vi "User Manual.vi"() -> ()   [LabVIEW 2019]
uses:
  <userlib>/Exaprom PDF/Controls/Page Controls/Page setup.ctl
  <userlib>/Exaprom PDF/Controls/Page Controls/Page size.ctl
  <userlib>/Exaprom PDF/Controls/Page Controls/Page Orientation.ctl
  <userlib>/Exaprom PDF/Controls/Page Controls/Page Layout Custom.ctl
  <userlib>/Exaprom PDF/Controls/Page Controls/Page margins.ctl
  <userlib>/Exaprom PDF/Controls/Font Controls/Font complete cluster.ctl
  <userlib>/Exaprom PDF/Controls/Font Controls/Font size.ctl
  <userlib>/Exaprom PDF/Controls/Font Controls/Font color.ctl
  <userlib>/Exaprom PDF/Controls/Font Controls/Type and encoding.ctl
  <userlib>/Exaprom PDF/Controls/Text Controls/Unicode/Type and run direction.ctl
  <userlib>/Exaprom PDF/Controls/Initialization Controls/Defaut Paragraphe and Line Spacing.ctl
  <userlib>/Exaprom PDF/Controls/Text Controls/Texte alignement.ctl
  <userlib>/Exaprom PDF/Controls/Text Controls/Line spacing.ctl
  <userlib>/Exaprom PDF/Controls/Table Controls/Table properties.ctl
  <userlib>/Exaprom PDF/Controls/Table Controls/Table position.ctl
  <userlib>/Exaprom PDF/Controls/Initialization Controls/PDF Details.ctl
  <userlib>/Exaprom PDF/Controls/Header, Footer and Watermark Controls/Header or Footer  Image cluster.ctl
  <userlib>/Exaprom PDF/Controls/Table Controls/Cell Alignment 20px.ctl
  <userlib>/Exaprom PDF/Controls/Header, Footer and Watermark Controls/Header or Footer  Page # cluster.ctl
  <userlib>/Exaprom PDF/Controls/Header, Footer and Watermark Controls/Page number.ctl
  <userlib>/Exaprom PDF/Controls/Font Controls/Font complete cluster horizontal.ctl
  <userlib>/Exaprom PDF/Controls/Header, Footer and Watermark Controls/Header or Footer Line cluster.ctl
  <userlib>/Exaprom PDF/Controls/Header, Footer and Watermark Controls/Header Footer Line.ctl
  <userlib>/Exaprom PDF/Controls/Header, Footer and Watermark Controls/Header or Footer  Text cluster.ctl
  <userlib>/Exaprom PDF/Controls/Initialization Controls/Captions.ctl
  <userlib>/Exaprom PDF/Controls/Initialization Controls/Image or Table Caption.ctl
  <userlib>/Exaprom PDF/Controls/Initialization Controls/Unit.ctl
  <userlib>/Exaprom PDF/Controls/Text Controls/Text and hyperlink [ ].ctl
  <userlib>/Exaprom PDF/Controls/Text Controls/Text from String of File and hyperlink.ctl
  <userlib>/Exaprom PDF/Controls/Text Controls/Paragraph indentation.ctl
  <userlib>/Exaprom PDF/Controls/Image Controls/Image alignment and position.ctl
  <userlib>/Exaprom PDF/Controls/Image Controls/Image aligment.ctl
  <userlib>/Exaprom PDF/Controls/Image Controls/Image border.ctl
  <userlib>/Exaprom PDF/Controls/Table Controls/Row Predefined borders cluster.ctl
  <userlib>/Exaprom PDF/Controls/Table Controls/Row Predefined borders.ctl
  <userlib>/Exaprom PDF/Controls/Image Controls/Image Scale.ctl
  <userlib>/Exaprom PDF/Controls/Table Controls/Cell Font, type, Alignment and LS V2.ctl
  <userlib>/Exaprom PDF/Controls/Table Controls/Cell Type, Alignment and LS.ctl
  <userlib>/Exaprom PDF/Controls/Table Controls/Text vertical arrangement.ctl
  <userlib>/Exaprom PDF/Controls/Table Controls/Row Back Ground color Datas.ctl
  <userlib>/Exaprom PDF/Controls/Header, Footer and Watermark Controls/Watermark Text Cluster.ctl
  <userlib>/Exaprom PDF/Controls/Header, Footer and Watermark Controls/Watermark Position.ctl
  <userlib>/Exaprom PDF/Controls/Header, Footer and Watermark Controls/Header footer horiz alignment.ctl
  <userlib>/Exaprom PDF/Controls/Header, Footer and Watermark Controls/Watermark Image Cluster.ctl
  <userlib>/Exaprom PDF/Controls/Table Controls/Simplified Table Row Borders [ ].ctl
  <userlib>/Exaprom PDF/Controls/Table Controls/Simplified Table Row Borders.ctl
  <userlib>/Exaprom PDF/Controls/Table Controls/Border and BG Color [ ].ctl
  <userlib>/Exaprom PDF/Controls/Table Controls/Border and BG Color.ctl
  <userlib>/Exaprom PDF/Controls/Table Controls/Cell Border 20 px.ctl
  <userlib>/Exaprom PDF/Controls/Concatenate Controls/PDF file to concatenate.ctl
  <userlib>/Exaprom PDF/Controls/Table Controls/Table Appearance and Font Row [ ].ctl
  <userlib>/Exaprom PDF/Controls/Table Controls/One Row Appearance.ctl
  <userlib>/Exaprom PDF/Controls/Table Controls/Row from to.ctl
  <userlib>/Exaprom PDF/Controls/Table Controls/Cell, Alignment, LS and Font - hide Vmerge.ctl
  <userlib>/Exaprom PDF/Controls/Table Controls/Cell Appearance.ctl
  <userlib>/Exaprom PDF/Controls/Table Controls/Merge Horizontal.ctl
  <userlib>/Exaprom PDF/Controls/Table Controls/Merge Vertical.ctl
  <userlib>/Exaprom PDF/Controls/Initialization Controls/File Permission Parameters.ctl
  <userlib>/Exaprom PDF/Controls/Initialization Controls/At the opening.ctl
  <vilib>/Utility/miscctls.llb/LVPointTypeDef.ctl
  <userlib>/Exaprom PDF/Controls/Header, Footer and Watermark Controls/Header or Footer.ctl
  <userlib>/Exaprom PDF/Controls/Chapter Controls/Chapter.ctl
  <userlib>/Exaprom PDF/Controls/Image Controls/Image Size Block Diagram.ctl
  <userlib>/Exaprom PDF/VIs/Low level/Header, Footer and Watermark Low level/Append Text HF.vi
  <userlib>/Exaprom PDF/VIs/Low level/Header, Footer and Watermark Low level/AppendLine seperator.vi
  <userlib>/Exaprom PDF/VIs/Low level/Header, Footer and Watermark Low level/Append Image HF.vi
  <userlib>/Exaprom PDF/VIs/Low level/Header, Footer and Watermark Low level/Append Page number HF.vi
  <userlib>/Exaprom PDF/VIs/Low level/Header, Footer and Watermark Low level/Append Watermark Image.vi
  <userlib>/Exaprom PDF/VIs/Low level/Header, Footer and Watermark Low level/Append Watermark Text.vi
  <userlib>/Exaprom PDF/VIs/Text/Append Paragraph with Link [ ].vi
  <userlib>/Exaprom PDF/VIs/Text/Append Paragraph.vi
  <userlib>/Exaprom PDF/VIs/Text/Append Phrase.vi
  <userlib>/Exaprom PDF/LV Class/PDF Report Class/PDF Report Class.lvclass
panel:
  out "Tab Control":T1(tab)
  in  "Page Setup":T2={"Page Size"=1, "Orientation"=enum."Portrait", "Custom Size"={"Width"=0.0, "Height"=0.0}, "Margins"={"Left"=1.0, "Right"=1.0, "Top"=1.0, "Bottom"=1.0}} {"Page Size" items=["Custom", "LETTER", "NOTE", "LEGAL", "TABLOID", "EXECUTIVE", "POSTCARD", "A0", "A1", "A2", "A3", "A4", "A5", "A6", "A7", "A8", "A9", "A10", "B0", "B1", "B2", "B3", "B4", "B5", "B6", "B7", "B8", "B9", "B10", "ARCH_E", "ARCH_D", "ARCH_C", "ARCH_B", "ARCH_A", "FLSA", "FLSE", "HALFLETTER", "_11X17", "ID_1", "ID_2", "ID_3", "LEDGER", "CROWN_QUARTO", "LARGE_CROWN_QUARTO", "DEMY_QUARTO", "ROYAL_QUARTO", "CROWN_OCTAVO", "LARGE_CROWN_OCTAVO", "DEMY_OCTAVO", "ROYAL_OCTAVO", "SMALL_PAPERBACK", "PENGUIN_SMALL_PAPERBACK", "PENGUIN_LARGE_PAPERBACK"]}
  in  "Default Paragraph":T7={" Aligment"=enum."JUSTIFY", "Line spacing"=enum."1.0"}
  out "error out":errorcluster
  in  "PDF Details":T10={"Title"="User Manual for Exaprom PDF 2.0", "Author"="Jean-Marc Simard", "Subject"="This example shows how to create a PDF Report with the toolkit Exaprom PDF 2.0.", "Keywords"="", "Creator"="Exaprom PDF 2.0"}
  in  "File or Directory path":path=path "C:/Users/Jean-Marc/Documents/User Manual.pdf"
  out "PDF File Name":path=path "C:/Users/Jean-Marc/Documents/User Manual.pdf"
  in  "Default Font":T11={"Name"="Arial", "Size"=12.0, "Color"=0, "Style"={"Bold"=FALSE, "Italic"=FALSE, "Underline"=FALSE, "Strikeout"=FALSE}, "Type"={"Type&direction"=enum."ASCII", "Embedded"=FALSE, "Encoding"="CP1252"}}
  in  "Captions":T16={"Figure"={"Caption"="Figure ", "Separator"=":  ", "Position"=enum."Below"}, "Table"={"Caption"="Table ", "Separator"=":  ", "Position"=enum."Above"}, "Font"={"Name"="", "Size"=-1.0, "Color"=0, "Style"={"Bold"=FALSE, "Italic"=FALSE, "Underline"=FALSE, "Strikeout"=FALSE}, "Type"={"Type&direction"=enum."Select", "Embedded"=FALSE, "Encoding"=""}}}
  in  "Unit (default = mm)":T18
  in  "Overwrite?":bool=TRUE
  out "Progress":u8(slide) scale=0.0..20.0
  in  "Permissions":T19={"User Password"="", "Owner Password"="", "Printing"=enum."Allow Printing", "Allow Modify Contents"=FALSE, "Allow Copy"=TRUE, "Allow Modify Annotations"=FALSE, "Allow Fill In "=FALSE, "Allow Screen Readers"=FALSE, "Allow Assembly"=FALSE}
  in  "At the opening":T20={"Page"=1, "Show Bookmarks"=TRUE} {"Page" items=["Single Page - Fit Page"=1, "Single Page - Fit Width"=0]}
  in  "Watermark":enum16{"none", "Image", "Text"}(ring)=enum."Text"
  in  "Footer Page #":T21={"Start at page"=3, "Start with #"=1, "Cell Alignment"=6, "Page #"={"Text 1"="!\u0004B\u0004@\u00040\u0004=\u00048\u0004F\u00040\u0004", "Text 2"="8\u00047\u0004", "Text 3"=""}, "Font"={"Name"="Arial Unicode MS", "Size"=10.0, "Color"=0, "Style"={"Bold"=FALSE, "Italic"=FALSE, "Underline"=FALSE, "Strikeout"=FALSE}, "Type"={"Type&direction"=enum."UTF-16", "Embedded"=FALSE, "Encoding"="CP1251"}}}
  in  "Footer Line":T25={"H/F Line"=enum."Horizontal line", "Thickness (point)"=0.75, " Colour"=7171459}
  in  "Header Line":T25={"H/F Line"=enum."Horizontal line", "Thickness (point)"=0.75, " Colour"=7171459}
  in  "Header Text":T27={"Start at page"=3, "Cell Alignment"=5, "Line spacing"=enum."Select", "Text"="Exaprom PDF 2.0 Toolkit for LabVIEW\n(with <a>iTextSharp</a> 4.1.6)", "Font complete"={"Name"="", "Size"=14.0, "Color"=0, "Style"={"Bold"=TRUE, "Italic"=FALSE, "Underline"=FALSE, "Strikeout"=FALSE}, "Type"={"Type&direction"=enum."Select", "Embedded"=FALSE, "Encoding"=""}}, "Link"="http://itextpdf.com/"}
  in  "Footer Text":T27={"Start at page"=3, "Cell Alignment"=4, "Line spacing"=enum."Select", "Text"="This is an example for the fonts (Segoe Script).", "Font complete"={"Name"="Segoe Script", "Size"=8.0, "Color"=16711680, "Style"={"Bold"=TRUE, "Italic"=TRUE, "Underline"=FALSE, "Strikeout"=FALSE}, "Type"={"Type&direction"=enum."Select", "Embedded"=FALSE, "Encoding"=""}}, "Link"="http://www.microsoft.com/typography/fonts/family.aspx?FID=353"}
  in  "Watermark Image":T28={"Image path"=path "C:/Program Files (x86)/National Instruments/LabVIEW 2013/vi.lib/Exaprom PDF/Examples/Images/Logo Exaprom.jpg", "Opacity (%)"=10.0, "Postion"={"Position"=enum."Center (text section)", "X"=0.0, "Y"=0.0}, "Automatic"=TRUE, "Scale(%)"=100.0, "Rotate(°)"=0.0}
  in  "Watermark Text":T30={"Text "="DRAFT", "Opacity (%)"=5.0, "Position"={"Position"=enum."Center (text section)", "X"=0.0, "Y"=0.0}, "Automatic"=TRUE, "Font"={"Font Name"="", "Size"=-1.0, "Color"=0}, "Alignment"=enum."Center", "Rotate(°)"=0.0}
  in  "Footer Image":T32={"Start at page"=3, "Cell Alignment"=5, "Path"=path "C:/Program Files (x86)/National Instruments/LabVIEW 2013/vi.lib/Exaprom PDF/Examples/Images/Logo Exaprom.jpg", "Image (%)"=15.0, "Link"="http://www.exaprom.com/"}
  in  "Text FP1 [ ]":T33=[{"Text"={"Text"="\n\nExaprom PDF 2.0 Toolkit\n\nUser Manual\n\n", "Path"=path "", "Font complete"={"Name"="", "Size"=32.0, "Color"=0, "Style"={"Bold"=TRUE, "Italic"=FALSE, "Underline"=FALSE, "Strikeout"=FALSE}, "Type"={"Type&direction"=enum."ASCII", "Embedded"=FALSE, "Encoding"=""}}}, "Link"={"Hyperlink"="", "Font complete"={"Name"="", "Size"=-1.0, "Color"=255, "Style"={"Bold"=FALSE, "Italic"=TRUE, "Underline"=FALSE, "Strikeout"=FALSE}, "Type"={"Type&direction"=enum."Select", "Embedded"=FALSE, "Encoding"=""}}}, "Paragraphe"={" Aligment"=enum."CENTER", "Line spacing"=enum."Select"}, "Indentation"={"Left"=0.0, "Right"=0.0}}, {"Text"={"Text"="\nPDF Report with iTextSharp 4.1.6\nfor LabVIEW", "Path"=path "", "Font complete"={"Name"="", "Size"=24.0, "Color"=0, "Style"={"Bold"=TRUE, "Italic"=FALSE, "Underline"=FALSE, "Strikeout"=FALSE}, "Type"={"Type&direction"=enum."Select", "Embedded"=FALSE, "Encoding"=""}}}, "Link"={"Hyperlink"="", "Font complete"={"Name"="", "Size"=-1.0, "Color"=255, "Style"={"Bold"=FALSE, "Italic"=TRUE, "Underline"=FALSE, "Strikeout"=FALSE}, "Type"={"Type&direction"=enum."Select", "Embedded"=FALSE, "Encoding"=""}}}, "Paragraphe"={" Aligment"=enum."CENTER", "Line spacing"=enum."Select"}, "Indentation"={"Left"=0.0, "Right"=0.0}}, {"Text"={"Text"="\n\n\n\nby\n\nJean-Marc Simard\n\n\n\nDevember 10, 2013", "Path"=path "", "Font complete"={"Name"="", "Size"=24.0, "Color"=0, "Style"={"Bold"=FALSE, "Italic"=FALSE, "Underline"=FALSE, "Strikeout"=FALSE}, "Type"={"Type&direction"=enum."Select", "Embedded"=FALSE, "Encoding"=""}}}, "Link"={"Hyperlink"="", "Font complete"={"Name"="", "Size"=-1.0, "Color"=255, "Style"={"Bold"=FALSE, "Italic"=TRUE, "Underline"=FALSE, "Strikeout"=FALSE}, "Type"={"Type&direction"=enum."Select", "Embedded"=FALSE, "Encoding"=""}}}, "Paragraphe"={" Aligment"=enum."CENTER", "Line spacing"=enum."Select"}, "Indentation"={"Left"=0.0, "Right"=0.0}}]
  in  "Image FP1":path=path "C:/Program Files/National Instruments/LabVIEW 2009/vi.lib/Exaprom PDF/Examples/Images/Logo Exaprom.jpg"
  in  "TOC Title":string="\nTable of Contents\n\n\n"
  in  "TOC Title Font":T11={"Name"="Arial Unicode MS", "Size"=14.0, "Color"=0, "Style"={"Bold"=TRUE, "Italic"=FALSE, "Underline"=FALSE, "Strikeout"=FALSE}, "Type"={"Type&direction"=enum."ASCII", "Embedded"=FALSE, "Encoding"="CP1252"}}
  in  "TOC Chapter and section Font":T11={"Name"="Arial Unicode MS", "Size"=-1.0, "Color"=0, "Style"={"Bold"=FALSE, "Italic"=FALSE, "Underline"=FALSE, "Strikeout"=FALSE}, "Type"={"Type&direction"=enum."UTF-16", "Embedded"=FALSE, "Encoding"="CP1251"}}
  in  "Text C8":string="\nAlthough this toolkit had not intended to replace a word processor, we have produced this document, as an example, with this PDF toolkit . The VI \"User Manual.vi\" is available in the palette \"Exaprom PDF 2.0\"."
  in  "Texte C2 [ ]":T33=[{"Text"={"Text"="\nI developed this Reports generation toolkit for PDF because I wanted to be able to generate PDF reports, on LabVIEW, without having to buy a license. The choice fell on the open source iTextSharp 4.1.6 library (<a>Mozilla Public License Version 1.1</a>).  I have developed a series of VIs allowing me to generate PDF reports directly without having to purchase a commercial product. The license chosen:\n", "Path"=path "", "Font complete"={"Name"="", "Size"=-1.0, "Color"=0, "Style"={"Bold"=FALSE, "Italic"=FALSE, "Underline"=FALSE, "Strikeout"=FALSE}, "Type"={"Type&direction"=enum."Select", "Embedded"=FALSE, "Encoding"=""}}}, "Link"={"Hyperlink"="http://www.mozilla.org/MPL/MPL-1.1.html", "Font complete"={"Name"="", "Size"=-1.0, "Color"=255, "Style"={"Bold"=FALSE, "Italic"=TRUE, "Underline"=FALSE, "Strikeout"=FALSE}, "Type"={"Type&direction"=enum."Select", "Embedded"=FALSE, "Encoding"=""}}}, "Paragraphe"={" Aligment"=enum."Select", "Line spacing"=enum."Select"}, "Indentation"={"Left"=0.0, "Right"=0.0}}, {"Text"={"Text"="\n\"The <a>BSD (Berkeley software distribution license)</a> allows proprietary use, and for the software released under the license to be incorporated into proprietary products. Works based on the material may be released under a proprietary license or as closed source software.\" \n", "Path"=path "", "Font complete"={"Name"="", "Size"=-1.0, "Color"=0, "Style"={"Bold"=FALSE, "Italic"=FALSE, "Underline"=FALSE, "Strikeout"=FALSE}, "Type"={"Type&direction"=enum."Select", "Embedded"=FALSE, "Encoding"=""}}}, "Link"={"Hyperlink"="http://fr.wikipedia.org/wiki/Licence_BSD", "Font complete"={"Name"="", "Size"=-1.0, "Color"=255, "Style"={"Bold"=FALSE, "Italic"=TRUE, "Underline"=FALSE, "Strikeout"=FALSE}, "Type"={"Type&direction"=enum."Select", "Embedded"=FALSE, "Encoding"=""}}}, "Paragraphe"={" Aligment"=enum."Select", "Line spacing"=enum."Select"}, "Indentation"={"Left"=0.5, "Right"=0.5}}, {"Text"={"Text"="\nRoughly, you do what you want with those VIs.\n\nThe newer version, <a>iTextSharp 5.X</a>, is under Affero General Public License and is not free for activities involving the iText software without disclosing the source code of your own applications.\n\n\n", "Path"=path "", "Font complete"={"Name"="", "Size"=-1.0, "Color"=0, "Style"={"Bold"=FALSE, "Italic"=FALSE, "Underline"=FALSE, "Strikeout"=FALSE}, "Type"={"Type&direction"=enum."Select", "Embedded"=FALSE, "Encoding"=""}}}, "Link"={"Hyperlink"="http://itextpdf.com/terms-of-use/", "Font complete"={"Name"="", "Size"=-1.0, "Color"=255, "Style"={"Bold"=FALSE, "Italic"=TRUE, "Underline"=FALSE, "Strikeout"=FALSE}, "Type"={"Type&direction"=enum."Select", "Embedded"=FALSE, "Encoding"=""}}}, "Paragraphe"={" Aligment"=enum."Select", "Line spacing"=enum."Select"}, "Indentation"={"Left"=0.0, "Right"=0.0}}]
  in  "Texte D2 [ ]":T33=[{"Text"={"Text"="\n\nThe production of a PDF report can be divided into four steps:\n\n     1) Creating a report (PDF file and default parameters)\n     2) Adding header, footer and watermark (all optional)\n     3) Writing of the PDF report which involves the addition of text elements, images (file,\n           control and front panel) and tables;\n     4) The closure of the PDF report.\n\nIn chapter 5, we review the different VI needed to create a PDF report.\n\n", "Path"=path "", "Font complete"={"Name"="", "Size"=-1.0, "Color"=0, "Style"={"Bold"=FALSE, "Italic"=FALSE, "Underline"=FALSE, "Strikeout"=FALSE}, "Type"={"Type&direction"=enum."Select", "Embedded"=FALSE, "Encoding"=""}}}, "Link"={"Hyperlink"="", "Font complete"={"Name"="", "Size"=-1.0, "Color"=255, "Style"={"Bold"=FALSE, "Italic"=TRUE, "Underline"=FALSE, "Strikeout"=FALSE}, "Type"={"Type&direction"=enum."Select", "Embedded"=FALSE, "Encoding"=""}}}, "Paragraphe"={" Aligment"=enum."Select", "Line spacing"=enum."Select"}, "Indentation"={"Left"=0.0, "Right"=0.0}}]
  in  "Text C6":string="After restart LabVIEW, the palette \"Exaprom PDF 2.0\" will appears.\n\n"
  in  "Text C1":string="Introduction"
  in  "Text C3":string="Installation"
  in  "Texte C4 [ ]":T33=[{"Text"={"Text"="\nAfter unzipping \"ExapromPDF2.0.ZIP\", you have a folder and a file:\n\n     1)\tthe folder \"Exaprom PDF\";\n     2)\tand the file \"exaprompdf.mnu\".\n\n\n", "Path"=path "", "Font complete"={"Name"="", "Size"=-1.0, "Color"=0, "Style"={"Bold"=FALSE, "Italic"=FALSE, "Underline"=FALSE, "Strikeout"=FALSE}, "Type"={"Type&direction"=enum."Select", "Embedded"=FALSE, "Encoding"=""}}}, "Link"={"Hyperlink"="", "Font complete"={"Name"="", "Size"=-1.0, "Color"=16777222, "Style"={"Bold"=TRUE, "Italic"=FALSE, "Underline"=FALSE, "Strikeout"=FALSE}, "Type"={"Type&direction"=enum."Select", "Embedded"=FALSE, "Encoding"=""}}}, "Paragraphe"={" Aligment"=enum."LEFT", "Line spacing"=enum."Select"}, "Indentation"={"Left"=0.0, "Right"=0.0}}]
  in  "Text C5":string="\n\nThe folder \"Exaprom PDF\" has to be place in (see figure 2):\n\nC:\\Program Files\\National Instruments\\LabVIEW Version\\vi.lib\\\n\n"
  in  "Text C7":string="\nThe file \"exaprompdf.mnu\" have to be place in (see figure 3):\n\nC:\\Program Files\\National Instruments\\LabVIEW Version\\\n                                                                                     menus\\Categories\\Programming\\"
  in  "Text D1":string="PDF Report (simplified)"
  in  "Texte E2 [ ]":T33=[{"Text"={"Text"="\n\nThe library used to generate PDF reports is iTextSharp. \n\nThis library uses the point  (72 points = 1 inch = 25.4 mm), but you will work with the unit you choose (inch or mm - section 5.4) unless  the unit \"point\" is clearly indicated.  The font is an exception: the unit is the point.\n\nThe origin of the page is the bottom left corner (see the figure below).\n\nThe text box is the page minus the margins (blue rectangle in the figure below).\n\n\n", "Path"=path "", "Font complete"={"Name"="", "Size"=-1.0, "Color"=0, "Style"={"Bold"=FALSE, "Italic"=FALSE, "Underline"=FALSE, "Strikeout"=FALSE}, "Type"={"Type&direction"=enum."Select", "Embedded"=FALSE, "Encoding"=""}}}, "Link"={"Hyperlink"="", "Font complete"={"Name"="", "Size"=-1.0, "Color"=255, "Style"={"Bold"=FALSE, "Italic"=TRUE, "Underline"=FALSE, "Strikeout"=FALSE}, "Type"={"Type&direction"=enum."Select", "Embedded"=FALSE, "Encoding"=""}}}, "Paragraphe"={" Aligment"=enum."Select", "Line spacing"=enum."Select"}, "Indentation"={"Left"=0.0, "Right"=0.0}}]
  in  "Text E1":string="General"
  in  "Text F2":string="The \"Text\" palette "
  in  "Text F1":string="The different palettes"
  in  "Texte F3 [ ]":T33=[{"Text"={"Text"="\n\nYou have access the fonts contained in the directory C: \\ Windows \\ Fonts (you should check the copyrights). In addition, you have the fonts that come automatically with iTextSharp: Courier, Helvetica, Symbol, Times-Roman and ZapfDingbats.\n\nWhen the PDF report was created, we have specified that the Default Font was Arial 12 points (bold, italic, underline and strikeout = F), Type&direction = ASCII and character encoding = CP1252 (Latin alphabet). This information is stored in the LV Class \"PDF Report\". The parameters of the font in all VI of the Text palette are:\n\n           - Name = empty string;\n           - Size = -1;\n           - Bold, Italic, Underline and Strikeout = F;\n           - Type&direction = Select;\n           - E (Embedded) = F;\n           - Encoding = empty string.\n\nWhen the name of the font is left empty, the name of the default font is used.  When the value of the font size is -1 then the default font size is used. When the value of Type&direction is left to Select, the Type&direction of the default font is used. When the value of the Encoding is left empty, the Encoding of the default font is used.\n", "Path"=path "", "Font complete"={"Name"="", "Size"=-1.0, "Color"=0, "Style"={"Bold"=FALSE, "Italic"=FALSE, "Underline"=FALSE, "Strikeout"=FALSE}, "Type"={"Type&direction"=enum."Select", "Embedded"=FALSE, "Encoding"=""}}}, "Link"={"Hyperlink"="", "Font complete"={"Name"="", "Size"=-1.0, "Color"=255, "Style"={"Bold"=FALSE, "Italic"=TRUE, "Underline"=FALSE, "Strikeout"=FALSE}, "Type"={"Type&direction"=enum."Select", "Embedded"=FALSE, "Encoding"=""}}}, "Paragraphe"={" Aligment"=enum."Select", "Line spacing"=enum."Select"}, "Indentation"={"Left"=0.0, "Right"=0.0}}]
  in  "Text F6":string="When the PDF Report was created, we specified that the default alignment was \"JUSTIFY\" and the default line spacing was 1.0. This information is also stored in the LV Class \"PDF Report\". \n\nWhen the alignment is left to \"Select\" than the default alignment is used. When the spacing is left to \"Select\" than the default line spacing is used.\n\n"
  in  "Text F8 [ ]":T33=[{"Text"={"Text"="This tag allows you to insert the image \"Arrow.jpg\" like this <img src=\"Arrow\"/>.  To insert the image \"Logo E.jpg\" with a link <a><img src=\"Logo\"/></a> you should use \"Append Paragraph & Link [ ].vi\".  All these paragraphs are automatically terminated with a line Feed.  \n\n", "Path"=path "", "Font complete"={"Name"="", "Size"=-1.0, "Color"=0, "Style"={"Bold"=FALSE, "Italic"=FALSE, "Underline"=FALSE, "Strikeout"=FALSE}, "Type"={"Type&direction"=enum."Select", "Embedded"=FALSE, "Encoding"=""}}}, "Link"={"Hyperlink"="http://www.exaprom.com/", "Font complete"={"Name"="", "Size"=-1.0, "Color"=255, "Style"={"Bold"=FALSE, "Italic"=TRUE, "Underline"=FALSE, "Strikeout"=FALSE}, "Type"={"Type&direction"=enum."Select", "Embedded"=FALSE, "Encoding"=""}}}, "Paragraphe"={" Aligment"=enum."Select", "Line spacing"=enum."Select"}, "Indentation"={"Left"=0.0, "Right"=0.0}}, {"Text"={"Text"="The third one, \"Append Phrase.vi\" (number \"4\"), adds a phrase but without a line feed and with a left alignment.   In addition, except for \"Append Phrase.vi\", it is possible to have a paragraph indentation (left and right).\n", "Path"=path "", "Font complete"={"Name"="", "Size"=-1.0, "Color"=0, "Style"={"Bold"=FALSE, "Italic"=FALSE, "Underline"=FALSE, "Strikeout"=FALSE}, "Type"={"Type&direction"=enum."Select", "Embedded"=FALSE, "Encoding"=""}}}, "Link"={"Hyperlink"="", "Font complete"={"Name"="", "Size"=-1.0, "Color"=255, "Style"={"Bold"=FALSE, "Italic"=TRUE, "Underline"=FALSE, "Strikeout"=FALSE}, "Type"={"Type&direction"=enum."Select", "Embedded"=FALSE, "Encoding"=""}}}, "Paragraphe"={" Aligment"=enum."Select", "Line spacing"=enum."Select"}, "Indentation"={"Left"=0.0, "Right"=0.0}}]
  in  "Text F7":string="There are three VIs to add text, and they are grouped in the VI \"Append Text polymorphic.vi\" (number \"1\"  in the previous figure). \n\nWith the first, \"Append Paragraph.vi\" (number \"2\"), you can add text as paragraphs and the text is automatically terminated with a line feed.\n\nThe second or \"Append Paragraph & Link [ ]. Vi\" (number \"3\"), adds a sequence of paragraphs with the particularity that it is possible to associate a link (http://www.mywebsite.com/ ou mailto:name@example.com) with the text, placed between the tags < a> </ a>. \n\nFurthermore, it is possible with \"Append Paragraph.vi\" and \"Append Paragraph & Link [ ]. Vi\" to insert images in a paragraph with the tag <img src=\"Image name\"/>.\n"
  in  "Text F5":string="\nThe character encoding can be ASCII or Unicode (UTF-16).  The writing directions (only for Unicode) are:\n\n  - UTF-16 \"UTF-16 characters, left to right writing\";\n  - UTF-16 (default) \"Use the default run direction\";\n  - UTF-16 (LTR) \"Use bidirectional reordering with a left-to-right preferential\n     run direction\";\n  - UTF-16 (RTL) \"Use bidirectional reordering with a right-to-left preferential\n     run direction\".\n\n"
  in  "Text F4":string="The cluster font could be vertical or horizontal.\n"
  in  "Text G4":string="\nThe available choices are:\n1) Absolute (X, Y) in mm;\n2) Left;\n3) Center;\n4) Right;\n5) Left (TextWrap)\n6) Right (TextWrap).\n\"Left (TextWrap)\" means the image is placed left and the text is placed to the right.  \"Right (TextWrap)\" means that the image is placed to the right, and the text is placed to the left. The indentation works only with \"TextWrap\" and it is the horizontal space that we leave between the image and the text. We can also choose to put a border to the image.\n"
  in  "Texte G3 [ ]":T33=[{"Text"={"Text"=" \nThe Image palette has 4 VIs :\n\n         1)\t\"Append Control Image.vi \";\n         2)\t\"Append Front Panel Image.vi\".\n         3)\t\"Append Block Diagram Image.vi \";\n         4)\t\"Append Image File.vi\".\n\nWe have at the following figure the controls for the properties of the image (this image has been added with \"Append Control Image.vi). We can reduce or enlarge the size of the image (Scale percent). If the image is bigger than the text zone (page size minus the margins), the size will be adjusted automatically to fit.", "Path"=path "", "Font complete"={"Name"="", "Size"=-1.0, "Color"=0, "Style"={"Bold"=FALSE, "Italic"=FALSE, "Underline"=FALSE, "Strikeout"=FALSE}, "Type"={"Type&direction"=enum."Select", "Embedded"=FALSE, "Encoding"=""}}}, "Link"={"Hyperlink"="", "Font complete"={"Name"="", "Size"=-1.0, "Color"=255, "Style"={"Bold"=FALSE, "Italic"=TRUE, "Underline"=FALSE, "Strikeout"=FALSE}, "Type"={"Type&direction"=enum."Select", "Embedded"=FALSE, "Encoding"=""}}}, "Paragraphe"={" Aligment"=enum."Select", "Line spacing"=enum."Select"}, "Indentation"={"Left"=0.0, "Right"=0.0}}, {"Text"={"Text"="\nWe can choose the horizontal position of the image, as long as we have not added a caption, because in this case, it is always centered horizontally.", "Path"=path "", "Font complete"={"Name"="", "Size"=-1.0, "Color"=0, "Style"={"Bold"=FALSE, "Italic"=FALSE, "Underline"=FALSE, "Strikeout"=FALSE}, "Type"={"Type&direction"=enum."Select", "Embedded"=FALSE, "Encoding"=""}}}, "Link"={"Hyperlink"="", "Font complete"={"Name"="", "Size"=-1.0, "Color"=255, "Style"={"Bold"=FALSE, "Italic"=TRUE, "Underline"=FALSE, "Strikeout"=FALSE}, "Type"={"Type&direction"=enum."Select", "Embedded"=FALSE, "Encoding"=""}}}, "Paragraphe"={" Aligment"=enum."Select", "Line spacing"=enum."Select"}, "Indentation"={"Left"=0.0, "Right"=0.0}}]
  in  "Texte G2 [ ]":T33=[{"Text"={"Text"="\nImages placed in the PDF can be reduced or enlarged, but it's only a matter of view: they will always occupy the same space in the PDF file.\n", "Path"=path "", "Font complete"={"Name"="", "Size"=-1.0, "Color"=0, "Style"={"Bold"=FALSE, "Italic"=FALSE, "Underline"=FALSE, "Strikeout"=FALSE}, "Type"={"Type&direction"=enum."Select", "Embedded"=FALSE, "Encoding"=""}}}, "Link"={"Hyperlink"="", "Font complete"={"Name"="", "Size"=-1.0, "Color"=255, "Style"={"Bold"=FALSE, "Italic"=TRUE, "Underline"=FALSE, "Strikeout"=FALSE}, "Type"={"Type&direction"=enum."Select", "Embedded"=FALSE, "Encoding"=""}}}, "Paragraphe"={" Aligment"=enum."Select", "Line spacing"=enum."Select"}, "Indentation"={"Left"=0.0, "Right"=0.0}}]
  in  "Text G1":string="The \"Image\" palette"
  in  "Text H3":string="To create a table, there are six variables, including five optional:\n\n               1) Table columnWidht [ ] (optional);\n               2) Repeat Headers Column (optional)\n               3) Column Headers 2D [ ] (optional);\n               4) Row Headers 1D [ ] (optional);\n               5) Text Data 2D [ ] (required);\n               6) Image to Add [ ] (optional).\n\nThe first specifies the width of each column. The second offers the possibility, if the table has more than one page, to repeat the column headers on each new page.   The third is the column headers.  The fourth is the row headers.  The fifth is the text datas while the last one  allows you to insert images in a table cell. It should be noted that a cell can contain either text or an image, but not both.\n\nThe number of columns is defined by the number of columns after \"Column Headers 2D [ ]\", \"Row Headers 1D\" and \"Text Data 2D [ ]\" are concatenated.\n\nIf the variable \"Table columnWidht [ ]\" is not wired, then the width of each column will be identical and equal to the width of the page (minus the margins) divided by the number of columns (Table 2 versus Table 3 at page 21). If the variable  \"Table columnWidht []\" has more elements than the number of columns, only the first elements will be used. If the variable \"Table columnWidht [ ]\" has fewer elements than the number of columns, columns of 25 mm will be added.\n\nIf the total width of the table is larger than the width of the text zone, then the width of each column will be proportionately reduced so that the table width equals the width of the text zone.\n\nLike for images, we can choose the horizontal position if we have not added any caption, because in this case, the table is always centered horizontally.\n"
  in  "Texte H2 [ ]":T33=[{"Text"={"Text"="\nAdding a table is done in two steps: first, create the table with \"Create Table.vi\" and then add the table with \"Append Table.vi\" or \"Append Customized Table.vi\".\n\n", "Path"=path "", "Font complete"={"Name"="", "Size"=-1.0, "Color"=0, "Style"={"Bold"=FALSE, "Italic"=FALSE, "Underline"=FALSE, "Strikeout"=FALSE}, "Type"={"Type&direction"=enum."Select", "Embedded"=FALSE, "Encoding"=""}}}, "Link"={"Hyperlink"="", "Font complete"={"Name"="", "Size"=-1.0, "Color"=255, "Style"={"Bold"=FALSE, "Italic"=TRUE, "Underline"=FALSE, "Strikeout"=FALSE}, "Type"={"Type&direction"=enum."Select", "Embedded"=FALSE, "Encoding"=""}}}, "Paragraphe"={" Aligment"=enum."Select", "Line spacing"=enum."Select"}, "Indentation"={"Left"=0.0, "Right"=0.0}}]
  in  "Text H7 [ ]":T33=[{"Text"={"Text"="The variable \"Costum Borders\", column by column, defines the type of border for each cell. In iTextSharp there are 16 options, ranging from no line to a line on all four sides. We can also define the background color of each cell.\n\nThe variable <img src=\"Row1\"/> is used to format the table, row by row. A value of -2 indicates the penultimate row. For example,  <img src=\"Row2\"/> iindicates that formatting is applied to row 0 to the penultimate row. A value of -1 indicates the last row. For example, <img src=\"Row3\"/> indicates that formatting is applied to the last row.\n\n", "Path"=path "", "Font complete"={"Name"="", "Size"=-1.0, "Color"=0, "Style"={"Bold"=FALSE, "Italic"=FALSE, "Underline"=FALSE, "Strikeout"=FALSE}, "Type"={"Type&direction"=enum."Select", "Embedded"=FALSE, "Encoding"=""}}}, "Link"={"Hyperlink"="", "Font complete"={"Name"="", "Size"=-1.0, "Color"=255, "Style"={"Bold"=FALSE, "Italic"=TRUE, "Underline"=FALSE, "Strikeout"=FALSE}, "Type"={"Type&direction"=enum."Select", "Embedded"=FALSE, "Encoding"=""}}}, "Paragraphe"={" Aligment"=enum."Select", "Line spacing"=enum."Select"}, "Indentation"={"Left"=0.0, "Right"=0.0}}]
  in  "Texte H4 [ ]":T33=[{"Text"={"Text"="\nIf the total width of the table is larger than the width of the text zone, then the width of each column will be proportionately reduced so that the table width equals the width of the text zone.\n\nLike for images, we can choose the horizontal position if we have not added any caption, because in this case, the table is always centered horizontally.\n", "Path"=path "", "Font complete"={"Name"="", "Size"=-1.0, "Color"=0, "Style"={"Bold"=FALSE, "Italic"=FALSE, "Underline"=FALSE, "Strikeout"=FALSE}, "Type"={"Type&direction"=enum."Select", "Embedded"=FALSE, "Encoding"=""}}}, "Link"={"Hyperlink"="", "Font complete"={"Name"="", "Size"=-1.0, "Color"=255, "Style"={"Bold"=FALSE, "Italic"=TRUE, "Underline"=FALSE, "Strikeout"=FALSE}, "Type"={"Type&direction"=enum."Select", "Embedded"=FALSE, "Encoding"=""}}}, "Paragraphe"={" Aligment"=enum."Select", "Line spacing"=enum."Select"}, "Indentation"={"Left"=0.0, "Right"=0.0}}, {"Text"={"Text"="\nThe final table generated with \"Column Headers 2D [ ]\", \"Row Headers 1D [ ]\" and \"Text Data 2D [ ]\" appears at the following figure.\n\n", "Path"=path "", "Font complete"={"Name"="", "Size"=-1.0, "Color"=0, "Style"={"Bold"=FALSE, "Italic"=FALSE, "Underline"=FALSE, "Strikeout"=FALSE}, "Type"={"Type&direction"=enum."Select", "Embedded"=FALSE, "Encoding"=""}}}, "Link"={"Hyperlink"="", "Font complete"={"Name"="", "Size"=-1.0, "Color"=255, "Style"={"Bold"=FALSE, "Italic"=TRUE, "Underline"=FALSE, "Strikeout"=FALSE}, "Type"={"Type&direction"=enum."Select", "Embedded"=FALSE, "Encoding"=""}}}, "Paragraphe"={" Aligment"=enum."Select", "Line spacing"=enum."Select"}, "Indentation"={"Left"=0.0, "Right"=0.0}}]
  in  "Text H8":string="We can also append a table with \"Append Customized Table.vi\". It is not really intuitive, but you have more flexibility like horizontal merging (see table 5).\n\n"
  in  "Text H5":string="When we add the table to the document with \"Append Table.vi\" we have , if we exclude \"PDF Table\", eight variables (all optional):\n               1) Row background color\n               2) Predefined Borders;\n               3) Column Header Format;\n               4) Table properties;\n               5) Caption;\n               6) Row Header Format;\n               7) Datas Format;\n               8) Custom Table Borders.\n\nThe first offer the possibility to add a background color at each X row.  The second offers a choice for types of borders available: predefined and custom. If the custom type is chosen, then it must use the variable \"Custom Table Borders\" to define the borders of table cells.\n\n"
  in  "Text H6":string="The third, the sixth and the seventh are the cell format for the column headers, the row headers and the data respectively."
  in  "Text H1":string="The \"Table\" palette"
  in  "Texte I6 [ ]":T33=[{"Text"={"Text"="\n ix) the opening of the PDF file generated\n\nHow the PDF file will open.\n\n", "Path"=path "", "Font complete"={"Name"="", "Size"=-1.0, "Color"=0, "Style"={"Bold"=FALSE, "Italic"=FALSE, "Underline"=FALSE, "Strikeout"=FALSE}, "Type"={"Type&direction"=enum."Select", "Embedded"=FALSE, "Encoding"=""}}}, "Link"={"Hyperlink"="", "Font complete"={"Name"="", "Size"=-1.0, "Color"=255, "Style"={"Bold"=FALSE, "Italic"=TRUE, "Underline"=FALSE, "Strikeout"=FALSE}, "Type"={"Type&direction"=enum."Select", "Embedded"=FALSE, "Encoding"=""}}}, "Paragraphe"={" Aligment"=enum."Select", "Line spacing"=enum."Select"}, "Indentation"={"Left"=0.0, "Right"=0.0}}, {"Text"={"Text"="b) Closing the PDF report with \"Close PDF.vi\"", "Path"=path "", "Font complete"={"Name"="", "Size"=-1.0, "Color"=0, "Style"={"Bold"=TRUE, "Italic"=FALSE, "Underline"=FALSE, "Strikeout"=FALSE}, "Type"={"Type&direction"=enum."Select", "Embedded"=FALSE, "Encoding"=""}}}, "Link"={"Hyperlink"="", "Font complete"={"Name"="", "Size"=-1.0, "Color"=255, "Style"={"Bold"=FALSE, "Italic"=TRUE, "Underline"=FALSE, "Strikeout"=FALSE}, "Type"={"Type&direction"=enum."Select", "Embedded"=FALSE, "Encoding"=""}}}, "Paragraphe"={" Aligment"=enum."Select", "Line spacing"=enum."Select"}, "Indentation"={"Left"=0.0, "Right"=0.0}}, {"Text"={"Text"="\nThis VI is used to complete the writing of the report PDF. He closes various references needed to write a PDF file, it writes the header, footer and watermark (if needed) and closes the PDF.\n\n", "Path"=path "", "Font complete"={"Name"="", "Size"=-1.0, "Color"=0, "Style"={"Bold"=FALSE, "Italic"=FALSE, "Underline"=FALSE, "Strikeout"=FALSE}, "Type"={"Type&direction"=enum."Select", "Embedded"=FALSE, "Encoding"=""}}}, "Link"={"Hyperlink"="", "Font complete"={"Name"="", "Size"=-1.0, "Color"=255, "Style"={"Bold"=FALSE, "Italic"=TRUE, "Underline"=FALSE, "Strikeout"=FALSE}, "Type"={"Type&direction"=enum."Select", "Embedded"=FALSE, "Encoding"=""}}}, "Paragraphe"={" Aligment"=enum."Select", "Line spacing"=enum."Select"}, "Indentation"={"Left"=0.0, "Right"=0.0}}, {"Text"={"Text"="c) Adding a page break with \"Append New Page.vi\"", "Path"=path "", "Font complete"={"Name"="", "Size"=-1.0, "Color"=0, "Style"={"Bold"=TRUE, "Italic"=FALSE, "Underline"=FALSE, "Strikeout"=FALSE}, "Type"={"Type&direction"=enum."Select", "Embedded"=FALSE, "Encoding"=""}}}, "Link"={"Hyperlink"="", "Font complete"={"Name"="", "Size"=-1.0, "Color"=255, "Style"={"Bold"=FALSE, "Italic"=TRUE, "Underline"=FALSE, "Strikeout"=FALSE}, "Type"={"Type&direction"=enum."Select", "Embedded"=FALSE, "Encoding"=""}}}, "Paragraphe"={" Aligment"=enum."Select", "Line spacing"=enum."Select"}, "Indentation"={"Left"=0.0, "Right"=0.0}}, {"Text"={"Text"="\nThis VI adds a page break in PDF document.\n\n", "Path"=path "", "Font complete"={"Name"="", "Size"=-1.0, "Color"=0, "Style"={"Bold"=FALSE, "Italic"=FALSE, "Underline"=FALSE, "Strikeout"=FALSE}, "Type"={"Type&direction"=enum."Select", "Embedded"=FALSE, "Encoding"=""}}}, "Link"={"Hyperlink"="", "Font complete"={"Name"="", "Size"=-1.0, "Color"=255, "Style"={"Bold"=FALSE, "Italic"=TRUE, "Underline"=FALSE, "Strikeout"=FALSE}, "Type"={"Type&direction"=enum."Select", "Embedded"=FALSE, "Encoding"=""}}}, "Paragraphe"={" Aligment"=enum."Select", "Line spacing"=enum."Select"}, "Indentation"={"Left"=0.0, "Right"=0.0}}, {"Text"={"Text"="d) Adding a section break (new page) by changing the properties of the page with \"Page Set Size.vi\"", "Path"=path "", "Font complete"={"Name"="", "Size"=-1.0, "Color"=0, "Style"={"Bold"=TRUE, "Italic"=FALSE, "Underline"=FALSE, "Strikeout"=FALSE}, "Type"={"Type&direction"=enum."Select", "Embedded"=FALSE, "Encoding"=""}}}, "Link"={"Hyperlink"="", "Font complete"={"Name"="", "Size"=-1.0, "Color"=255, "Style"={"Bold"=FALSE, "Italic"=TRUE, "Underline"=FALSE, "Strikeout"=FALSE}, "Type"={"Type&direction"=enum."Select", "Embedded"=FALSE, "Encoding"=""}}}, "Paragraphe"={" Aligment"=enum."Select", "Line spacing"=enum."Select"}, "Indentation"={"Left"=0.0, "Right"=0.0}}, {"Text"={"Text"="\nThis VI adds a page break in PDF document and can change the properties of the new page. These new properties apply to all new pages as long you will  not use \"Set Page Size.vi.\n\n", "Path"=path "", "Font complete"={"Name"="", "Size"=-1.0, "Color"=0, "Style"={"Bold"=FALSE, "Italic"=FALSE, "Underline"=FALSE, "Strikeout"=FALSE}, "Type"={"Type&direction"=enum."Select", "Embedded"=FALSE, "Encoding"=""}}}, "Link"={"Hyperlink"="", "Font complete"={"Name"="", "Size"=-1.0, "Color"=255, "Style"={"Bold"=FALSE, "Italic"=TRUE, "Underline"=FALSE, "Strikeout"=FALSE}, "Type"={"Type&direction"=enum."Select", "Embedded"=FALSE, "Encoding"=""}}}, "Paragraphe"={" Aligment"=enum."Select", "Line spacing"=enum."Select"}, "Indentation"={"Left"=0.0, "Right"=0.0}}, {"Text"={"Text"="e) Change the default font with \"Set Default Font.vi\"", "Path"=path "", "Font complete"={"Name"="", "Size"=-1.0, "Color"=0, "Style"={"Bold"=TRUE, "Italic"=FALSE, "Underline"=FALSE, "Strikeout"=FALSE}, "Type"={"Type&direction"=enum."Select", "Embedded"=FALSE, "Encoding"=""}}}, "Link"={"Hyperlink"="", "Font complete"={"Name"="", "Size"=-1.0, "Color"=255, "Style"={"Bold"=FALSE, "Italic"=TRUE, "Underline"=FALSE, "Strikeout"=FALSE}, "Type"={"Type&direction"=enum."Select", "Embedded"=FALSE, "Encoding"=""}}}, "Paragraphe"={" Aligment"=enum."Select", "Line spacing"=enum."Select"}, "Indentation"={"Left"=0.0, "Right"=0.0}}, {"Text"={"Text"="\nThis VI changes the default font.\n\n", "Path"=path "", "Font complete"={"Name"="", "Size"=-1.0, "Color"=0, "Style"={"Bold"=FALSE, "Italic"=FALSE, "Underline"=FALSE, "Strikeout"=FALSE}, "Type"={"Type&direction"=enum."Select", "Embedded"=FALSE, "Encoding"=""}}}, "Link"={"Hyperlink"="", "Font complete"={"Name"="", "Size"=-1.0, "Color"=255, "Style"={"Bold"=FALSE, "Italic"=TRUE, "Underline"=FALSE, "Strikeout"=FALSE}, "Type"={"Type&direction"=enum."Select", "Embedded"=FALSE, "Encoding"=""}}}, "Paragraphe"={" Aligment"=enum."Select", "Line spacing"=enum."Select"}, "Indentation"={"Left"=0.0, "Right"=0.0}}, {"Text"={"Text"="f) Printing of the PDF report with \"Print PDF.vi\"\n", "Path"=path "", "Font complete"={"Name"="", "Size"=-1.0, "Color"=0, "Style"={"Bold"=TRUE, "Italic"=FALSE, "Underline"=FALSE, "Strikeout"=FALSE}, "Type"={"Type&direction"=enum."Select", "Embedded"=FALSE, "Encoding"=""}}}, "Link"={"Hyperlink"="", "Font complete"={"Name"="", "Size"=-1.0, "Color"=255, "Style"={"Bold"=FALSE, "Italic"=TRUE, "Underline"=FALSE, "Strikeout"=FALSE}, "Type"={"Type&direction"=enum."Select", "Embedded"=FALSE, "Encoding"=""}}}, "Paragraphe"={" Aligment"=enum."Select", "Line spacing"=enum."Select"}, "Indentation"={"Left"=0.0, "Right"=0.0}}, {"Text"={"Text"="\nThis VI is not based on the iTextSharp library.\n\n", "Path"=path "", "Font complete"={"Name"="", "Size"=-1.0, "Color"=0, "Style"={"Bold"=FALSE, "Italic"=FALSE, "Underline"=FALSE, "Strikeout"=FALSE}, "Type"={"Type&direction"=enum."Select", "Embedded"=FALSE, "Encoding"=""}}}, "Link"={"Hyperlink"="", "Font complete"={"Name"="", "Size"=-1.0, "Color"=255, "Style"={"Bold"=FALSE, "Italic"=TRUE, "Underline"=FALSE, "Strikeout"=FALSE}, "Type"={"Type&direction"=enum."Select", "Embedded"=FALSE, "Encoding"=""}}}, "Paragraphe"={" Aligment"=enum."Select", "Line spacing"=enum."Select"}, "Indentation"={"Left"=0.0, "Right"=0.0}}]
  in  "Texte I4":string="\n\ni) The generic name for captions\n\nYou can specify a generic name for figure captions and tables. If you write in Figure.Caption \"Figure\" and in Figure.Separator \":\" then for each picture (or pictures) that you add a caption, it will be written into the PDF document: \"Figure 1: Caption of Figure 1\", \" Figure 2: Caption of Figure 2\" and so on. The numbering is automatic.\nii) Unit (default = mm)\n\nThe basic unit used throughout the PDF report (mm or inch)\n\niii) File path or directory\n\nIf you only specify the directory, a dialog box will appear when the program runs,  asking for the file name to use.\n\niv) Default Font\n\nThis is the font (name, color, size and style) used in the document when no other font is specified. The font name is a string. The fonts available are those that appear in the directory \"C: \\ Windows \\ Fonts\". If you specify a font that is not available or misspelled, the font \"Helvetica\" will be substituted.\n\nv) The line spacing and text alignment\n \nYou have the choice of line spacing 1.0, 1.5 and 2.0. Text alignment can be: centered, justify, left or right.\n\nvi) Page Setup\n\nYou choose the page size (default or not), orientation and margins. If the chosen format is \"Custom\", then you must specify the width X (mm or inch) and height Y (mm or inch). This format will be used in the document as you will not change the page size.\n\nvii) The metadata of the PDF (PDF Details)\n\nThis is metadata that you see when you look after the properties from the PDF file that you created (File>>Properties and Description tab).\n\n"
  in  "Texte I3 [ ]":T33=[{"Text"={"Text"="a) Creating a new PDF report with \"New PDF.vi\"", "Path"=path "", "Font complete"={"Name"="", "Size"=-1.0, "Color"=0, "Style"={"Bold"=TRUE, "Italic"=FALSE, "Underline"=FALSE, "Strikeout"=FALSE}, "Type"={"Type&direction"=enum."Select", "Embedded"=FALSE, "Encoding"=""}}}, "Link"={"Hyperlink"="", "Font complete"={"Name"="", "Size"=-1.0, "Color"=255, "Style"={"Bold"=FALSE, "Italic"=TRUE, "Underline"=FALSE, "Strikeout"=FALSE}, "Type"={"Type&direction"=enum."Select", "Embedded"=FALSE, "Encoding"=""}}}, "Paragraphe"={" Aligment"=enum."Select", "Line spacing"=enum."Select"}, "Indentation"={"Left"=0.0, "Right"=0.0}}, {"Text"={"Text"="\nThe first step is to create a new PDF report. The variables in the PDF report are:\n\n          i) generic names for captions of figures and tables;\n          ii) the unit used;\n          iii) the directory or file name (full path) to use;\n          iv) the default font of the document;\n          v) the line spacing and the default alignment of the document;\n          vi) the format of the page;\n          vii) the metadata about the PDF file created;\n          viii) the file permissions;\n          ix) the opening of the PDF file generated.\n", "Path"=path "", "Font complete"={"Name"="", "Size"=-1.0, "Color"=0, "Style"={"Bold"=FALSE, "Italic"=FALSE, "Underline"=FALSE, "Strikeout"=FALSE}, "Type"={"Type&direction"=enum."Select", "Embedded"=FALSE, "Encoding"=""}}}, "Link"={"Hyperlink"="", "Font complete"={"Name"="", "Size"=-1.0, "Color"=255, "Style"={"Bold"=FALSE, "Italic"=TRUE, "Underline"=FALSE, "Strikeout"=FALSE}, "Type"={"Type&direction"=enum."Select", "Embedded"=FALSE, "Encoding"=""}}}, "Paragraphe"={" Aligment"=enum."Select", "Line spacing"=enum."Select"}, "Indentation"={"Left"=0.0, "Right"=0.0}}]
  in  "Texte I2 [ ]":T33=[{"Text"={"Text"="\nDocument palette consists of 6 VIs:\n\na)\tNew PDF.vi;\nb)\tClose PDF.vi;\nc)\tAppend New Page.vi;\nd)\tSet Page Size.vi;\ne)\tSet Default Font.vi;\nf)\tPrint PDF.vi.\n", "Path"=path "", "Font complete"={"Name"="", "Size"=-1.0, "Color"=0, "Style"={"Bold"=FALSE, "Italic"=FALSE, "Underline"=FALSE, "Strikeout"=FALSE}, "Type"={"Type&direction"=enum."Select", "Embedded"=FALSE, "Encoding"=""}}}, "Link"={"Hyperlink"="", "Font complete"={"Name"="", "Size"=-1.0, "Color"=255, "Style"={"Bold"=FALSE, "Italic"=TRUE, "Underline"=FALSE, "Strikeout"=FALSE}, "Type"={"Type&direction"=enum."Select", "Embedded"=FALSE, "Encoding"=""}}}, "Paragraphe"={" Aligment"=enum."Select", "Line spacing"=enum."Select"}, "Indentation"={"Left"=0.0, "Right"=0.0}}]
  in  "Texte I5":string="viii) The file permissions\n\nIn the following table, you have the file permissions you can set with an owner password.  The user password is for the opening of the file.\n\n"
  in  "Text I1":string="The \"Document\" palette"
  in  "Texte J2 [ ]":T33=[{"Text"={"Text"="\nThe header, footer and watermark can be added anywhere during the creation of the report because they are written at the end with \"Close PDF.vi\". For reasons of clarity, we put them immediately after the creation of new PDF report.\n\nA header or footer is a table with one row and a maximum of three columns of equal widths. The number of elements added to a header or a footer (text, image or page number) gives the number of columns for the table.\n\nThe total width of the header (or footer) is the text zone (page width minus the left margin and the right margin). The height of the header (or footer) is the margin (top or bottom) minus 10 mm (0.394\"). The header or the footer is centered vertically.\n", "Path"=path "", "Font complete"={"Name"="", "Size"=-1.0, "Color"=0, "Style"={"Bold"=FALSE, "Italic"=FALSE, "Underline"=FALSE, "Strikeout"=FALSE}, "Type"={"Type&direction"=enum."Select", "Embedded"=FALSE, "Encoding"=""}}}, "Link"={"Hyperlink"="", "Font complete"={"Name"="", "Size"=-1.0, "Color"=255, "Style"={"Bold"=FALSE, "Italic"=TRUE, "Underline"=FALSE, "Strikeout"=FALSE}, "Type"={"Type&direction"=enum."Select", "Embedded"=FALSE, "Encoding"=""}}}, "Paragraphe"={" Aligment"=enum."Select", "Line spacing"=enum."Select"}, "Indentation"={"Left"=0.0, "Right"=0.0}}]
  in  "Texte J4 [ ]":T33=[{"Text"={"Text"=" Header", "Path"=path "", "Font complete"={"Name"="", "Size"=-1.0, "Color"=0, "Style"={"Bold"=TRUE, "Italic"=FALSE, "Underline"=FALSE, "Strikeout"=FALSE}, "Type"={"Type&direction"=enum."Select", "Embedded"=FALSE, "Encoding"=""}}}, "Link"={"Hyperlink"="", "Font complete"={"Name"="", "Size"=-1.0, "Color"=255, "Style"={"Bold"=FALSE, "Italic"=TRUE, "Underline"=FALSE, "Strikeout"=FALSE}, "Type"={"Type&direction"=enum."Select", "Embedded"=FALSE, "Encoding"=""}}}, "Paragraphe"={" Aligment"=enum."Select", "Line spacing"=enum."Select"}, "Indentation"={"Left"=0.0, "Right"=0.0}}, {"Text"={"Text"="\nIn the previous figure, we see that we added one block to the header. It follows that we will have a table consisting of a single column. If we look at the controls \"Header Text\", we can see that the variables are as follows:\n    \n    - Start Page;\n    - Text (the text in question: PDF report generation toolkit for LabVIEW...);\n    - Link (hyperlink optional - http://itextpdf.com/);\n    - The vertical and horizontal alignment (\"CENTER-top\" is selected);\n    - The font (Arial, 14 points bold).\n\nMoreover, we can add a horizontal line to separate the header or the footer from the text.\n\n", "Path"=path "", "Font complete"={"Name"="", "Size"=-1.0, "Color"=0, "Style"={"Bold"=FALSE, "Italic"=FALSE, "Underline"=FALSE, "Strikeout"=FALSE}, "Type"={"Type&direction"=enum."Select", "Embedded"=FALSE, "Encoding"=""}}}, "Link"={"Hyperlink"="", "Font complete"={"Name"="", "Size"=-1.0, "Color"=255, "Style"={"Bold"=FALSE, "Italic"=TRUE, "Underline"=FALSE, "Strikeout"=FALSE}, "Type"={"Type&direction"=enum."Select", "Embedded"=FALSE, "Encoding"=""}}}, "Paragraphe"={" Aligment"=enum."Select", "Line spacing"=enum."Select"}, "Indentation"={"Left"=0.0, "Right"=0.0}}]
  in  "Texte J5 [ ]":T33=[{"Text"={"Text"=" \nFooter", "Path"=path "", "Font complete"={"Name"="", "Size"=-1.0, "Color"=0, "Style"={"Bold"=TRUE, "Italic"=FALSE, "Underline"=FALSE, "Strikeout"=FALSE}, "Type"={"Type&direction"=enum."Select", "Embedded"=FALSE, "Encoding"=""}}}, "Link"={"Hyperlink"="", "Font complete"={"Name"="", "Size"=-1.0, "Color"=255, "Style"={"Bold"=FALSE, "Italic"=TRUE, "Underline"=FALSE, "Strikeout"=FALSE}, "Type"={"Type&direction"=enum."Select", "Embedded"=FALSE, "Encoding"=""}}}, "Paragraphe"={" Aligment"=enum."Select", "Line spacing"=enum."Select"}, "Indentation"={"Left"=0.0, "Right"=0.0}}, {"Text"={"Text"="\nWe have added three blocks to the footer. It follows that we will have a table consisting of three columns. The addition of the blocks is done from left to right:\n\n    - the first block, block \"Text\" is located to the left;\n    - the second block, block \"Image\" is located in the center;\n    - the last block, the block \"Page #\" is located right.\n\t\nIn all cases, we need to specify at which page this block begins to appear (and the vertical and horizontal alignment). The hyperlink is always optional. If an image is too large to fit into the space provided, the dimensions are automatically reduced.\n\n", "Path"=path "", "Font complete"={"Name"="", "Size"=-1.0, "Color"=0, "Style"={"Bold"=FALSE, "Italic"=FALSE, "Underline"=FALSE, "Strikeout"=FALSE}, "Type"={"Type&direction"=enum."Select", "Embedded"=FALSE, "Encoding"=""}}}, "Link"={"Hyperlink"="", "Font complete"={"Name"="", "Size"=-1.0, "Color"=255, "Style"={"Bold"=FALSE, "Italic"=TRUE, "Underline"=FALSE, "Strikeout"=FALSE}, "Type"={"Type&direction"=enum."Select", "Embedded"=FALSE, "Encoding"=""}}}, "Paragraphe"={" Aligment"=enum."Select", "Line spacing"=enum."Select"}, "Indentation"={"Left"=0.0, "Right"=0.0}}]
  in  "Texte J6 [ ]":T33=[{"Text"={"Text"=" \nWatermark\n\n", "Path"=path "", "Font complete"={"Name"="", "Size"=-1.0, "Color"=0, "Style"={"Bold"=TRUE, "Italic"=FALSE, "Underline"=FALSE, "Strikeout"=FALSE}, "Type"={"Type&direction"=enum."Select", "Embedded"=FALSE, "Encoding"=""}}}, "Link"={"Hyperlink"="", "Font complete"={"Name"="", "Size"=-1.0, "Color"=255, "Style"={"Bold"=FALSE, "Italic"=TRUE, "Underline"=FALSE, "Strikeout"=FALSE}, "Type"={"Type&direction"=enum."Select", "Embedded"=FALSE, "Encoding"=""}}}, "Paragraphe"={" Aligment"=enum."Select", "Line spacing"=enum."Select"}, "Indentation"={"Left"=0.0, "Right"=0.0}}, {"Text"={"Text"="\nThe first element in the cluster watermark is the cluster name \"General\", it consists of:\n\n    - Type (Text, Text auto and Image);\n    - Opacity (%);\n    - The angle of rotation (Rotate (°))\n    - The position (Absolute, Center on page and Center on text section);\n    - Absolute position (X (mm or inch) and Y (mm or inch)).\n\n\nThe type defines the element that we add (Text, Text auto et Image). In the case of  \" Text auto \", the angle of rotation is automatically calculated so that the text is placed on the diagonal of the area (the whole page or text zone), and the font size is maximized.\n\nBecause the watermark is placed into the foreground, you must specify its opacity. When you select \"Text\" or \"Picture\", we can specify the rotation of the text box or image.\n\nPosition \"Absolute\" applies only to the type \"Text\" or \"Picture\". When this position is selected then the point (0,0) is the lower left corner of the page.\n\n\n", "Path"=path "", "Font complete"={"Name"="", "Size"=-1.0, "Color"=0, "Style"={"Bold"=FALSE, "Italic"=FALSE, "Underline"=FALSE, "Strikeout"=FALSE}, "Type"={"Type&direction"=enum."Select", "Embedded"=FALSE, "Encoding"=""}}}, "Link"={"Hyperlink"="", "Font complete"={"Name"="", "Size"=-1.0, "Color"=255, "Style"={"Bold"=FALSE, "Italic"=TRUE, "Underline"=FALSE, "Strikeout"=FALSE}, "Type"={"Type&direction"=enum."Select", "Embedded"=FALSE, "Encoding"=""}}}, "Paragraphe"={" Aligment"=enum."Select", "Line spacing"=enum."Select"}, "Indentation"={"Left"=0.0, "Right"=0.0}}]
  in  "Texte J3":string="\n\nBlocks of the header or footer are added with \"Header or Footer polymorphic.vi\" and the watermark with \"Append Watermark.vi\".\n"
  in  "TexteJ7":string="\nFor the watermark, it is impossible  to change the style of a font (bold, italic, underline and strikeout) and Watermark supports only ASCII characters.\n\n"
  in  "Text J1":string="The \"Header, Footer and Watermark\" palette"
  in  "Texte K2 [ ]":T33=[{"Text"={"Text"="\n\nYou could append a PDF file in the PDF Report with \"Append PDF files to PDF Report.vi\".  You have to take care if the Report has header or footer because it is added as an exact copy (the footer, and the header could be written over a part of the text you added).  The last page of this manual is added with this VI.  I also include a standalone VI to concatenate PDF files.\n\n", "Path"=path "", "Font complete"={"Name"="", "Size"=-1.0, "Color"=0, "Style"={"Bold"=FALSE, "Italic"=FALSE, "Underline"=FALSE, "Strikeout"=FALSE}, "Type"={"Type&direction"=enum."Select", "Embedded"=FALSE, "Encoding"=""}}}, "Link"={"Hyperlink"="", "Font complete"={"Name"="", "Size"=-1.0, "Color"=255, "Style"={"Bold"=FALSE, "Italic"=TRUE, "Underline"=FALSE, "Strikeout"=FALSE}, "Type"={"Type&direction"=enum."Select", "Embedded"=FALSE, "Encoding"=""}}}, "Paragraphe"={" Aligment"=enum."Select", "Line spacing"=enum."Select"}, "Indentation"={"Left"=0.0, "Right"=0.0}}]
  in  "Texte K3 [ ]":T33=[{"Text"={"Text"="The general syntax for the range that is used looks like this: [!][o][odd][e][even]start-end.   You can have multiple page ranges separated by commas. The ! modifier removes pages from what is already selected. The range changes are incremental—numbers are added or deleted as the range appears. The start or the end can be omitted. If you omit both, you need at least o (odd; selects all odd pages) or e (even; selects all even pages):\n\n", "Path"=path "", "Font complete"={"Name"="", "Size"=-1.0, "Color"=0, "Style"={"Bold"=FALSE, "Italic"=FALSE, "Underline"=FALSE, "Strikeout"=FALSE}, "Type"={"Type&direction"=enum."Select", "Embedded"=FALSE, "Encoding"=""}}}, "Link"={"Hyperlink"="", "Font complete"={"Name"="", "Size"=-1.0, "Color"=255, "Style"={"Bold"=FALSE, "Italic"=TRUE, "Underline"=FALSE, "Strikeout"=FALSE}, "Type"={"Type&direction"=enum."Select", "Embedded"=FALSE, "Encoding"=""}}}, "Paragraphe"={" Aligment"=enum."Select", "Line spacing"=enum."Select"}, "Indentation"={"Left"=0.0, "Right"=0.0}}, {"Text"={"Text"="\"all\" : complete PDF document\n\"o\":  selects all odd pages\n\"e\":  selects all even pages\n\"1-4, 6-8, !7\": selects pages 1, 2, 3,4, 6, and 8 (\"!\" excluded page 7)\n\n\n", "Path"=path "", "Font complete"={"Name"="", "Size"=-1.0, "Color"=0, "Style"={"Bold"=FALSE, "Italic"=FALSE, "Underline"=FALSE, "Strikeout"=FALSE}, "Type"={"Type&direction"=enum."Select", "Embedded"=FALSE, "Encoding"=""}}}, "Link"={"Hyperlink"="", "Font complete"={"Name"="", "Size"=-1.0, "Color"=255, "Style"={"Bold"=FALSE, "Italic"=TRUE, "Underline"=FALSE, "Strikeout"=FALSE}, "Type"={"Type&direction"=enum."Select", "Embedded"=FALSE, "Encoding"=""}}}, "Paragraphe"={" Aligment"=enum."Select", "Line spacing"=enum."Select"}, "Indentation"={"Left"=1.0, "Right"=0.0}}, {"Text"={"Text"="If a PDF file is not protected, then Password = empty string. If the PDF file is protected you need to provide:\n\n", "Path"=path "", "Font complete"={"Name"="", "Size"=-1.0, "Color"=0, "Style"={"Bold"=FALSE, "Italic"=FALSE, "Underline"=FALSE, "Strikeout"=FALSE}, "Type"={"Type&direction"=enum."Select", "Embedded"=FALSE, "Encoding"=""}}}, "Link"={"Hyperlink"="", "Font complete"={"Name"="", "Size"=-1.0, "Color"=255, "Style"={"Bold"=FALSE, "Italic"=TRUE, "Underline"=FALSE, "Strikeout"=FALSE}, "Type"={"Type&direction"=enum."Select", "Embedded"=FALSE, "Encoding"=""}}}, "Paragraphe"={" Aligment"=enum."Select", "Line spacing"=enum."Select"}, "Indentation"={"Left"=0.0, "Right"=0.0}}, {"Text"={"Text"="- the owner password (if protected with a user and an owner password);\n- the owner password (if protected with only an owner password);\n- the user password (if protected with only a user password).\n", "Path"=path "", "Font complete"={"Name"="", "Size"=-1.0, "Color"=0, "Style"={"Bold"=FALSE, "Italic"=FALSE, "Underline"=FALSE, "Strikeout"=FALSE}, "Type"={"Type&direction"=enum."Select", "Embedded"=FALSE, "Encoding"=""}}}, "Link"={"Hyperlink"="", "Font complete"={"Name"="", "Size"=-1.0, "Color"=255, "Style"={"Bold"=FALSE, "Italic"=TRUE, "Underline"=FALSE, "Strikeout"=FALSE}, "Type"={"Type&direction"=enum."Select", "Embedded"=FALSE, "Encoding"=""}}}, "Paragraphe"={" Aligment"=enum."Select", "Line spacing"=enum."Select"}, "Indentation"={"Left"=1.0, "Right"=0.0}}]
  in  "Text k1":string="The \"Concatenate\" palette"
  in  "Text L1":string="The \"Table of Contents\" palette"
  in  "Text L2":string="\nYou could add auto numbering bookmark (Append Chapter bookmark.vi) and you could add a Table of Contents (Append a Table of Contents.vi).\n"
  in  "Text L3":string="\nAppend Chapter bookmark.vi works with UTF-16 characters like you can see in this manual.\n"
  in  "Text L4":string="\nYou could also add a table of contents with \"Append a Table of Contents.vi\".  Bookmarks you set (with \"Append Chapter bookmark.vi\") are then used to generate the table of contents.  If you left click on the text  of the table of content you will jump to the corresponding section for ASCII text, but you will not jump for UTF-16 text.  \n"
  in  "Text M1":string="The \"Tools\" palette"
  in  "Text M2":string="All the VIs in this palette are standalone.\n\nThe first two VIs (\"Read Unicode File.vi\" and \"Get Available Font Encoding [ ].vi\") will be discussed in the next section of the document.\n\nThe third VI \"Change AcroField Value (String).vi\" allows to change the value of an AcroField (string) of a PDF form.\n\nThe fourth VI \"Read AcroFields.vi\" allows to read the list of AcroFields in a PDF form.\n\n\n"
  in  "Texte N4 [ ]":T33=[{"Text"={"Text"="\nYou have access to the characters U+0000 to U+FFFF (what is in the \"Character Map\" of Windows).  I know two methods to write Unicode text in a LabVIEW string:\n\n", "Path"=path "", "Font complete"={"Name"="", "Size"=-1.0, "Color"=0, "Style"={"Bold"=FALSE, "Italic"=FALSE, "Underline"=FALSE, "Strikeout"=FALSE}, "Type"={"Type&direction"=enum."Select", "Embedded"=FALSE, "Encoding"=""}}}, "Link"={"Hyperlink"="", "Font complete"={"Name"="", "Size"=-1.0, "Color"=255, "Style"={"Bold"=FALSE, "Italic"=TRUE, "Underline"=FALSE, "Strikeout"=FALSE}, "Type"={"Type&direction"=enum."Select", "Embedded"=FALSE, "Encoding"=""}}}, "Paragraphe"={" Aligment"=enum."Select", "Line spacing"=enum."Select"}, "Indentation"={"Left"=0.0, "Right"=0.0}}, {"Text"={"Text"="1) enable Unicode support by adding the following setting in the LabVIEW.ini \"UseUnicode=True\" (see \"<a>A List of Tips and Tools for using Unicode in LabVIEW</a>\") and write directly in the string control.\n2) read an Unicode text file and copy it in a string.", "Path"=path "", "Font complete"={"Name"="", "Size"=-1.0, "Color"=0, "Style"={"Bold"=FALSE, "Italic"=FALSE, "Underline"=FALSE, "Strikeout"=FALSE}, "Type"={"Type&direction"=enum."Select", "Embedded"=FALSE, "Encoding"=""}}}, "Link"={"Hyperlink"="https://decibel.ni.com/content/docs/DOC-10153", "Font complete"={"Name"="", "Size"=-1.0, "Color"=255, "Style"={"Bold"=FALSE, "Italic"=TRUE, "Underline"=FALSE, "Strikeout"=FALSE}, "Type"={"Type&direction"=enum."Select", "Embedded"=FALSE, "Encoding"=""}}}, "Paragraphe"={" Aligment"=enum."Select", "Line spacing"=enum."Select"}, "Indentation"={"Left"=0.75, "Right"=0.0}}, {"Text"={"Text"="\nI stopped to use the first method because I often had unexpected LabVIEW crash or strange things have happened (like what JackDunaway has reported in <a>post 657</a>).  If I want to use Unicode I write the text in Notepad and I save with the encoding Unicode.\n\n", "Path"=path "", "Font complete"={"Name"="", "Size"=-1.0, "Color"=0, "Style"={"Bold"=FALSE, "Italic"=FALSE, "Underline"=FALSE, "Strikeout"=FALSE}, "Type"={"Type&direction"=enum."Select", "Embedded"=FALSE, "Encoding"=""}}}, "Link"={"Hyperlink"="http://forums.ni.com/t5/BreakPoint/Rube-Goldberg-Code/m-p/1106596#M11877", "Font complete"={"Name"="", "Size"=-1.0, "Color"=255, "Style"={"Bold"=FALSE, "Italic"=TRUE, "Underline"=FALSE, "Strikeout"=FALSE}, "Type"={"Type&direction"=enum."Select", "Embedded"=FALSE, "Encoding"=""}}}, "Paragraphe"={" Aligment"=enum."Select", "Line spacing"=enum."Select"}, "Indentation"={"Left"=0.0, "Right"=0.0}}]
  in  "Text N1":string="U\u0000n\u0000i\u0000c\u0000o\u0000d\u0000e\u0000 \u0000U\u0000T\u0000F\u0000-\u00001\u00006\u0000 \u0000(\u0000B\u0000a\u0000s\u0000i\u0000c\u0000 \u0000M\u0000u\u0000l\u0000t\u0000i\u0000l\u0000i\u0000n\u0000g\u0000u\u0000a\u0000l\u0000 \u0000P\u0000l\u0000a\u0000n\u0000e\u0000)\u0000 \u0000i\u0000n\u0000 \u0000P\u0000D\u0000F\u0000 \u0000R\u0000e\u0000p\u0000o\u0000r\u0000t\u0000 \u0000(\u0000.\u0004=\u00048\u0004:\u0004>\u00044\u0004)\u0000"
  in  "Font N1":T11={"Name"="Arial Unicode MS", "Size"=-1.0, "Color"=0, "Style"={"Bold"=TRUE, "Italic"=FALSE, "Underline"=FALSE, "Strikeout"=FALSE}, "Type"={"Type&direction"=enum."UTF-16", "Embedded"=FALSE, "Encoding"="CP1251"}}
  in  "Text N10":string="\nIf you want to know the different encoding supported by a font you can use \"Get Available Font Encoding [ ].vi\" from the tools' palette (you need at least to know one supported encoding).\n\n"
  in  "Text N8":string="\nHere is the string in the PDF Report with font = \"Arial Unicode MS\", Bold = True, Encoding = CP1251 (cyrillic) and type = unicode:\n\n"
  in  "Text N6":string="Here is the original text saved in Notepad (as Unicode).\n"
  in  "Text N5":string="Then I read the file with \"Read Unicode File.vi\" (in the tools palette) and I copy the text from \"Copy from this string\" in the string of the PDF Report.  \n\nBecause we have not enabled Unicode support, and we don't want to activate that support, then what you see in the normal display is not shown correctly, but the hexagonal values from the string are correct."
  in  "Text N9":string
  in  "Text N7":string="\nHere is the text copied in the string of the PDF Report. \n"
  in  "Text N3":string="How to write Unicode text in a string"
  in  "Text N11":string="Which VIs support Unicode"
  in  "Text N2":string="\nWarning:  Unicode is not officially supported by LabVIEW.\n\n"
  in  "Text O2 [ ]":T33=[{"Text"={"Text"="\n\n\nError 1172\n\n", "Path"=path "", "Font complete"={"Name"="", "Size"=-1.0, "Color"=0, "Style"={"Bold"=TRUE, "Italic"=FALSE, "Underline"=FALSE, "Strikeout"=FALSE}, "Type"={"Type&direction"=enum."Select", "Embedded"=FALSE, "Encoding"=""}}}, "Link"={"Hyperlink"="", "Font complete"={"Name"="", "Size"=-1.0, "Color"=255, "Style"={"Bold"=FALSE, "Italic"=TRUE, "Underline"=FALSE, "Strikeout"=FALSE}, "Type"={"Type&direction"=enum."Select", "Embedded"=FALSE, "Encoding"=""}}}, "Paragraphe"={" Aligment"=enum."Select", "Line spacing"=enum."Select"}, "Indentation"={"Left"=0.0, "Right"=0.0}}, {"Text"={"Text"="If the built application is running from a Network Drive take a look at:   <a>Running LabVIEW VIs or Executables That Use .NET Assemblies From a Network Drive</a>.  This text is at the next page of the manual.", "Path"=path "", "Font complete"={"Name"="", "Size"=-1.0, "Color"=0, "Style"={"Bold"=FALSE, "Italic"=FALSE, "Underline"=FALSE, "Strikeout"=FALSE}, "Type"={"Type&direction"=enum."Select", "Embedded"=FALSE, "Encoding"=""}}}, "Link"={"Hyperlink"="http://digital.ni.com/public.nsf/allkb/F326A891E72073B486256EEC0006E019", "Font complete"={"Name"="", "Size"=-1.0, "Color"=255, "Style"={"Bold"=FALSE, "Italic"=TRUE, "Underline"=FALSE, "Strikeout"=FALSE}, "Type"={"Type&direction"=enum."Select", "Embedded"=FALSE, "Encoding"=""}}}, "Paragraphe"={" Aligment"=enum."Select", "Line spacing"=enum."Select"}, "Indentation"={"Left"=0.0, "Right"=0.0}}, {"Text"={"Text"="\n\n\nFor the built application:\n\n", "Path"=path "", "Font complete"={"Name"="", "Size"=-1.0, "Color"=0, "Style"={"Bold"=TRUE, "Italic"=FALSE, "Underline"=FALSE, "Strikeout"=FALSE}, "Type"={"Type&direction"=enum."Select", "Embedded"=FALSE, "Encoding"=""}}}, "Link"={"Hyperlink"="", "Font complete"={"Name"="", "Size"=-1.0, "Color"=255, "Style"={"Bold"=FALSE, "Italic"=TRUE, "Underline"=FALSE, "Strikeout"=FALSE}, "Type"={"Type&direction"=enum."Select", "Embedded"=FALSE, "Encoding"=""}}}, "Paragraphe"={" Aligment"=enum."Select", "Line spacing"=enum."Select"}, "Indentation"={"Left"=0.0, "Right"=0.0}}, {"Text"={"Text"="“Properties>>Source Files>>Always included” add “itextsharp.dll”\n\niTextSharp.dll is located at:\n\nC:\\Program Files\\National Instruments\\LabVIEW XXXX\\vi.lib\\Exaprom PDF\\\n                                                                                                   DLL\\itextsharp.dll", "Path"=path "", "Font complete"={"Name"="", "Size"=-1.0, "Color"=0, "Style"={"Bold"=FALSE, "Italic"=FALSE, "Underline"=FALSE, "Strikeout"=FALSE}, "Type"={"Type&direction"=enum."Select", "Embedded"=FALSE, "Encoding"=""}}}, "Link"={"Hyperlink"="", "Font complete"={"Name"="", "Size"=-1.0, "Color"=255, "Style"={"Bold"=FALSE, "Italic"=TRUE, "Underline"=FALSE, "Strikeout"=FALSE}, "Type"={"Type&direction"=enum."Select", "Embedded"=FALSE, "Encoding"=""}}}, "Paragraphe"={" Aligment"=enum."LEFT", "Line spacing"=enum."Select"}, "Indentation"={"Left"=0.0, "Right"=0.0}}]
  in  "PDF Files  to concatenate and pages":T36={"Path"=path "C:/Program Files (x86)/National Instruments/LabVIEW 2013/vi.lib/Exaprom PDF/Examples/Images/Running LabVIEW VIs or Executables That Use .NET Assemblies From a Network Drive.pdf", "Pages"="all", "Password"=""}
  in  "Text O1":string="Build application with error 1172"
  in  "Image F4":cluster{"Nom":path, "Légende":string}={"Nom"=path "C:/Program Files/National Instruments/LabVIEW 2009/vi.lib/Exaprom PDF/Examples/Images/Palette Text/Palette Text.jpg", "Légende"="Text palette and the VI \"Append Text polymorphic.vi\""}
  in  "Image H8":cluster{"Nom":path, "Légende":string}={"Nom"=path "C:/Program Files/National Instruments/LabVIEW 2009/vi.lib/Exaprom PDF/Examples/Images/Palette Table/Custom Borders.jpg", "Légende"="Custom borders"}
  in  "Image C2":cluster{"Nom":path, "Légende":string}={"Nom"=path "C:/Program Files/National Instruments/LabVIEW 2009/vi.lib/Exaprom PDF/Examples/Images/Installation/Folder programming.jpg", "Légende"="Folder \"Exaprom PDF\""}
  in  "Image F5":cluster{"Nom":path, "Légende":string}={"Nom"=path "C:/Program Files/National Instruments/LabVIEW 2009/vi.lib/Exaprom PDF/Examples/Images/Palette Text/Controls Text poly.jpg", "Légende"="The main variables for the different VIs of \"Append Text polymorphic.vi\""}
  in  "Image G1":cluster{"Nom":path, "Légende":string}={"Nom"=path "C:/Program Files/National Instruments/LabVIEW 2009/vi.lib/Exaprom PDF/Examples/Images/Palette Images/Palette Image.jpg", "Légende"="The VIs to insert images in PDF documents (this image was\nadded with \"Append Image.vi\")"}
  in  "Image H1":cluster{"Nom":path, "Légende":string}={"Nom"=path "C:/Program Files/National Instruments/LabVIEW 2009/vi.lib/Exaprom PDF/Examples/Images/Palette Table/Palette Table.jpg", "Légende"="The three VIs to create a table"}
  in  "Image H2":cluster{"Nom":path, "Légende":string}={"Nom"=path "C:/Program Files/National Instruments/LabVIEW 2009/vi.lib/Exaprom PDF/Examples/Images/Palette Table/Create table B.jpg", "Légende"="Table creation"}
  in  "Image H3":cluster{"Nom":path, "Légende":string}={"Nom"=path "C:/Program Files/National Instruments/LabVIEW 2009/vi.lib/Exaprom PDF/Examples/Images/Palette Table/Create Table VI.jpg", "Légende"="Create Table.vi and default values"}
  in  "Image D1":cluster{"Nom":path, "Légende":string}={"Nom"=path "C:/Program Files/National Instruments/LabVIEW 2009/vi.lib/Exaprom PDF/Examples/Images/Simplified Report block diagram V2.jpg", "Légende"="\"Bloc Diagram\" of a simplified PDF Report"}
  in  "Image E1":cluster{"Nom":path, "Légende":string}={"Nom"=path "C:/Program Files/National Instruments/LabVIEW 2009/vi.lib/Exaprom PDF/Examples/Images/Page Layout V2.jpg", "Légende"="Text zone and origin"}
  in  "Image G2":string="Font Panel Image (this image was added with  \"Append Front Panel Image.vi\")"
  in  "Image H6":cluster{"Nom":path, "Légende":string}={"Nom"=path "C:/Program Files/National Instruments/LabVIEW 2009/vi.lib/Exaprom PDF/Examples/Images/Palette Table/Predefined borders.jpg", "Légende"="Choice of table borders (the default is framed)."}
  in  "Image H5":cluster{"Nom":path, "Légende":string}={"Nom"=path "C:/Program Files/National Instruments/LabVIEW 2009/vi.lib/Exaprom PDF/Examples/Images/Palette Table/Append Table VI.jpg", "Légende"="Append Table.vi and default values"}
  in  "Image G3":string="Block Diagram Image (this image was added with \"Append Block Diagram Image.vi\")"
  in  "Add block diagram":bool=TRUE caption="Add block \ndiagram image"
  in  "Image C3":cluster{"Nom":path, "Légende":string}={"Nom"=path "C:/Program Files/National Instruments/LabVIEW 2009/vi.lib/Exaprom PDF/Examples/Images/Installation/Folder menu.jpg", "Légende"="File \"exaprompdf.mnu\""}
  in  "Image C4":cluster{"Nom":path, "Légende":string}={"Nom"=path "C:/Program Files/National Instruments/LabVIEW 2009/vi.lib/Exaprom PDF/Examples/Images/Installation/Palette Exaprom.jpg", "Légende"="Palette \"PDF Exaprom\""}
  in  "Image F2":cluster{"Nom":path, "Légende":string}={"Nom"=path "C:/Program Files/National Instruments/LabVIEW 2009/vi.lib/Exaprom PDF/Examples/Images/Palette Text/Controls Text Types.jpg", "Légende"="Text Types (ASCII or Unicode) and writing directions"}
  in  "Image H7":cluster{"Nom":path, "Légende":string}={"Nom"=path "C:/Program Files/National Instruments/LabVIEW 2009/vi.lib/Exaprom PDF/Examples/Images/Palette Table/Table Standard Format.jpg", "Légende"="Cell format for the column headers, the row headers and the data "}
  in  "Image H9":cluster{"Nom":path, "Légende":string}={"Nom"=path "C:/Program Files/National Instruments/LabVIEW 2009/vi.lib/Exaprom PDF/Examples/Images/Palette Table/Append Customized VI.jpg", "Légende"="Append Customized Table.vi and default values"}
  in  "Image H10":cluster{"Nom":path, "Légende":string}={"Nom"=path "C:/Program Files/National Instruments/LabVIEW 2009/vi.lib/Exaprom PDF/Examples/Images/Palette Table/Control for Append Customized Table VI.jpg", "Légende"="Specific control for \"Append Customized Table.vi\" at the right bottom"}
  in  "Cluster of images controls":T40={"Scale (%)"=55.0, "Position"={"Alignment"=enum."Left (textwrap)", "X "=0.0, "Y"=0.0, "Indentation"=0.1}, "Border"={"Show?"=TRUE, "Thickness (point)"=5.0, "Color"=3418879}}
  in  "Image H11":cluster{"Nom":path, "Légende":string}={"Nom"=path "C:/Program Files/National Instruments/LabVIEW 2009/vi.lib/Exaprom PDF/Examples/Images/Palette Table/Block Diagram Tableaux 2 et 3.jpg", "Légende"="Block diagram for table 2 and 3"}
  in  "Image H12":cluster{"Nom":path, "Légende":string}={"Nom"=path "C:/Program Files/National Instruments/LabVIEW 2009/vi.lib/Exaprom PDF/Examples/Images/Palette Table/Block Diagram Tableau 4.jpg", "Légende"="Block diagram for table 4"}
  in  "Image H13":cluster{"Nom":path, "Légende":string}={"Nom"=path "C:/Program Files/National Instruments/LabVIEW 2009/vi.lib/Exaprom PDF/Examples/Images/Palette Table/Block Diagram Tableau 5.jpg", "Légende"="Block diagram for table 5"}
  in  "Image C1":cluster{"Nom":path, "Légende":string}={"Nom"=path "C:/Program Files/National Instruments/LabVIEW 2009/vi.lib/Exaprom PDF/Examples/Images/Installation/Unzip ExapromPDF 2.jpg", "Légende"="Folder \"Exaprom PD2.0\" unzipped"}
  in  "Image F3":cluster{"Nom":path, "Légende":string}={"Nom"=path "C:/Program Files/National Instruments/LabVIEW 2009/vi.lib/Exaprom PDF/Examples/Images/Palette Text/Default Paragraph.jpg", "Légende"="Alignment and line spacing"}
  in  "Image F1":cluster{"Nom":path, "Légende":string}={"Nom"=path "C:/Program Files/National Instruments/LabVIEW 2009/vi.lib/Exaprom PDF/Examples/Images/Palette Text/Font V and H clusters.jpg", "Légende"="Vertical and horizontal cluster font"}
  in  "Image H4":cluster{"Nom":path, "Légende":string}={"Nom"=path "C:/Program Files/National Instruments/LabVIEW 2009/vi.lib/Exaprom PDF/Examples/Images/Palette Table/Final table.jpg", "Légende"="Final table generated"}
  in  "Image L1":cluster{"Nom":path, "Légende":string}={"Nom"=path "C:/Program Files/National Instruments/LabVIEW 2009/vi.lib/Exaprom PDF/Examples/Images/TOC Palette/TOC palette.jpg", "Légende"="VIs of \"Table of Contents\" palette"}
  in  "Image J10":string="Text Watermark control"
  in  "Image J9":string="Image Watermark control"
  in  "Image J4":cluster{"Nom":path, "Légende":string}={"Nom"=path "C:/Program Files/National Instruments/LabVIEW 2009/vi.lib/Exaprom PDF/Examples/Images/Palette Header Footer Watermark/Header2.jpg", "Légende"="Horizontal line and block Text of the Header"}
  in  "Image J3":cluster{"Nom":path, "Légende":string}={"Nom"=path "C:/Program Files/National Instruments/LabVIEW 2009/vi.lib/Exaprom PDF/Examples/Images/Palette Header Footer Watermark/Block Diagram H F and W.jpg", "Légende"="Block Diagram for Header, Footer and Watermark"}
  in  "Image J2":cluster{"Nom":path, "Légende":string}={"Nom"=path "C:/Program Files/National Instruments/LabVIEW 2009/vi.lib/Exaprom PDF/Examples/Images/Palette Header Footer Watermark/Palette Header, Footer et Watermark.jpg", "Légende"="Header, Footer and Watermark palette"}
  in  "Image J1":cluster{"Nom":path, "Légende":string}={"Nom"=path "C:/Program Files/National Instruments/LabVIEW 2009/vi.lib/Exaprom PDF/Examples/Images/Palette Header Footer Watermark/Header footer V2.jpg", "Légende"="Header and footer"}
  in  "Image I2":cluster{"Nom":path, "Légende":string}={"Nom"=path "C:/Program Files/National Instruments/LabVIEW 2009/vi.lib/Exaprom PDF/Examples/Images/Palette Document/New PDF VI variables.jpg", "Légende"="Variables for a new PDF report"}
  in  "Image I3":cluster{"Nom":path, "Légende":string}={"Nom"=path "C:/Program Files/National Instruments/LabVIEW 2009/vi.lib/Exaprom PDF/Examples/Images/Palette Document/New PDF VI.jpg", "Légende"="New PDF.vi and his default values"}
  in  "Image I4":cluster{"Nom":path, "Légende":string}={"Nom"=path "C:/Program Files/National Instruments/LabVIEW 2009/vi.lib/Exaprom PDF/Examples/Images/Palette Document/Metadatas.jpg", "Légende"="Metada (PDF Details)"}
  in  "Image I1":cluster{"Nom":path, "Légende":string}={"Nom"=path "C:/Program Files/National Instruments/LabVIEW 2009/vi.lib/Exaprom PDF/Examples/Images/Palette Document/Palette Document.jpg", "Légende"="VIs of \"Document\" palette"}
  in  "Image J5":cluster{"Nom":path, "Légende":string}={"Nom"=path "C:/Program Files/National Instruments/LabVIEW 2009/vi.lib/Exaprom PDF/Examples/Images/Palette Header Footer Watermark/Footer Text.jpg", "Légende"="Footer Text block"}
  in  "Image J6":cluster{"Nom":path, "Légende":string}={"Nom"=path "C:/Program Files/National Instruments/LabVIEW 2009/vi.lib/Exaprom PDF/Examples/Images/Palette Header Footer Watermark/Footer Image.jpg", "Légende"="Footer Image block"}
  in  "Image J7":cluster{"Nom":path, "Légende":string}={"Nom"=path "C:/Program Files/National Instruments/LabVIEW 2009/vi.lib/Exaprom PDF/Examples/Images/Palette Header Footer Watermark/Footer Page#.jpg", "Légende"="Footer Page number block"}
  in  "Image J8":cluster{"Nom":path, "Légende":string}={"Nom"=path "C:/Program Files/National Instruments/LabVIEW 2009/vi.lib/Exaprom PDF/Examples/Images/Palette Header Footer Watermark/Two footers.jpg", "Légende"="Change the order of VIs"}
  in  "Image K1":cluster{"Nom":path, "Légende":string}={"Nom"=path "C:/Program Files/National Instruments/LabVIEW 2009/vi.lib/Exaprom PDF/Examples/Images/Palette Concatenate/Palette Concatenate.jpg", "Légende"="VIs of \"Concatenate\" palette"}
  in  "Image N1":cluster{"Nom":path, "Légende":string}={"Nom"=path "C:/Program Files/National Instruments/LabVIEW 2009/vi.lib/Exaprom PDF/Examples/Images/Unicode/Cyrillic 0410 to 042F.jpg", "Légende"="Notepad and Unicode"}
  in  "Image N2":cluster{"Nom":path, "Légende":string}={"Nom"=path "C:/Program Files/National Instruments/LabVIEW 2009/vi.lib/Exaprom PDF/Examples/Images/Unicode/Read Unicode File VI.jpg", "Légende"="Copy the text from \"Read Unicode File.vi\" and paste in  the string of the PDF Report"}
  in  "Image N3":cluster{"Nom":path, "Légende":string}={"Nom"=path "C:/Program Files/National Instruments/LabVIEW 2009/vi.lib/Exaprom PDF/Examples/Images/Unicode/Unicode string in Notepad.jpg", "Légende"="Original text in Notepad"}
  in  "Image N4":string="String in the PDF Report (not shown correctly, but the hexagonal values from the string are correct)"
  in  "Image N5":cluster{"Nom":path, "Légende":string}={"Nom"=path "C:/Program Files/National Instruments/LabVIEW 2009/vi.lib/Exaprom PDF/Examples/Images/Unicode/Get Available Font Encoding VI.jpg", "Légende"="Get Availaible Font Encoding [ ].vi for \"Arial Unicode MS\" (ARIALUNI.TTF)"}
  in  "Image K2":string="Variable of \"Append PDF file to PDF Report .vi\""
  in  "Image M1":cluster{"Nom":path, "Légende":string}={"Nom"=path "C:/Program Files/National Instruments/LabVIEW 2009/vi.lib/Exaprom PDF/Examples/Images/Tools palette/Tools palette.jpg", "Légende"="VIs of \"Tools\" palette"}
  in  "Image L2":cluster{"Nom":path, "Légende":string}={"Nom"=path "C:/Program Files/National Instruments/LabVIEW 2009/vi.lib/Exaprom PDF/Examples/Images/TOC Palette/Append Bookmark VI.jpg", "Légende"="Append Chapter bookmark.vi"}
  in  "Image L3":cluster{"Nom":path, "Légende":string}={"Nom"=path "C:/Program Files/National Instruments/LabVIEW 2009/vi.lib/Exaprom PDF/Examples/Images/TOC Palette/User Manual Bookmark.jpg", "Légende"="Bookmarks ot this User Manual"}
  in  "Image L4":cluster{"Nom":path, "Légende":string}={"Nom"=path "C:/Program Files/National Instruments/LabVIEW 2009/vi.lib/Exaprom PDF/Examples/Images/TOC Palette/Append TOC VI.jpg", "Légende"="Append a Table of Contents.vi"}
  in  "Predefined Borders Table 1":T41={"Borders"=4, "Header"={"Thickness"=1.0, "Line"=0, "Background "=16777215}, "Data"={"Thickness"=0.5, "Line"=0, "Background "=16777215}}
  in  "Image to Add [ ]":T44(array[cluster])=[{"Image name"="Arrow", "Path"=path "C:/Program Files/National Instruments/LabVIEW 2009/vi.lib/Exaprom PDF/Examples/Images/Arrow.jpg", "Scale"=7.0}, {"Image name"="Default", "Path"=path "C:/Program Files/National Instruments/LabVIEW 2009/vi.lib/Exaprom PDF/Examples/Images/Palette Text/Default font.jpg", "Scale"=100.0}, {"Image name"="A", "Path"=path "C:/Program Files/National Instruments/LabVIEW 2009/vi.lib/Exaprom PDF/Examples/Images/Palette Text/Font A.jpg", "Scale"=100.0}, {"Image name"="B", "Path"=path "C:/Program Files/National Instruments/LabVIEW 2009/vi.lib/Exaprom PDF/Examples/Images/Palette Text/Font B.jpg", "Scale"=100.0}, {"Image name"="B1", "Path"=path "C:/Program Files/National Instruments/LabVIEW 2009/vi.lib/Exaprom PDF/Examples/Images/Palette Text/Font B1.jpg", "Scale"=100.0}, {"Image name"="C", "Path"=path "C:/Program Files/National Instruments/LabVIEW 2009/vi.lib/Exaprom PDF/Examples/Images/Palette Text/Font C.jpg", "Scale"=100.0}, {"Image name"="C1", "Path"=path "C:/Program Files/National Instruments/LabVIEW 2009/vi.lib/Exaprom PDF/Examples/Images/Palette Text/Font C1.jpg", "Scale"=100.0}, {"Image name"="D", "Path"=path "C:/Program Files/National Instruments/LabVIEW 2009/vi.lib/Exaprom PDF/Examples/Images/Palette Text/Font D.jpg", "Scale"=100.0}, {"Image name"="D1", "Path"=path "C:/Program Files/National Instruments/LabVIEW 2009/vi.lib/Exaprom PDF/Examples/Images/Palette Text/Font D1.jpg", "Scale"=100.0}, {"Image name"="E", "Path"=path "C:/Program Files/National Instruments/LabVIEW 2009/vi.lib/Exaprom PDF/Examples/Images/Palette Text/Font E.jpg", "Scale"=100.0}, {"Image name"="E1", "Path"=path "C:/Program Files/National Instruments/LabVIEW 2009/vi.lib/Exaprom PDF/Examples/Images/Palette Text/Font E1.jpg", "Scale"=100.0}, {"Image name"="Logo", "Path"=path "C:/Program Files/National Instruments/LabVIEW 2009/vi.lib/Exaprom PDF/Examples/Images/Logo Exaprom.jpg", "Scale"=15.0}, {"Image name"="Row1", "Path"=path "C:/Program Files/National Instruments/LabVIEW 2009/vi.lib/Exaprom PDF/Examples/Images/Palette Table/Row1.jpg", "Scale"=37.0}, {"Image name"="Row2", "Path"=path "C:/Program Files/National Instruments/LabVIEW 2009/vi.lib/Exaprom PDF/Examples/Images/Palette Table/Row2.jpg", "Scale"=37.0}, {"Image name"="Row3", "Path"=path "C:/Program Files/National Instruments/LabVIEW 2009/vi.lib/Exaprom PDF/Examples/Images/Palette Table/Row3.jpg", "Scale"=37.0}] {"Scale" format="%#_g %"}
  in  "Caption 1":string="Resulting font if  \"Default font\" is Arial 12 points (bold, underline, Italic and strikeout = false), Type&direction = ASCII with Embedded = F and Encoding = CP1252."
  in  "Datas properties 1":T45={"Cell Type, Alignment and LS"={"Cell Alignment"=5, "Text rotation"=enum."None", "Line spacing"=enum."Select"}, "Font"={"Name"="", "Size"=0.0, "Color"=0, "Style"={"Bold"=FALSE, "Italic"=FALSE, "Underline"=FALSE, "Strikeout"=FALSE}, "Type"={"Type&direction"=enum."Select", "Embedded"=FALSE, "Encoding"=""}}}
  in  "Column Headers 2D [ ] - Table 1":string[][](array[string])=[["Wired to terminal", "", "In the\nPDF Report", " ", "Wired to terminal", " ", "In the\nPDF Report"]]
  in  "Table columnWidth [ ] - Table 1":sgl[](array[numeric])=[1.0, 0.6, 1.0, 0.4, 1.0, 0.6, 1.0]
  in  "Table properties 1)":T48={"Table position"=1, "SpacingBefore (points)"=12.0, "SpacingAfter (points)"=12.0} {"Table position" items=["LEFT", "CENTER", "RIGHT"]}
  in  "Text Data 2D [ ] - Table 1":string[][](array[string])=[["nothing", "Arrow", "Default", "", "C", "Arrow", "C1"], ["A", "Arrow", "Default", "", "D", "Arrow", "D1"], ["B", "Arrow", "B1", "", "E", "Arrow", "E1"]]
  in  "Custom Table Borders 1":T50=[{"Row"={"#"=0, "to #"=0}, "Line"={"Thickness"=1.5, "Color"=0}, "Column Borders [ ]"=[{"Cell Border"=8, "BG"=16776704}, {"Cell Border"=4, "BG"=16776704}, {"Cell Border"=18, "BG"=16776704}, {"Cell Border"=0, "BG"=16777225}, {"Cell Border"=8, "BG"=16776704}, {"Cell Border"=4, "BG"=16776704}, {"Cell Border"=18, "BG"=16776704}]}, {"Row"={"#"=1, "to #"=-1}, "Line"={"Thickness"=0.75, "Color"=0}, "Column Borders [ ]"=[{"Cell Border"=2, "BG"=16777225}, {"Cell Border"=1, "BG"=16777225}, {"Cell Border"=17, "BG"=16777225}, {"Cell Border"=0, "BG"=16777225}, {"Cell Border"=2, "BG"=16777225}, {"Cell Border"=1, "BG"=16777225}, {"Cell Border"=17, "BG"=16777225}]}]
  in  "Table columnWidth [ ]  - Tables 3 and 4":sgl[](array[numeric])=[1.0, 1.4, 1.4, 1.4]
  in  "Column Headers 2D [ ] - Tables 2 to 4":string[][](array[string])=[["Time", "Thermocouple 1\n(°C)", "Thermocouple 2\n(°C)", "Thermocouple 3\n(°C)"]]
  in  "Text Data 2D [ ]  - Tables 2 to 4":string[][](array[string])=[["09:59:42", "214.8", "212.3", "216.1"], ["09:59:52", "215.0", "212.4", "217.8"], ["10:00:02", "215.0", "212.0", "217.7"], ["10:00:12", "214.1", "211.6", "217.2"], ["10:00:22", "214.2", "212.6", "217.3"], ["10:00:32", "214.6", "212.5", "217.8"], ["10:00:42", "214.6", "212.5", "217.8"], ["10:00:52", "214.8", "212.5", "216.3"], ["10:01:02", "215.6", "211.7", "216.7"], ["10:01:12", "214.6", "211.1", "218.0"]]
  in  "Table properties  - Tables 2 to 4":T48={"Table position"=1, "SpacingBefore (points)"=12.0, "SpacingAfter (points)"=12.0} {"Table position" items=["LEFT", "CENTER", "RIGHT"]}
  in  "Caption - Table 2":string="Example of a table with the variable columnWidth [ ] \"not wired"
  in  "Caption - Table 3":string="Example of a table with the variable columnWidth [ ] \"wired"
  in  "Caption - Table 4":string="Example with Row Background color"
  in  "Row background color - Table 4":T55={"color"=14606046, "at each"=3}
  in  "Predefined Borders - Table 4":T41={"Borders"=2, "Header"={"Thickness"=1.0, "Line"=0, "Background "=15990711}, "Data"={"Thickness"=0.5, "Line"=0, "Background "=16777215}}
  in  "Datas format - Table 4":T45={"Cell Type, Alignment and LS"={"Cell Alignment"=5, "Text rotation"=enum."None", "Line spacing"=enum."Select"}, "Font"={"Name"="", "Size"=0.0, "Color"=0, "Style"={"Bold"=FALSE, "Italic"=FALSE, "Underline"=FALSE, "Strikeout"=FALSE}, "Type"={"Type&direction"=enum."Select", "Embedded"=FALSE, "Encoding"=""}}}
  in  "Column Header format - Table 4":T45={"Cell Type, Alignment and LS"={"Cell Alignment"=5, "Text rotation"=enum."None", "Line spacing"=enum."Select"}, "Font"={"Name"="", "Size"=0.0, "Color"=0, "Style"={"Bold"=FALSE, "Italic"=FALSE, "Underline"=FALSE, "Strikeout"=FALSE}, "Type"={"Type&direction"=enum."Select", "Embedded"=FALSE, "Encoding"=""}}}
  in  "Table columnWidth [ ] - Table 5":sgl[](array[numeric])=[0.75, 0.6, 0.6, 0.6, 0.6, 0.6, 0.6]
  in  "Column Headers 2D [ ] - Table 5":string[][](array[string])=[["", "Furnace (°C)", "", "", "Crucible (°C)", "", ""], ["", "Thermocouple 1", "Thermocouple 2", "Thermocouple 3", "Thermocouple 4", "Thermocouple 5", "Thermocouple 6"]]
  in  "Text Data 2D [ ] - Table 5":string[][](array[string])=[["722.2", "753.0", "714.6", "647.7", "649.3", "644.9"], ["722.9", "751.2", "711.4", "646.4", "652.7", "646.9"], ["721.8", "753.0", "713.0", "645.3", "652.5", "645.4"], ["724.2", "750.9", "711.6", "648.9", "651.1", "644.0"], ["723.7", "752.4", "710.7", "648.4", "650.6", "645.3"], ["723.9", "753.8", "712.2", "645.3", "648.9", "646.8"], ["722.6", "754.1", "710.5", "645.7", "651.0", "645.8"], ["724.6", "751.2", "713.8", "648.8", "648.6", "644.4"], ["722.9", "750.7", "710.8", "645.7", "649.7", "647.2"], ["721.8", "755.0", "713.7", "646.8", "652.2", "644.5"], ["723.1", "752.5", "712.2", "646.9", "650.7", "645.5"]]
  in  "Table properties - Table 5":T48={"Table position"=1, "SpacingBefore (points)"=12.0, "SpacingAfter (points)"=12.0} {"Table position" items=["LEFT", "CENTER", "RIGHT"]}
  in  "Caption - Table 5":string="Example with merge cell"
  in  "Row Headers 1D [ ] - Table 5":string[](array[string])=["Test 1", "Test 2", "Test 3", "Test 4", "Test 5", "Test 6", "Test 7", "Test 8", "Test 9", "\nTest 10\n ", "Mean"]
  in  "Row  [ ] - Table 5":T56=[{"Row"={"From #"=0, "to #"=0}, "Cell [ ]"=[{"Text"={"Cell Alignment"=5, "Text rotation"=enum."None", "Line spacing"=enum."Select"}, "Cell Appearance"={"Border"=0, "Thickness"=0.5, "Color"=0, "BG"=16777225}, "HMerge"={"From"=-1, "to"=-1}, "VMerge"={"From"=-1, "to"=-1}, "Font"={"Name"="", "Size"=-1.0, "Color"=0, "Style"={"Bold"=FALSE, "Italic"=FALSE, "Underline"=FALSE, "Strikeout"=FALSE}, "Type"={"Type&direction"=enum."Select", "Embedded"=FALSE, "Encoding"=""}}}, {"Text"={"Cell Alignment"=5, "Text rotation"=enum."None", "Line spacing"=enum."Select"}, "Cell Appearance"={"Border"=8, "Thickness"=1.0, "Color"=0, "BG"=16777225}, "HMerge"={"From"=1, "to"=3}, "VMerge"={"From"=-1, "to"=-1}, "Font"={"Name"="", "Size"=0.0, "Color"=0, "Style"={"Bold"=TRUE, "Italic"=FALSE, "Underline"=FALSE, "Strikeout"=FALSE}, "Type"={"Type&direction"=enum."Select", "Embedded"=FALSE, "Encoding"=""}}}, {"Text"={"Cell Alignment"=5, "Text rotation"=enum."None", "Line spacing"=enum."Select"}, "Cell Appearance"={"Border"=5, "Thickness"=1.0, "Color"=0, "BG"=16777225}, "HMerge"={"From"=4, "to"=6}, "VMerge"={"From"=-1, "to"=-1}, "Font"={"Name"="", "Size"=0.0, "Color"=0, "Style"={"Bold"=TRUE, "Italic"=FALSE, "Underline"=FALSE, "Strikeout"=FALSE}, "Type"={"Type&direction"=enum."Select", "Embedded"=FALSE, "Encoding"=""}}}]}, {"Row"={"From #"=1, "to #"=1}, "Cell [ ]"=[{"Text"={"Cell Alignment"=5, "Text rotation"=enum."None", "Line spacing"=enum."Select"}, "Cell Appearance"={"Border"=0, "Thickness"=1.0, "Color"=0, "BG"=16777225}, "HMerge"={"From"=-1, "to"=-1}, "VMerge"={"From"=-1, "to"=-1}, "Font"={"Name"="", "Size"=-1.0, "Color"=0, "Style"={"Bold"=FALSE, "Italic"=FALSE, "Underline"=FALSE, "Strikeout"=FALSE}, "Type"={"Type&direction"=enum."Select", "Embedded"=FALSE, "Encoding"=""}}}, {"Text"={"Cell Alignment"=5, "Text rotation"=enum."Clockwise", "Line spacing"=enum."Select"}, "Cell Appearance"={"Border"=2, "Thickness"=1.0, "Color"=0, "BG"=16777225}, "HMerge"={"From"=-1, "to"=-1}, "VMerge"={"From"=-1, "to"=-1}, "Font"={"Name"="", "Size"=0.0, "Color"=0, "Style"={"Bold"=TRUE, "Italic"=FALSE, "Underline"=FALSE, "Strikeout"=FALSE}, "Type"={"Type&direction"=enum."Select", "Embedded"=FALSE, "Encoding"=""}}}, {"Text"={"Cell Alignment"=5, "Text rotation"=enum."Clockwise", "Line spacing"=enum."Select"}, "Cell Appearance"={"Border"=2, "Thickness"=1.0, "Color"=0, "BG"=16777225}, "HMerge"={"From"=-1, "to"=-1}, "VMerge"={"From"=-1, "to"=-1}, "Font"={"Name"="", "Size"=0.0, "Color"=0, "Style"={"Bold"=TRUE, "Italic"=FALSE, "Underline"=FALSE, "Strikeout"=FALSE}, "Type"={"Type&direction"=enum."Select", "Embedded"=FALSE, "Encoding"=""}}}, {"Text"={"Cell Alignment"=5, "Text rotation"=enum."Clockwise", "Line spacing"=enum."Select"}, "Cell Appearance"={"Border"=2, "Thickness"=1.0, "Color"=0, "BG"=16777225}, "HMerge"={"From"=-1, "to"=-1}, "VMerge"={"From"=-1, "to"=-1}, "Font"={"Name"="", "Size"=0.0, "Color"=0, "Style"={"Bold"=TRUE, "Italic"=FALSE, "Underline"=FALSE, "Strikeout"=FALSE}, "Type"={"Type&direction"=enum."Select", "Embedded"=FALSE, "Encoding"=""}}}, {"Text"={"Cell Alignment"=5, "Text rotation"=enum."Clockwise", "Line spacing"=enum."Select"}, "Cell Appearance"={"Border"=2, "Thickness"=1.0, "Color"=0, "BG"=16777225}, "HMerge"={"From"=-1, "to"=-1}, "VMerge"={"From"=-1, "to"=-1}, "Font"={"Name"="", "Size"=0.0, "Color"=0, "Style"={"Bold"=TRUE, "Italic"=FALSE, "Underline"=FALSE, "Strikeout"=FALSE}, "Type"={"Type&direction"=enum."Select", "Embedded"=FALSE, "Encoding"=""}}}, {"Text"={"Cell Alignment"=5, "Text rotation"=enum."Clockwise", "Line spacing"=enum."Select"}, "Cell Appearance"={"Border"=2, "Thickness"=1.0, "Color"=0, "BG"=16777225}, "HMerge"={"From"=-1, "to"=-1}, "VMerge"={"From"=-1, "to"=-1}, "Font"={"Name"="", "Size"=0.0, "Color"=0, "Style"={"Bold"=TRUE, "Italic"=FALSE, "Underline"=FALSE, "Strikeout"=FALSE}, "Type"={"Type&direction"=enum."Select", "Embedded"=FALSE, "Encoding"=""}}}, {"Text"={"Cell Alignment"=5, "Text rotation"=enum."Clockwise", "Line spacing"=enum."Select"}, "Cell Appearance"={"Border"=3, "Thickness"=1.0, "Color"=0, "BG"=16777225}, "HMerge"={"From"=-1, "to"=-1}, "VMerge"={"From"=-1, "to"=-1}, "Font"={"Name"="", "Size"=0.0, "Color"=0, "Style"={"Bold"=TRUE, "Italic"=FALSE, "Underline"=FALSE, "Strikeout"=FALSE}, "Type"={"Type&direction"=enum."Select", "Embedded"=FALSE, "Encoding"=""}}}]}, {"Row"={"From #"=2, "to #"=-2}, "Cell [ ]"=[{"Text"={"Cell Alignment"=4, "Text rotation"=enum."None", "Line spacing"=enum."Select"}, "Cell Appearance"={"Border"=5, "Thickness"=0.5, "Color"=0, "BG"=16777225}, "HMerge"={"From"=-1, "to"=-1}, "VMerge"={"From"=-1, "to"=-1}, "Font"={"Name"="", "Size"=-1.0, "Color"=16777222, "Style"={"Bold"=FALSE, "Italic"=FALSE, "Underline"=FALSE, "Strikeout"=FALSE}, "Type"={"Type&direction"=enum."Select", "Embedded"=FALSE, "Encoding"=""}}}, {"Text"={"Cell Alignment"=1, "Text rotation"=enum."None", "Line spacing"=enum."Select"}, "Cell Appearance"={"Border"=17, "Thickness"=0.5, "Color"=0, "BG"=16777225}, "HMerge"={"From"=-1, "to"=-1}, "VMerge"={"From"=-1, "to"=-1}, "Font"={"Name"="", "Size"=0.0, "Color"=0, "Style"={"Bold"=FALSE, "Italic"=FALSE, "Underline"=FALSE, "Strikeout"=FALSE}, "Type"={"Type&direction"=enum."Select", "Embedded"=FALSE, "Encoding"=""}}}, {"Text"={"Cell Alignment"=5, "Text rotation"=enum."None", "Line spacing"=enum."Select"}, "Cell Appearance"={"Border"=17, "Thickness"=0.5, "Color"=0, "BG"=16777225}, "HMerge"={"From"=-1, "to"=-1}, "VMerge"={"From"=-1, "to"=-1}, "Font"={"Name"="", "Size"=0.0, "Color"=0, "Style"={"Bold"=FALSE, "Italic"=FALSE, "Underline"=FALSE, "Strikeout"=FALSE}, "Type"={"Type&direction"=enum."Select", "Embedded"=FALSE, "Encoding"=""}}}, {"Text"={"Cell Alignment"=9, "Text rotation"=enum."None", "Line spacing"=enum."Select"}, "Cell Appearance"={"Border"=17, "Thickness"=0.5, "Color"=0, "BG"=16777225}, "HMerge"={"From"=-1, "to"=-1}, "VMerge"={"From"=-1, "to"=-1}, "Font"={"Name"="", "Size"=0.0, "Color"=0, "Style"={"Bold"=FALSE, "Italic"=FALSE, "Underline"=FALSE, "Strikeout"=FALSE}, "Type"={"Type&direction"=enum."Select", "Embedded"=FALSE, "Encoding"=""}}}, {"Text"={"Cell Alignment"=5, "Text rotation"=enum."None", "Line spacing"=enum."Select"}, "Cell Appearance"={"Border"=17, "Thickness"=0.5, "Color"=0, "BG"=16777225}, "HMerge"={"From"=-1, "to"=-1}, "VMerge"={"From"=-1, "to"=-1}, "Font"={"Name"="", "Size"=0.0, "Color"=0, "Style"={"Bold"=FALSE, "Italic"=FALSE, "Underline"=FALSE, "Strikeout"=FALSE}, "Type"={"Type&direction"=enum."Select", "Embedded"=FALSE, "Encoding"=""}}}, {"Text"={"Cell Alignment"=5, "Text rotation"=enum."None", "Line spacing"=enum."Select"}, "Cell Appearance"={"Border"=17, "Thickness"=0.5, "Color"=0, "BG"=16777225}, "HMerge"={"From"=-1, "to"=-1}, "VMerge"={"From"=-1, "to"=-1}, "Font"={"Name"="", "Size"=0.0, "Color"=0, "Style"={"Bold"=FALSE, "Italic"=FALSE, "Underline"=FALSE, "Strikeout"=FALSE}, "Type"={"Type&direction"=enum."Select", "Embedded"=FALSE, "Encoding"=""}}}, {"Text"={"Cell Alignment"=5, "Text rotation"=enum."None", "Line spacing"=enum."Select"}, "Cell Appearance"={"Border"=17, "Thickness"=0.5, "Color"=0, "BG"=16777225}, "HMerge"={"From"=-1, "to"=-1}, "VMerge"={"From"=-1, "to"=-1}, "Font"={"Name"="", "Size"=0.0, "Color"=0, "Style"={"Bold"=FALSE, "Italic"=FALSE, "Underline"=FALSE, "Strikeout"=FALSE}, "Type"={"Type&direction"=enum."Select", "Embedded"=FALSE, "Encoding"=""}}}]}, {"Row"={"From #"=-1, "to #"=-1}, "Cell [ ]"=[{"Text"={"Cell Alignment"=5, "Text rotation"=enum."None", "Line spacing"=enum."Select"}, "Cell Appearance"={"Border"=5, "Thickness"=1.0, "Color"=0, "BG"=15000804}, "HMerge"={"From"=-1, "to"=-1}, "VMerge"={"From"=-1, "to"=-1}, "Font"={"Name"="", "Size"=-1.0, "Color"=16777222, "Style"={"Bold"=TRUE, "Italic"=FALSE, "Underline"=FALSE, "Strikeout"=FALSE}, "Type"={"Type&direction"=enum."Select", "Embedded"=FALSE, "Encoding"=""}}}, {"Text"={"Cell Alignment"=5, "Text rotation"=enum."None", "Line spacing"=enum."Select"}, "Cell Appearance"={"Border"=18, "Thickness"=1.0, "Color"=0, "BG"=15000804}, "HMerge"={"From"=-1, "to"=-1}, "VMerge"={"From"=-1, "to"=-1}, "Font"={"Name"="", "Size"=0.0, "Color"=0, "Style"={"Bold"=TRUE, "Italic"=FALSE, "Underline"=FALSE, "Strikeout"=FALSE}, "Type"={"Type&direction"=enum."Select", "Embedded"=FALSE, "Encoding"=""}}}, {"Text"={"Cell Alignment"=5, "Text rotation"=enum."None", "Line spacing"=enum."Select"}, "Cell Appearance"={"Border"=18, "Thickness"=1.0, "Color"=0, "BG"=15000804}, "HMerge"={"From"=-1, "to"=-1}, "VMerge"={"From"=-1, "to"=-1}, "Font"={"Name"="", "Size"=0.0, "Color"=0, "Style"={"Bold"=TRUE, "Italic"=FALSE, "Underline"=FALSE, "Strikeout"=FALSE}, "Type"={"Type&direction"=enum."Select", "Embedded"=FALSE, "Encoding"=""}}}, {"Text"={"Cell Alignment"=5, "Text rotation"=enum."None", "Line spacing"=enum."Select"}, "Cell Appearance"={"Border"=18, "Thickness"=1.0, "Color"=0, "BG"=15000804}, "HMerge"={"From"=-1, "to"=-1}, "VMerge"={"From"=-1, "to"=-1}, "Font"={"Name"="", "Size"=0.0, "Color"=0, "Style"={"Bold"=TRUE, "Italic"=FALSE, "Underline"=FALSE, "Strikeout"=FALSE}, "Type"={"Type&direction"=enum."Select", "Embedded"=FALSE, "Encoding"=""}}}, {"Text"={"Cell Alignment"=5, "Text rotation"=enum."None", "Line spacing"=enum."Select"}, "Cell Appearance"={"Border"=18, "Thickness"=1.0, "Color"=0, "BG"=15000804}, "HMerge"={"From"=-1, "to"=-1}, "VMerge"={"From"=-1, "to"=-1}, "Font"={"Name"="", "Size"=0.0, "Color"=0, "Style"={"Bold"=TRUE, "Italic"=FALSE, "Underline"=FALSE, "Strikeout"=FALSE}, "Type"={"Type&direction"=enum."Select", "Embedded"=FALSE, "Encoding"=""}}}, {"Text"={"Cell Alignment"=5, "Text rotation"=enum."None", "Line spacing"=enum."Select"}, "Cell Appearance"={"Border"=18, "Thickness"=1.0, "Color"=0, "BG"=15000804}, "HMerge"={"From"=-1, "to"=-1}, "VMerge"={"From"=-1, "to"=-1}, "Font"={"Name"="", "Size"=0.0, "Color"=0, "Style"={"Bold"=TRUE, "Italic"=FALSE, "Underline"=FALSE, "Strikeout"=FALSE}, "Type"={"Type&direction"=enum."Select", "Embedded"=FALSE, "Encoding"=""}}}, {"Text"={"Cell Alignment"=5, "Text rotation"=enum."None", "Line spacing"=enum."Select"}, "Cell Appearance"={"Border"=18, "Thickness"=1.0, "Color"=0, "BG"=15000804}, "HMerge"={"From"=-1, "to"=-1}, "VMerge"={"From"=-1, "to"=-1}, "Font"={"Name"="", "Size"=0.0, "Color"=0, "Style"={"Bold"=TRUE, "Italic"=FALSE, "Underline"=FALSE, "Strikeout"=FALSE}, "Type"={"Type&direction"=enum."Select", "Embedded"=FALSE, "Encoding"=""}}}]}]
  in  "Column Headers 2D [ ] - table 6":string[][](array[string])=[["Permission", "Bit position", "Meaning"]]
  in  "Text Data 2D [ ] - table 6":string[][](array[string])=[["3", "Print the document. Print the document (possibly not at the highest quality level, depending on whether bit 12 is also set). "], ["4", "Modify the contents of the document by operations other than those controlled by bits 6, 9, and 11. "], ["5", "Copy or otherwise extract text and graphics from the document, including extracting text and graphics (in support of accessibility to users with disabilities or for other purposes). Copy or otherwise extract text and graphics from the document by operations other than that controlled by bit 10. "], ["6", "Add or modify text annotations, fill in interactive form fields, and, if bit 4 is also set, create or modify interactive form fields (including signature fields). "], ["9", "Fill in existing interactive form fields (including signature fields), even if bit 6 is clear. "], ["10", "Extract text and graphics (in support of accessibility to users with disabilities or for other purposes). "], ["11", "Assemble the document (insert, rotate, or delete pages and create bookmarks or thumbnail images), even if bit 4 is clear. "], ["12", "Print the document to a representation from which a faithful digital copy of the PDF content could be generated. When this bit is clear (and bit 3 is set), printing is limited to a low-level representation of the appearance, possibly of degraded quality. "]]
  in  "Row Headers 1D [ ] - table 6":string[](array[string])=["Allow Degradated Printing", "Allow Modify Contents", "Allow Copy", "Allow Modify Annotations", "Allow Fill In", "Allow Screen Readers", "Allow Assembly", "Allow Printing"]
  in  "Table columnWidth [ ] - table 6":sgl[](array[numeric])=[1.9, 0.7, 3.9]
  in  "Row  [ ] - table 6":T56=[{"Row"={"From #"=0, "to #"=0}, "Cell [ ]"=[{"Text"={"Cell Alignment"=5, "Text rotation"=enum."None", "Line spacing"=enum."Select"}, "Cell Appearance"={"Border"=5, "Thickness"=1.0, "Color"=0, "BG"=16777225}, "HMerge"={"From"=-1, "to"=-1}, "VMerge"={"From"=-1, "to"=-1}, "Font"={"Name"="", "Size"=0.0, "Color"=0, "Style"={"Bold"=FALSE, "Italic"=FALSE, "Underline"=FALSE, "Strikeout"=FALSE}, "Type"={"Type&direction"=enum."Select", "Embedded"=FALSE, "Encoding"=""}}}, {"Text"={"Cell Alignment"=5, "Text rotation"=enum."None", "Line spacing"=enum."Select"}, "Cell Appearance"={"Border"=18, "Thickness"=1.0, "Color"=0, "BG"=16777225}, "HMerge"={"From"=-1, "to"=-1}, "VMerge"={"From"=-1, "to"=-1}, "Font"={"Name"="", "Size"=0.0, "Color"=0, "Style"={"Bold"=FALSE, "Italic"=FALSE, "Underline"=FALSE, "Strikeout"=FALSE}, "Type"={"Type&direction"=enum."Select", "Embedded"=FALSE, "Encoding"=""}}}, {"Text"={"Cell Alignment"=5, "Text rotation"=enum."None", "Line spacing"=enum."Select"}, "Cell Appearance"={"Border"=18, "Thickness"=1.0, "Color"=0, "BG"=16777225}, "HMerge"={"From"=-1, "to"=-1}, "VMerge"={"From"=-1, "to"=-1}, "Font"={"Name"="", "Size"=0.0, "Color"=0, "Style"={"Bold"=FALSE, "Italic"=FALSE, "Underline"=FALSE, "Strikeout"=FALSE}, "Type"={"Type&direction"=enum."Select", "Embedded"=FALSE, "Encoding"=""}}}]}, {"Row"={"From #"=1, "to #"=-1}, "Cell [ ]"=[{"Text"={"Cell Alignment"=4, "Text rotation"=enum."None", "Line spacing"=enum."Select"}, "Cell Appearance"={"Border"=3, "Thickness"=0.5, "Color"=0, "BG"=16777225}, "HMerge"={"From"=-1, "to"=-1}, "VMerge"={"From"=-1, "to"=-1}, "Font"={"Name"="", "Size"=0.0, "Color"=0, "Style"={"Bold"=FALSE, "Italic"=FALSE, "Underline"=FALSE, "Strikeout"=FALSE}, "Type"={"Type&direction"=enum."Select", "Embedded"=FALSE, "Encoding"=""}}}, {"Text"={"Cell Alignment"=5, "Text rotation"=enum."None", "Line spacing"=enum."Select"}, "Cell Appearance"={"Border"=17, "Thickness"=0.5, "Color"=0, "BG"=16777225}, "HMerge"={"From"=-1, "to"=-1}, "VMerge"={"From"=-1, "to"=-1}, "Font"={"Name"="", "Size"=0.0, "Color"=0, "Style"={"Bold"=FALSE, "Italic"=FALSE, "Underline"=FALSE, "Strikeout"=FALSE}, "Type"={"Type&direction"=enum."Select", "Embedded"=FALSE, "Encoding"=""}}}, {"Text"={"Cell Alignment"=7, "Text rotation"=enum."None", "Line spacing"=enum."Select"}, "Cell Appearance"={"Border"=17, "Thickness"=0.5, "Color"=0, "BG"=16777225}, "HMerge"={"From"=-1, "to"=-1}, "VMerge"={"From"=-1, "to"=-1}, "Font"={"Name"="", "Size"=0.0, "Color"=0, "Style"={"Bold"=FALSE, "Italic"=FALSE, "Underline"=FALSE, "Strikeout"=FALSE}, "Type"={"Type&direction"=enum."Select", "Embedded"=FALSE, "Encoding"=""}}}]}]
  in  "Caption - table 6":string="Permissions from \"Document management — Portable document format — Part 1: PDF 1.7 (PDF 32000-1:2008, page 61)\""
  in  "Row  [ ] - Table 7":T56
  in  "Table properties - Table 7":T48={"Table position"=1, "SpacingBefore (points)"=12.0, "SpacingAfter (points)"=12.0} {"Table position" items=["LEFT", "CENTER", "RIGHT"]}
  in  "Text Data 2D [ ] - Table 7":string[][](array[string])
  in  "Column Headers 2D [ ] - Table 7":string[][](array[string])=[["", "ASCII", "UTF-16", "UTF-16 (deault)", "UTF-16 (LTR)", "UTF-16 (RTL)"]]
  in  "Table columnWidth [ ] - Table 7":sgl[](array[numeric])=[3.0, 0.5, 0.5, 0.5, 0.5, 0.5]
  in  "Row Headers 1D [ ] - Table 7":string[](array[string])=["Text palette", "Append Phrase.vi", "Append Paragraph.vi", "Append Paragraph with Link [ ].vi", "Table palette", "Caption for table (not a VI)", "Append Table.vi", "Append Customized Table.vi", "Image palette", "Caption for image (not a VI)", "Header, Footer and Watermark palette", "Append Text HF.vi", "Append Page number HF.vi", "Append Watermark Text.vi", "Table of Contents palette", "Append Chapter bookmark.vi", "Append a Table of Contents.vi"]
  in  "Table properties - Table 8":T48={"Table position"=1, "SpacingBefore (points)"=12.0, "SpacingAfter (points)"=12.0} {"Table position" items=["LEFT", "CENTER", "RIGHT"]}
  in  "Text Data 2D [ ] - Table 8":string[][](array[string])=[["Not supported"], ["Not tested"], ["Tested"]]
  in  "Table columnWidth [ ] - Table 8":sgl[](array[numeric])=[0.5, 1.5]
  in  "Row  [ ] - Table 8":T56=[{"Row"={"From #"=0, "to #"=0}, "Cell [ ]"=[{"Text"={"Cell Alignment"=5, "Text rotation"=enum."None", "Line spacing"=enum."Select"}, "Cell Appearance"={"Border"=8, "Thickness"=0.5, "Color"=0, "BG"=15066597}, "HMerge"={"From"=-1, "to"=-1}, "VMerge"={"From"=-1, "to"=-1}, "Font"={"Name"="", "Size"=-1.0, "Color"=0, "Style"={"Bold"=FALSE, "Italic"=FALSE, "Underline"=FALSE, "Strikeout"=FALSE}, "Type"={"Type&direction"=enum."Select", "Embedded"=FALSE, "Encoding"=""}}}, {"Text"={"Cell Alignment"=4, "Text rotation"=enum."None", "Line spacing"=enum."Select"}, "Cell Appearance"={"Border"=5, "Thickness"=0.5, "Color"=0, "BG"=16777225}, "HMerge"={"From"=-1, "to"=-1}, "VMerge"={"From"=-1, "to"=-1}, "Font"={"Name"="", "Size"=-1.0, "Color"=0, "Style"={"Bold"=FALSE, "Italic"=FALSE, "Underline"=FALSE, "Strikeout"=FALSE}, "Type"={"Type&direction"=enum."Select", "Embedded"=FALSE, "Encoding"=""}}}]}, {"Row"={"From #"=1, "to #"=1}, "Cell [ ]"=[{"Text"={"Cell Alignment"=5, "Text rotation"=enum."None", "Line spacing"=enum."Select"}, "Cell Appearance"={"Border"=2, "Thickness"=0.5, "Color"=0, "BG"=10473471}, "HMerge"={"From"=-1, "to"=-1}, "VMerge"={"From"=-1, "to"=-1}, "Font"={"Name"="", "Size"=-1.0, "Color"=0, "Style"={"Bold"=FALSE, "Italic"=FALSE, "Underline"=FALSE, "Strikeout"=FALSE}, "Type"={"Type&direction"=enum."Select", "Embedded"=FALSE, "Encoding"=""}}}, {"Text"={"Cell Alignment"=4, "Text rotation"=enum."None", "Line spacing"=enum."Select"}, "Cell Appearance"={"Border"=3, "Thickness"=0.5, "Color"=0, "BG"=16777225}, "HMerge"={"From"=-1, "to"=-1}, "VMerge"={"From"=-1, "to"=-1}, "Font"={"Name"="", "Size"=-1.0, "Color"=0, "Style"={"Bold"=FALSE, "Italic"=FALSE, "Underline"=FALSE, "Strikeout"=FALSE}, "Type"={"Type&direction"=enum."Select", "Embedded"=FALSE, "Encoding"=""}}}]}, {"Row"={"From #"=2, "to #"=2}, "Cell [ ]"=[{"Text"={"Cell Alignment"=5, "Text rotation"=enum."None", "Line spacing"=enum."Select"}, "Cell Appearance"={"Border"=2, "Thickness"=0.5, "Color"=0, "BG"=16777224}, "HMerge"={"From"=-1, "to"=-1}, "VMerge"={"From"=-1, "to"=-1}, "Font"={"Name"="", "Size"=-1.0, "Color"=0, "Style"={"Bold"=FALSE, "Italic"=FALSE, "Underline"=FALSE, "Strikeout"=FALSE}, "Type"={"Type&direction"=enum."Select", "Embedded"=FALSE, "Encoding"=""}}}, {"Text"={"Cell Alignment"=4, "Text rotation"=enum."None", "Line spacing"=enum."Select"}, "Cell Appearance"={"Border"=3, "Thickness"=0.5, "Color"=0, "BG"=16777225}, "HMerge"={"From"=-1, "to"=-1}, "VMerge"={"From"=-1, "to"=-1}, "Font"={"Name"="", "Size"=-1.0, "Color"=0, "Style"={"Bold"=FALSE, "Italic"=FALSE, "Underline"=FALSE, "Strikeout"=FALSE}, "Type"={"Type&direction"=enum."Select", "Embedded"=FALSE, "Encoding"=""}}}]}]
  in  "Row Headers 1D [ ] - Table 8":string[](array[string])=[" ", "  ", " "]
  # "C:\\Program Files\\National Instruments\\LabVIEW 2009\\vi.lib\\Exaprom PDF\\Examples\\Images\\Palette Table\\Append Table VI.jpg\nC:\\Program Files\\National Instruments\\LabVIEW 2009\\vi.lib\\Exaprom PDF\\Examples\\Images\\Palette Table\\Table Standard Format.jpg"
  # "Table Standard Format"
  # "A"
  # "Not available in the Run Time System"
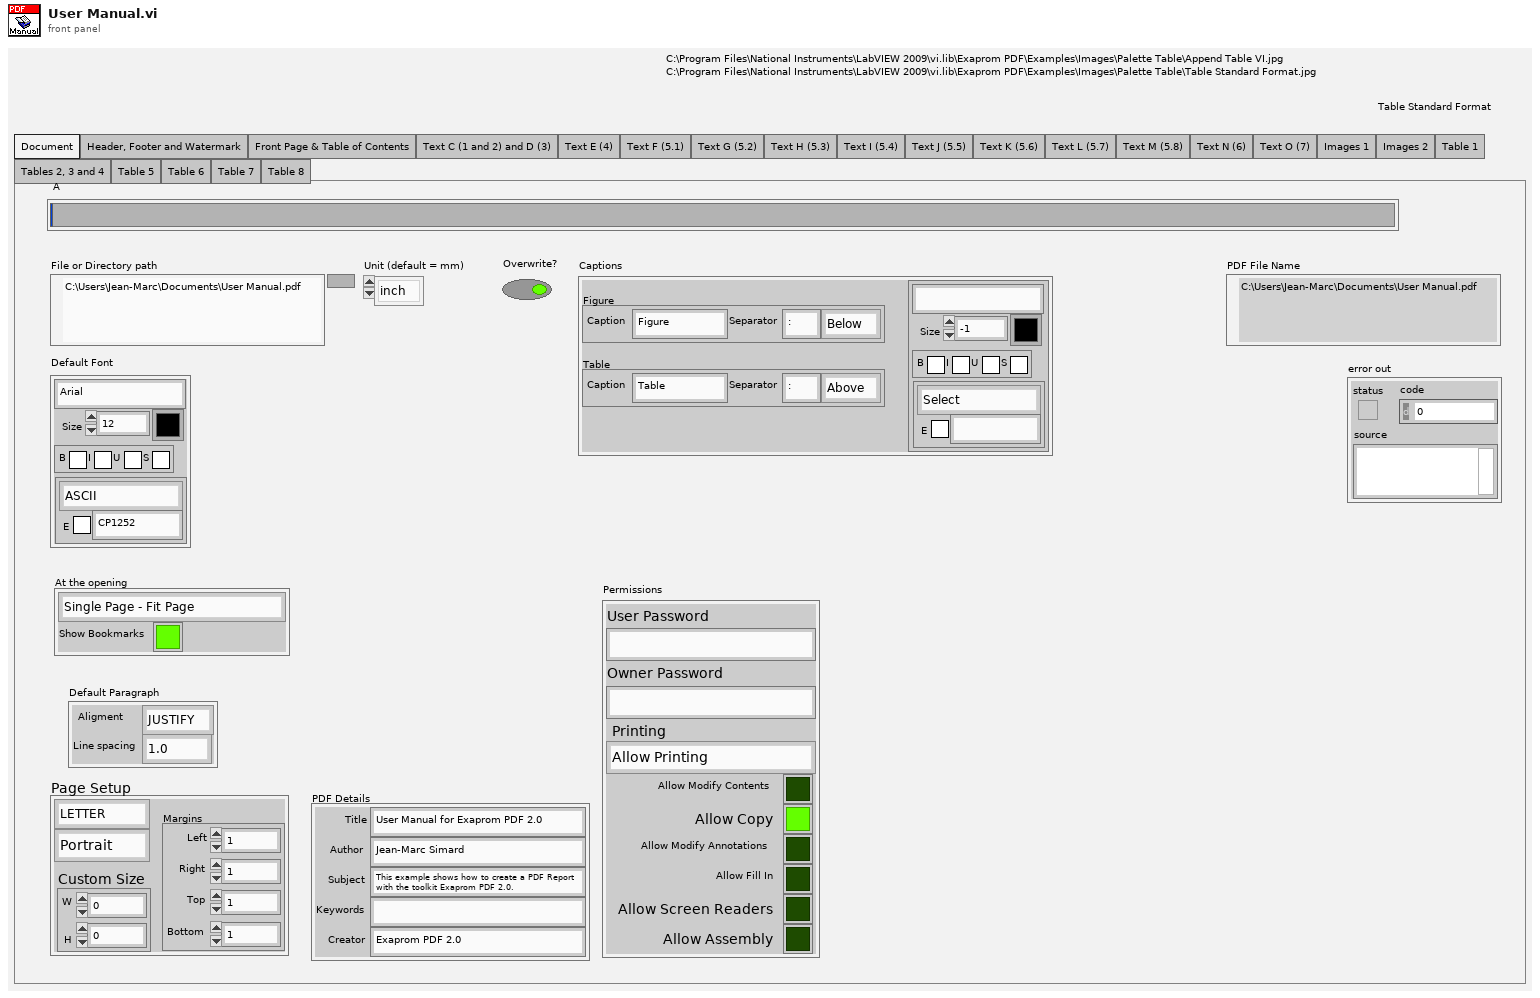
[diagram p1: front panel]
types:
  T1 = enum32{"Document", "Header, Footer and Watermark", "Front Page & Table of Contents", "Text C (1 and 2) and D (3)", "Text E (4)", "Text F (5.1)", "Text G (5.2)", "Text H (5.3)", "Text I (5.4)", "Text J (5.5)", "Text K (5.6)", "Text L (5.7)", "Text M (5.8)", "Text N (6)", "Text O (7)", "Images 1", "Images 2", "Table 1", "Tables 2, 3 and 4", "Table 5", "Table 6", "Table 7", "Table 8"}
  T2 = typedef "Page setup.ctl" = cluster{"Page Size":T3, "Orientation":T4, "Custom Size":T5, "Margins":T6}
  T3 = typedef "Page size.ctl" = i32
  T4 = typedef "Page Orientation.ctl" = enum16{"Portrait", "Landscape"}
  T5 = typedef "Page Layout Custom.ctl" = cluster{"Width":sgl, "Height":sgl}
  T6 = typedef "Page margins.ctl" = cluster{"Left":sgl, "Right":sgl, "Top":sgl, "Bottom":sgl}
  T7 = typedef "Defaut Paragraphe and Line Spacing.ctl" = cluster{" Aligment":T8, "Line spacing":T9}
  T8 = typedef "Texte alignement.ctl" = enum16{"Select", "CENTER", "JUSTIFY", "LEFT", "RIGHT"}
  T9 = typedef "Line spacing.ctl" = enum16{"Select", "1.0", "1.5", "2.0"}
  T10 = typedef "PDF Details.ctl" = cluster{"Title":string, "Author":string, "Subject":string, "Keywords":string, "Creator":string}
  T11 = typedef "Font complete cluster.ctl" = cluster{"Name":string, "Size":T12, "Color":T13, "Style":cluster{"Bold":bool, "Italic":bool, "Underline":bool, "Strikeout":bool}, "Type":T14}
  T12 = typedef "Font size.ctl" = sgl
  T13 = typedef "Font color.ctl" = u32
  T14 = typedef "Type and encoding.ctl" = cluster{"Type&direction":T15, "Embedded":bool, "Encoding":string}
  T15 = typedef "Type and run direction.ctl" = enum16{"Select", "ASCII", "UTF-16", "UTF-16 (default)", "UTF-16 (LTR)", "UTF-16 (RTL)"}
  T16 = typedef "Captions.ctl" = cluster{"Figure":T17, "Table":T17, "Font":T11}
  T17 = typedef "Image or Table Caption.ctl" = cluster{"Caption":string, "Separator":string, "Position":enum16{"Above", "Below"}}
  T18 = typedef "Unit.ctl" = enum16{"inch", "mm"}
  T19 = typedef "File Permission Parameters.ctl" = cluster{"User Password":string, "Owner Password":string, "Printing":enum16{"Allow Printing", "Allow Degraded Printing", "Don't Allow Printing"}, "Allow Modify Contents":bool, "Allow Copy":bool, "Allow Modify Annotations":bool, "Allow Fill In ":bool, "Allow Screen Readers":bool, "Allow Assembly":bool}
  T20 = typedef "At the opening.ctl" = cluster{"Page":u16, "Show Bookmarks":bool}
  T21 = typedef "Header or Footer  Page # cluster.ctl" = cluster{"Start at page":i32, "Start with #":i32, "Cell Alignment":T22, "Page #":T23, "Font":T24}
  T22 = typedef "Cell Alignment 20px.ctl" = u16
  T23 = typedef "Page number.ctl" = cluster{"Text 1":string, "Text 2":string, "Text 3":string}
  T24 = typedef "Font complete cluster horizontal.ctl" = cluster{"Name":string, "Size":T12, "Color":T13, "Style":cluster{"Bold":bool, "Italic":bool, "Underline":bool, "Strikeout":bool}, "Type":T14}
  T25 = typedef "Header or Footer Line cluster.ctl" = cluster{"H/F Line":T26, "Thickness (point)":sgl, " Colour":u32}
  T26 = typedef "Header Footer Line.ctl" = enum16{"No line", "Horizontal line"}
  T27 = typedef "Header or Footer  Text cluster.ctl" = cluster{"Start at page":i32, "Cell Alignment":T22, "Line spacing":T9, "Text":string, "Font complete":T24, "Link":string}
  T28 = typedef "Watermark Image Cluster.ctl" = cluster{"Image path":path, "Opacity (%)":sgl, "Postion":cluster{"Position":T29, "X":sgl, "Y":sgl}, "Automatic":bool, "Scale(%)":sgl, "Rotate(°)":sgl}
  T29 = typedef "Watermark Position.ctl" = enum16{"Absolute", "Center (page)", "Center (text section)"}
  T30 = typedef "Watermark Text Cluster.ctl" = cluster{"Text ":string, "Opacity (%)":sgl, "Position":cluster{"Position":T29, "X":sgl, "Y":sgl}, "Automatic":bool, "Font":cluster{"Font Name":string, "Size":T12, "Color":T13}, "Alignment":T31, "Rotate(°)":sgl}
  T31 = typedef "Header footer horiz alignment.ctl" = enum16{"Left", "Center", "Right"}
  T32 = typedef "Header or Footer  Image cluster.ctl" = cluster{"Start at page":i32, "Cell Alignment":T22, "Path":path, "Image (%)":sgl, "Link":string}
  T33 = typedef "Text and hyperlink [ ].ctl" = T34[]
  T34 = typedef "Text from String of File and hyperlink.ctl" = cluster{"Text":cluster{"Text":string, "Path":path, "Font complete":T24}, "Link":cluster{"Hyperlink":string, "Font complete":T24}, "Paragraphe":T7, "Indentation":T35}
  T35 = typedef "Paragraph indentation.ctl" = cluster{"Left":sgl, "Right":sgl}
  T36 = typedef "PDF file to concatenate.ctl" = cluster{"Path":path, "Pages":string, "Password":string}
  T37 = typedef "Image alignment and position.ctl" = cluster{"Alignment":T38, "X ":sgl, "Y":sgl, "Indentation":sgl}
  T38 = typedef "Image aligment.ctl" = enum16{"Absolute (X,Y)", "Left", "Center", "Right", "Left (textwrap)", "Right (textwrap)"}
  T39 = typedef "Image border.ctl" = cluster{"Show?":bool, "Thickness (point)":sgl, "Color":u32}
  T40 = cluster{"Scale (%)":sgl, "Position":T37, "Border":T39}
  T41 = typedef "Row Predefined borders cluster.ctl" = cluster{"Borders":T42, "Header":cluster{"Thickness":sgl, "Line":u32, "Background ":u32}, "Data":cluster{"Thickness":sgl, "Line":u32, "Background ":u32}}
  T42 = typedef "Row Predefined borders.ctl" = u16
  T43 = typedef "Image Scale.ctl" = sgl
  T44 = cluster{"Image name":string, "Path":path, "Scale":T43}[]
  T45 = typedef "Cell Font, type, Alignment and LS V2.ctl" = cluster{"Cell Type, Alignment and LS":T46, "Font":T11}
  T46 = typedef "Cell Type, Alignment and LS.ctl" = cluster{"Cell Alignment":T22, "Text rotation":T47, "Line spacing":T9}
  T47 = typedef "Text vertical arrangement.ctl" = enum16{"None", "Clockwise", "Counterclockwise"}
  T48 = typedef "Table properties.ctl" = cluster{"Table position":T49, "SpacingBefore (points)":sgl, "SpacingAfter (points)":sgl}
  T49 = typedef "Table position.ctl" = i32
  T50 = typedef "Simplified Table Row Borders [ ].ctl" = T51[]
  T51 = typedef "Simplified Table Row Borders.ctl" = cluster{"Row":cluster{"#":i16, "to #":i16}, "Line":cluster{"Thickness":sgl, "Color":u32}, "Column Borders [ ]":T52}
  T52 = typedef "Border and BG Color [ ].ctl" = T53[]
  T53 = typedef "Border and BG Color.ctl" = cluster{"Cell Border":T54, "BG":u32}
  T54 = typedef "Cell Border 20 px.ctl" = u16
  T55 = typedef "Row Back Ground color Datas.ctl" = cluster{"color":u32, "at each":i16}
  T56 = typedef "Table Appearance and Font Row [ ].ctl" = T57[]
  T57 = typedef "One Row Appearance.ctl" = cluster{"Row":T58, "Cell [ ]":T59[]}
  T58 = typedef "Row from to.ctl" = cluster{"From #":i16, "to #":i16}
  T59 = typedef "Cell, Alignment, LS and Font - hide Vmerge.ctl" = cluster{"Text":T46, "Cell Appearance":T60, "HMerge":T61, "VMerge":T62, "Font":T11}
  T60 = typedef "Cell Appearance.ctl" = cluster{"Border":T54, "Thickness":sgl, "Color":u32, "BG":u32}
  T61 = typedef "Merge Horizontal.ctl" = cluster{"From":i8, "to":i8}
  T62 = typedef "Merge Vertical.ctl" = cluster{"From":i8, "to":i8}
  T63 = typedef "LVPointTypeDef.ctl" = cluster{"Horizontal":i16, "Vertical":i16}
  T64 = typedef "Chapter.ctl" = enum16{"Chapter - level 1", "Chapter - level 2", "Chapter - level 3", "Chapter - level 4"}
  T65 = typedef "Header or Footer.ctl" = enum16{"Header", "Footer"}
  T66 = typedef "Image Size Block Diagram.ctl" = cluster{"Maximum Width":i32, "Maximum Height":i32}
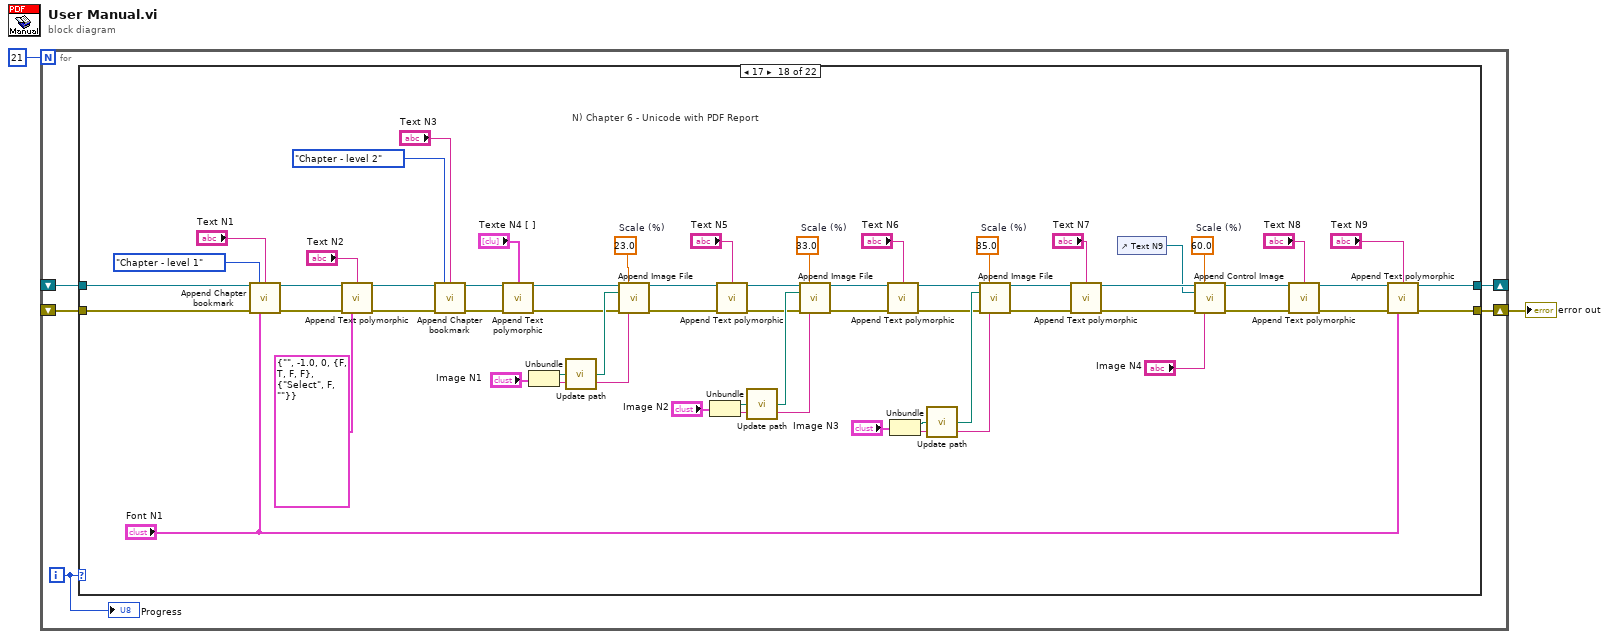
[diagram p0: block diagram]
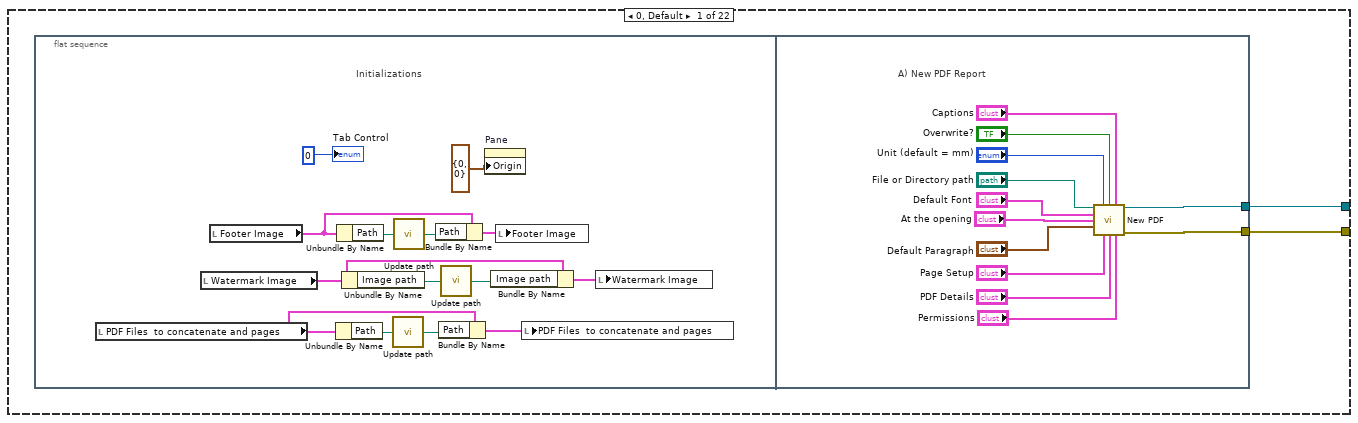
[diagram p2: hidden frame]
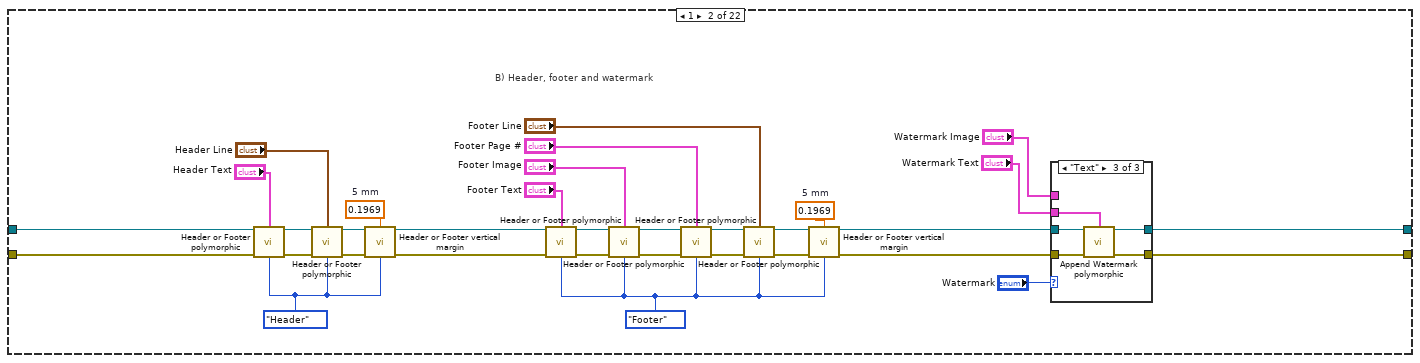
[diagram p3: hidden frame]
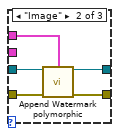
[diagram p5: hidden frame]
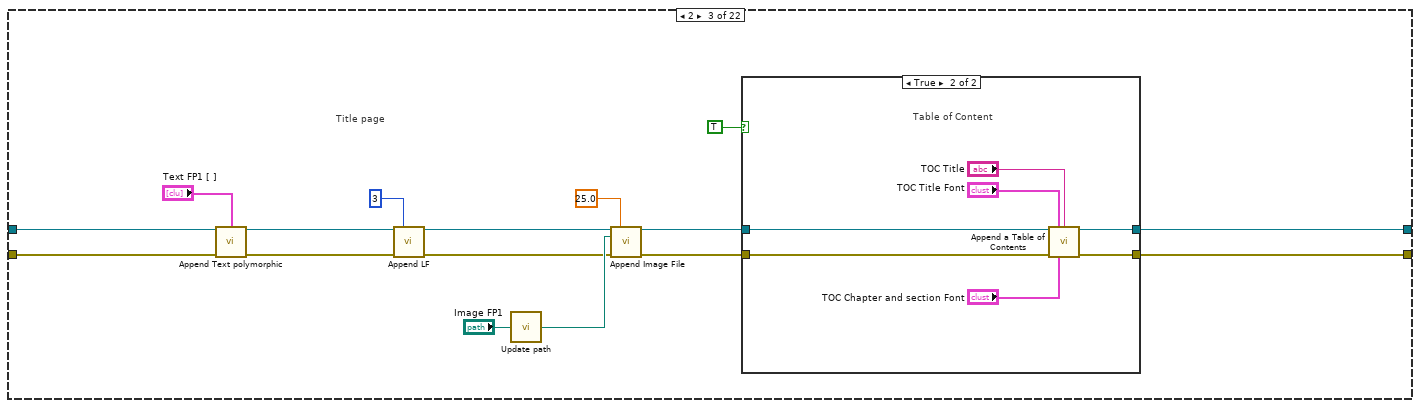
[diagram p6: hidden frame]
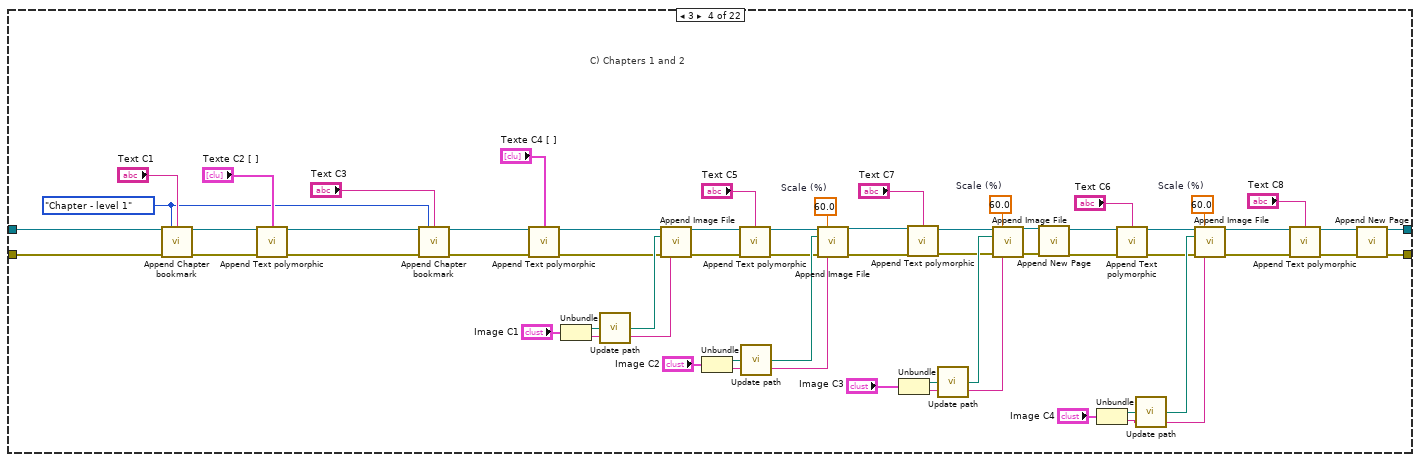
[diagram p8: hidden frame]
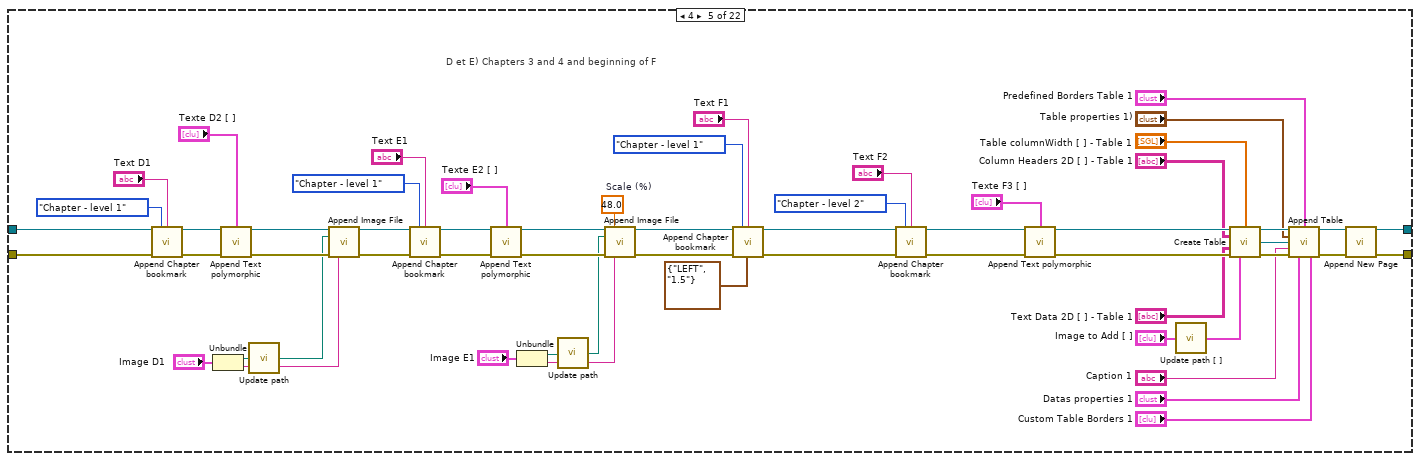
[diagram p9: hidden frame]
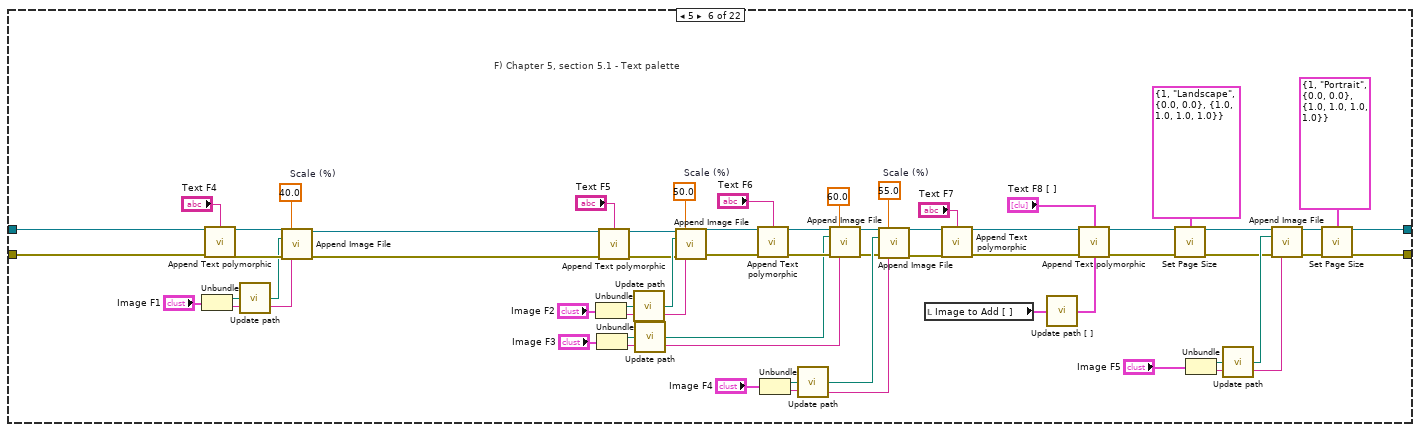
[diagram p10: hidden frame]
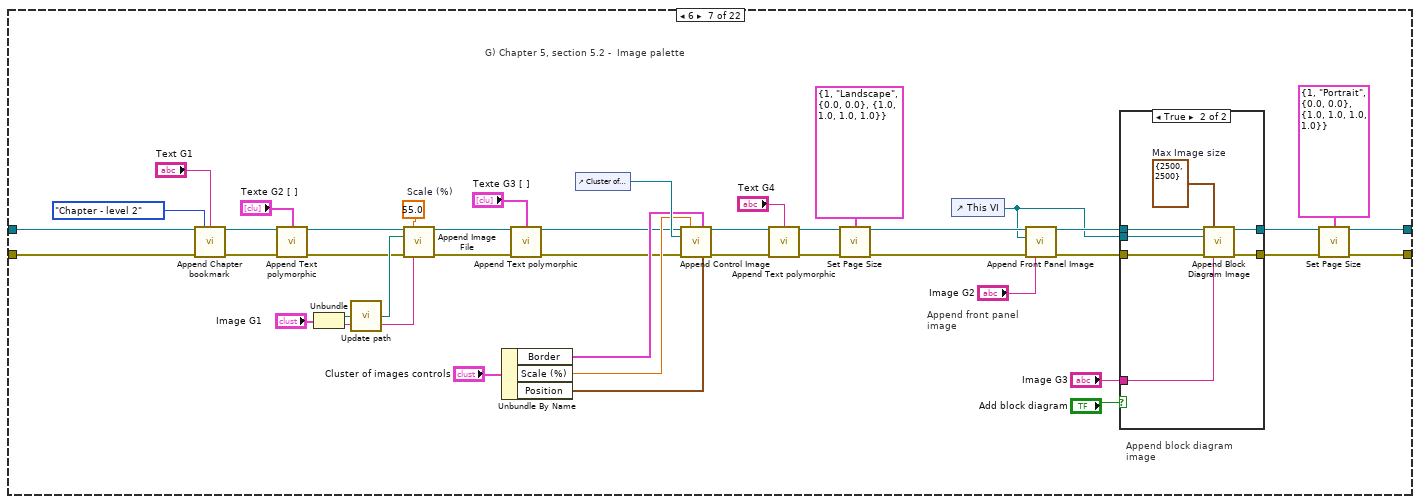
[diagram p11: hidden frame]
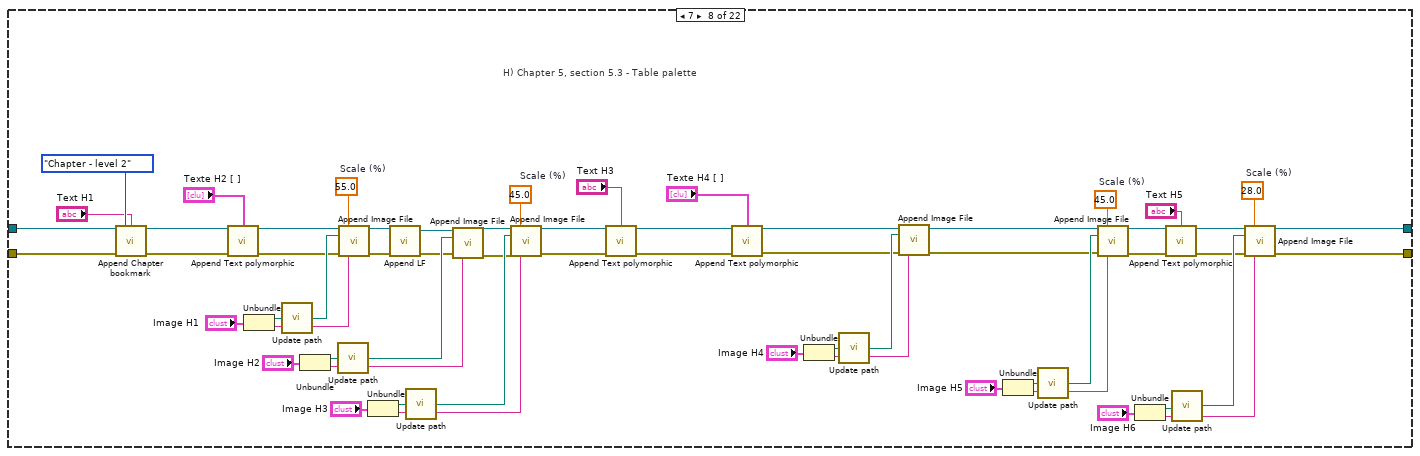
[diagram p13: hidden frame]
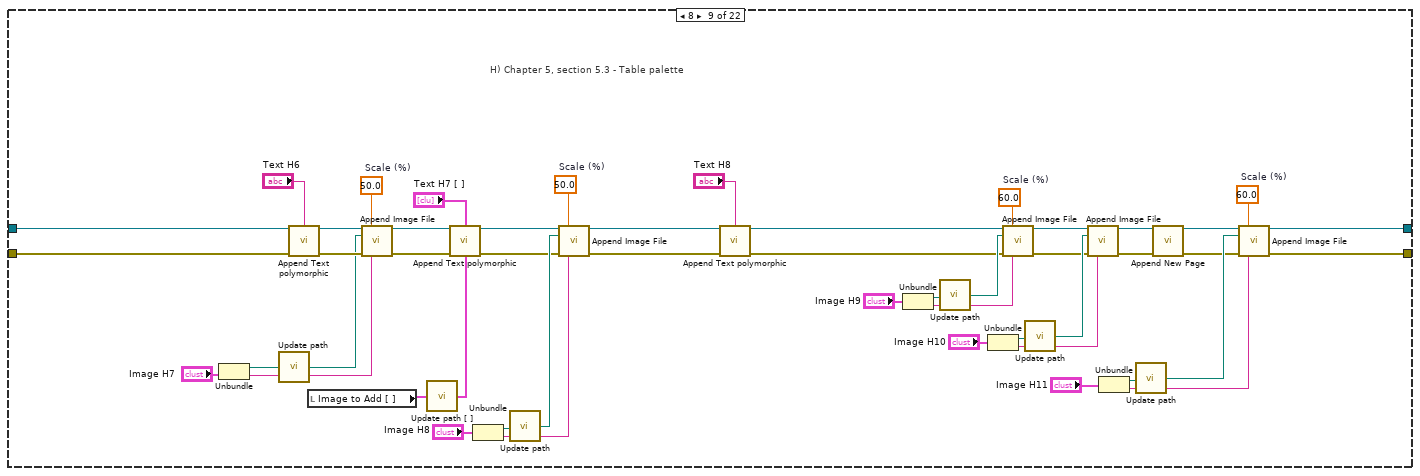
[diagram p14: hidden frame]
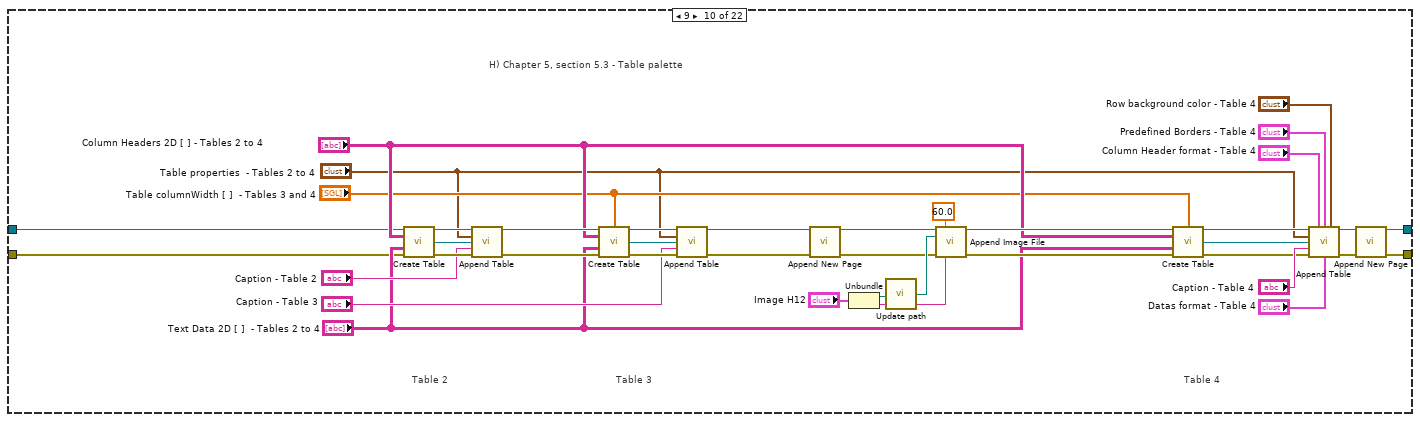
[diagram p15: hidden frame]
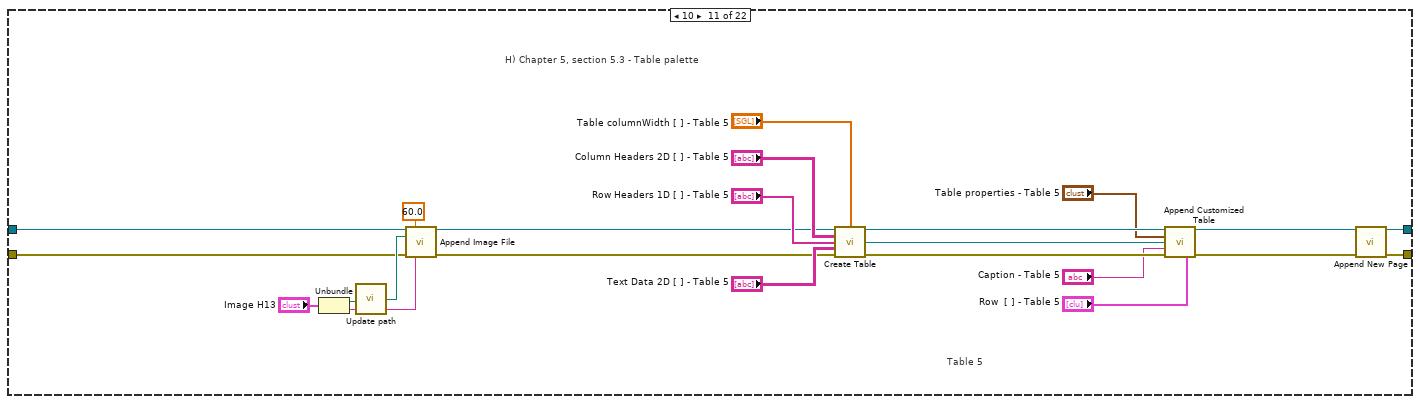
[diagram p16: hidden frame]
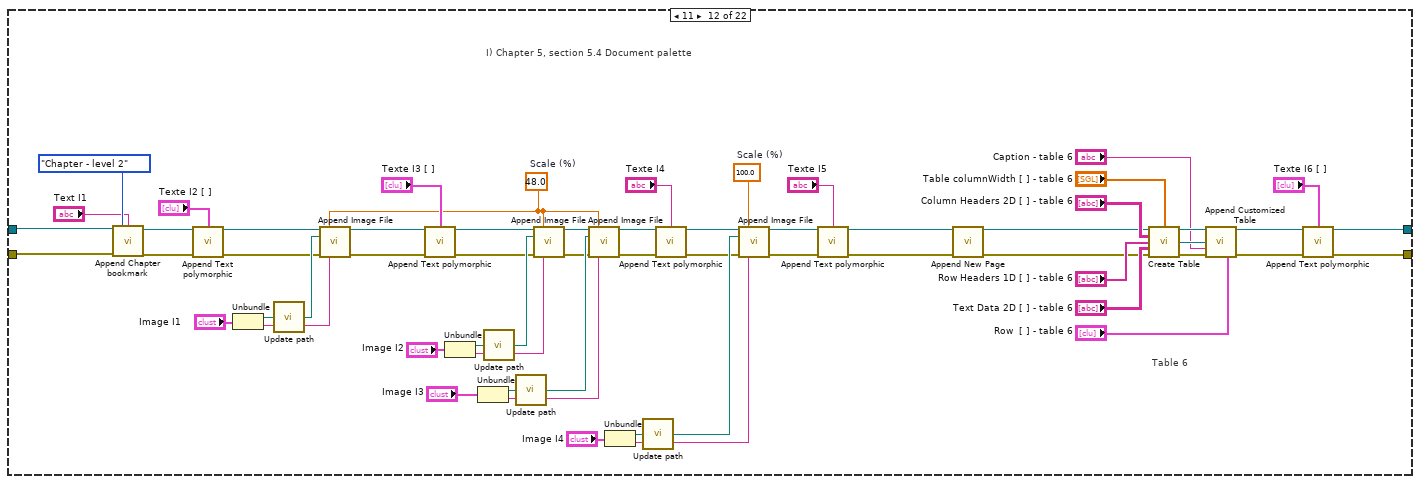
[diagram p17: hidden frame]
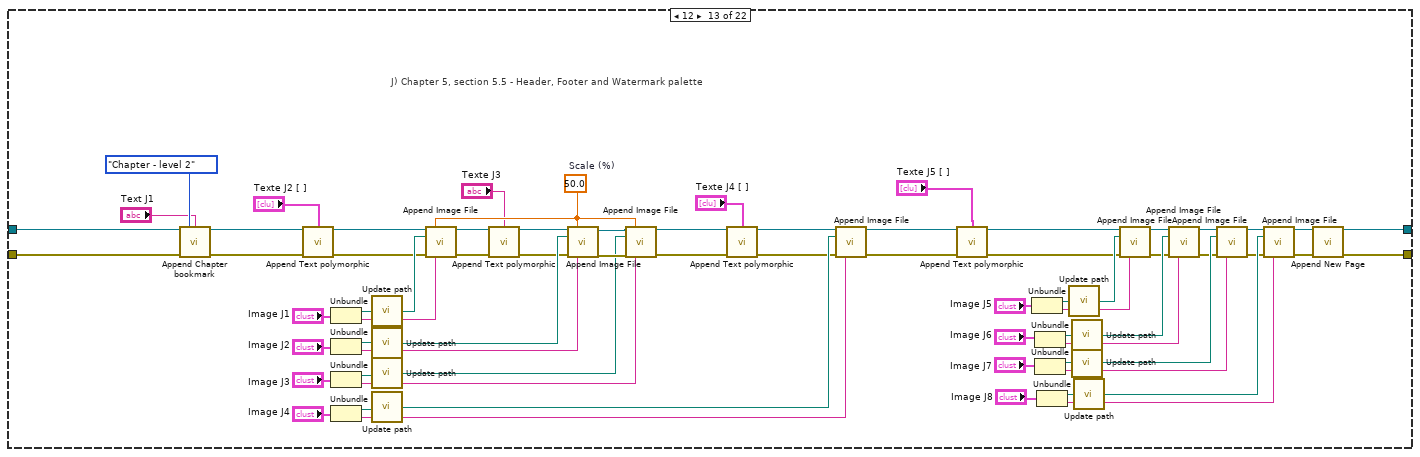
[diagram p18: hidden frame]
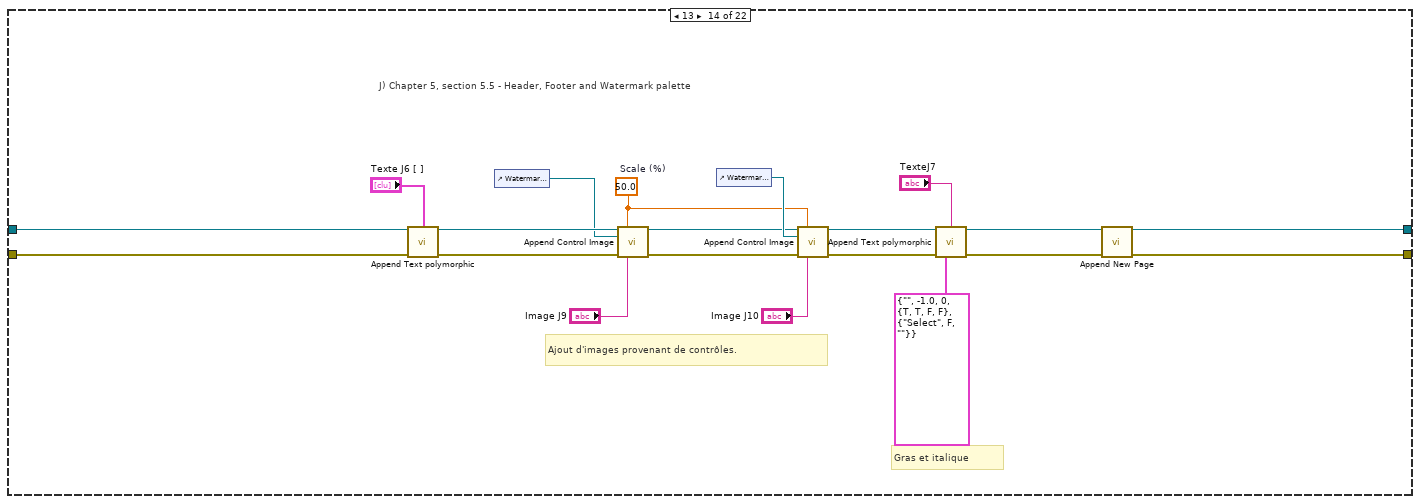
[diagram p19: hidden frame]
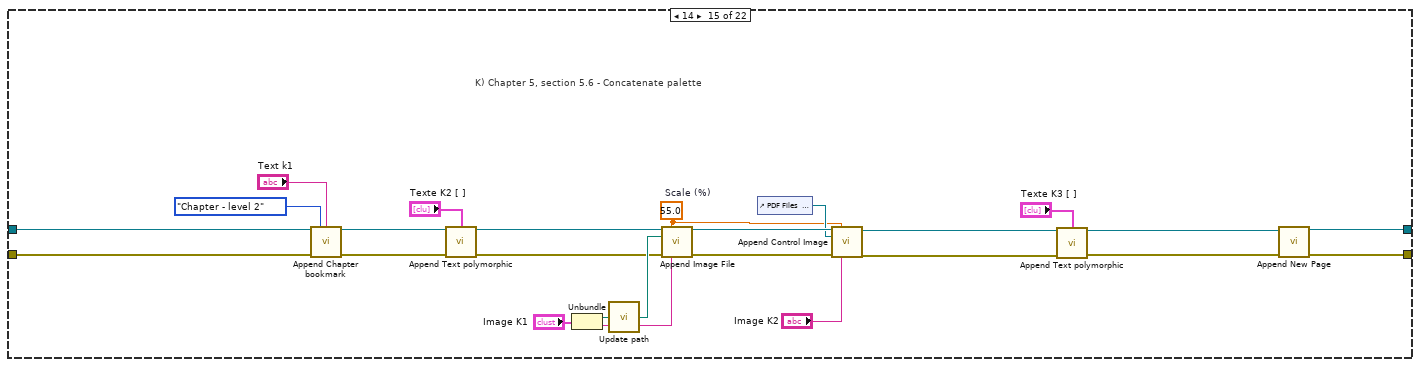
[diagram p20: hidden frame]
diagram:
  n1 = for {
    N: 21 -> [_]
    shift-right: [w6] -> _
    shift-left: _ -> [w5]
    shift-right: [w7] -> w2
    shift-left: _ -> [w4]
    i -> [w3]
    n2 = case shown="17" w3 {
      tunnel: [w9 w65 w84 w162 w165 w280 w287 w341 w424 w443 w503 w510 w571 w649 w666 w680 w725 w747 w796 w851 _ _] -> w6
      tunnel: [w8 w66 w85 w161 w164 w279 w288 w342 w423 w442 w502 w511 w570 w650 w665 w678 w723 w748 w797 w850 w854 w856] -> w7
      tunnel: w5 -> [_ w68 w93 w163 w201 w224 w282 w343 w396 w445 w481 w504 w564 w652 w653 w719 w727 w751 w827 w841 w852 _]
      tunnel: w4 -> [_ w67 w94 w116 w200 w223 w281 w344 w395 w444 w482 w505 w565 w651 w654 w718 w728 w750 w828 w840 w853 w856]
      frame 0, Default {
        n3 = flat-sequence {
          tunnel: [w34] -> w9
          tunnel: [w33] -> w8
          frame #0 {
            # "Initializations"
            n4 = local read "PDF Files  to concatenate and pages"() -> (w13:T36)
            n5 = local read "Watermark Image"() -> (w14:T28)
            n6 = local read "Footer Image"() -> (w21:T32)
            n7 = Unbundle By Name(w13) -> ("Path"=w11:path)
            n8 = Unbundle By Name(w21) -> ("Path"=w19:path)
            n9 = Unbundle By Name(w14) -> ("Image path"=w16:path)
            n10 = call <userlib>:"Update path.vi"("Path IN"=w11) -> ("Path OUT"=w12:path)  [unwired: 1 in, 2 out]
            n11 = call <userlib>:"Update path.vi"("Path IN"=w19) -> ("Path OUT"=w20:path)  [unwired: 1 in, 2 out]
            n12 = Bundle By Name(cluster=w21, "Path"=w20) -> (w18:T32)
            n13 = Bundle By Name(cluster=w13, "Path"=w12) -> (w10:T36)
            n14 = call <userlib>:"Update path.vi"("Path IN"=w16) -> ("Path OUT"=w15:path)  [unwired: 1 in, 2 out]
            n15 = property on="Pane" class="Pane"("Origin"=T63 {"Horizontal"=0, "Vertical"=0}) -> ()  [unwired: 2 in, 2 out]
            n16 = Bundle By Name(cluster=w14, "Image path"=w15) -> (w17:T28)
            n17 = local write "Footer Image"(w18) -> ()
            n18 = local write "PDF Files  to concatenate and pages"(w10) -> ()
            n19 = local write "Watermark Image"(w17) -> ()
            "Tab Control" <- 0
          }
          frame #1 {
            # "A) New PDF Report"
            n20 = call <userlib>:"New PDF.vi"("PDF Path"="File or Directory path", "Unit (default = mm)"="Unit (default = mm)", "Overwrite?"="Overwrite?", "Captions"="Captions", "Default Font"="Default Font", "At the opening"="At the opening", "Default Paragraph"="Default Paragraph", "Page Setup"="Page Setup", "PDF Details"="PDF Details", "Permissions"="Permissions") -> ("PDF Report"=w34:refnum<class "PDF Report Class.lvclass">, "error out"=w33:errorcluster)  [unwired: 1 in, 3 out]
          }
        }
      }
      frame 1 {
        w64 = 0.1969  # 5 mm
        w63 = 0.1969  # 5 mm
        w62 = Header_or_Footer."Header" ("Position")
        w61 = Header_or_Footer."Footer" ("Position")
        # "B) Header, footer and watermark"
        n21 = call-poly <userlib>:"Header or Footer polymorphic.vi"("PDF Report IN"=w68, "Header or footer"="Header Text", "error in (no error)"=w67, "Position"=w62) -> ("PDF Report OUT"=w50:refnum<class "PDF Report Class.lvclass">, "error out"=w49:errorcluster)  [unwired: 10 out]
        n22 = call-poly <userlib>:"Header or Footer polymorphic.vi"("PDF Report IN"=w50, "H/F Line"="Header Line", "error in (no error)"=w49, "Position"=w62) -> ("PDF Report OUT"=w42:refnum<class "PDF Report Class.lvclass">, "error out"=w55:errorcluster)  [unwired: 1 in, 9 out]
        n23 = call <userlib>:"Header or Footer vertical margin.vi"("PDF Report IN"=w42, "Vertical margin"=w63, "error in (no error)"=w55, "Position"=w62) -> ("PDF Report OUT"=w54:refnum<class "PDF Report Class.lvclass">, "error out"=w58:errorcluster)  [unwired: 10 out]
        n24 = call-poly <userlib>:"Header or Footer polymorphic.vi"("PDF Report IN"=w54, "Header or footer"="Footer Text", "error in (no error)"=w58, "Position"=w61) -> ("PDF Report OUT"=w45:refnum<class "PDF Report Class.lvclass">, "error out"=w48:errorcluster)  [unwired: 10 out]
        n25 = call-poly <userlib>:"Header or Footer polymorphic.vi"("PDF Report IN"=w45, "Header or footer"="Footer Image", "error in (no error)"=w48, "Position"=w61) -> ("PDF Report OUT"=w44:refnum<class "PDF Report Class.lvclass">, "error out"=w47:errorcluster)  [unwired: 10 out]
        n26 = call-poly <userlib>:"Header or Footer polymorphic.vi"("PDF Report IN"=w44, "Header or footer"="Footer Page #", "error in (no error)"=w47, "Position"=w61) -> ("PDF Report OUT"=w43:refnum<class "PDF Report Class.lvclass">, "error out"=w46:errorcluster)  [unwired: 10 out]
        n27 = call-poly <userlib>:"Header or Footer polymorphic.vi"("PDF Report IN"=w43, "H/F Line"="Footer Line", "error in (no error)"=w46, "Position"=w61) -> ("PDF Report OUT"=w57:refnum<class "PDF Report Class.lvclass">, "error out"=w56:errorcluster)  [unwired: 1 in, 9 out]
        n28 = call <userlib>:"Header or Footer vertical margin.vi"("PDF Report IN"=w57, "Vertical margin"=w64, "error in (no error)"=w56, "Position"=w61) -> ("PDF Report OUT"=w60:refnum<class "PDF Report Class.lvclass">, "error out"=w59:errorcluster)  [unwired: 10 out]
        n29 = case shown="\"Text\"" "Watermark" {
          tunnel: w59 -> [w69 w75 w80]
          tunnel: w60 -> [w70 w74 w79]
          tunnel: [w70 w73 w78] -> w65
          tunnel: [w69 w72 w77] -> w66
          tunnel: "Watermark Text" -> [_ _ w76]
          tunnel: "Watermark Image" -> [_ w71 _]
          frame "none", Default {
          }
          frame "Image" {
            n30 = call-poly <userlib>:"Append Watermark polymorphic.vi"("PDF Report IN"=w74, "Watermark Image"=w71, "error in (no error)"=w75) -> ("PDF Report OUT"=w73:refnum<class "PDF Report Class.lvclass">, "error out"=w72:errorcluster)  [unwired: 1 in, 10 out]
          }
          frame "Text" {
            n31 = call-poly <userlib>:"Append Watermark polymorphic.vi"("PDF Report IN"=w79, "Watermark Text"=w76, "error in (no error)"=w80) -> ("PDF Report OUT"=w78:refnum<class "PDF Report Class.lvclass">, "error out"=w77:errorcluster)  [unwired: 1 in, 10 out]
          }
        }
      }
      frame 2 {
        # "Title page"
        n32 = call-poly <userlib>:"Append Text polymorphic.vi"("PDF Report"=w93, "Text [ ]"="Text FP1 [ ]", "error in (no error)"=w94) -> ("PDF Report duplicate"=w95:refnum<class "PDF Report Class.lvclass">, "error out"=w88:errorcluster)  [unwired: 1 in, 10 out]
        n33 = call <userlib>:"Append LF.vi"("PDF Report IN"=w95, "Number of LF (default 1)"=u8 3, "error in (no error)"=w88) -> ("PDF Report duplicate"=w89:refnum<class "PDF Report Class.lvclass">, "error out"=w87:errorcluster)  [unwired: 11 in]
        n34 = call <userlib>:"Update path.vi"("Path IN"="Image FP1") -> ("Path OUT"=w91:path)  [unwired: 1 in, 2 out]
        n35 = call <userlib>:"Append Image File.vi"("PDF Report IN"=w89, "Scale (%)"=sgl 25.0, "Image path"=w91, "error in (no error)"=w87) -> ("PDF Report OUT"=w83:refnum<class "PDF Report Class.lvclass">, "error out"=w82:errorcluster)  [unwired: 8 in, 2 out]
        n36 = case shown="True" TRUE {
          tunnel: [w97 w105] -> w85
          tunnel: [w98 w104] -> w84
          tunnel: w83 -> [w98 w103]
          tunnel: w82 -> [w97 w102]
          frame False {
          }
          frame True {
            # "Table of Content"
            n37 = call <userlib>:"Append a Table of Contents.vi"("PDF Report IN"=w103, "Title Font"="TOC Title Font", "Title"="TOC Title", "error in (no error)"=w102, "Chapter and section Font"="TOC Chapter and section Font") -> ("PDF Report OUT"=w104:refnum<class "PDF Report Class.lvclass">, "error out"=w105:errorcluster)  [unwired: 9 in]
          }
        }
      }
      frame 3 {
        w108 = Chapter."Chapter - level 1" ("Chapter or section")
        w146 = sgl 60.0  # Scale (%)
        w151 = sgl 60.0  # Scale (%)
        w155 = sgl 60.0  # Scale (%)
        # "C) Chapters 1 and 2"
        n38 = call <userlib>:"Append Chapter bookmark.vi"("PDF Report"=w163, "Chapter or section"=w108, "Title"="Text C1", "error in (no error)"=w116) -> ("PDF Report duplicate"=w118:refnum<class "PDF Report Class.lvclass">, "error out"=w117:errorcluster)  [unwired: 10 in]
        n39 = call-poly <userlib>:"Append Text polymorphic.vi"("PDF Report"=w118, "Text [ ]"="Texte C2 [ ]", "error in (no error)"=w117) -> ("PDF Report duplicate"=w114:refnum<class "PDF Report Class.lvclass">, "error out"=w113:errorcluster)  [unwired: 1 in, 10 out]
        n40 = call <userlib>:"Append Chapter bookmark.vi"("PDF Report"=w114, "Chapter or section"=w108, "Title"="Text C3", "error in (no error)"=w113) -> ("PDF Report duplicate"=w109:refnum<class "PDF Report Class.lvclass">, "error out"=w112:errorcluster)  [unwired: 10 in]
        n41 = call-poly <userlib>:"Append Text polymorphic.vi"("PDF Report"=w109, "Text [ ]"="Texte C4 [ ]", "error in (no error)"=w112) -> ("PDF Report duplicate"=w110:refnum<class "PDF Report Class.lvclass">, "error out"=w111:errorcluster)  [unwired: 1 in, 10 out]
        n42 = Unbundle("Image C1") -> ("Nom"=w138:path, "Légende"=w137:string)
        n43 = call <userlib>:"Update path.vi"("Path IN"=w138) -> ("Path OUT"=w139:path)  [unwired: 1 in, 2 out]
        n44 = call <userlib>:"Append Image File.vi"("PDF Report IN"=w110, "Image path"=w139, "error in (no error)"=w111, "Caption"=w137) -> ("PDF Report OUT"=w132:refnum<class "PDF Report Class.lvclass">, "error out"=w135:errorcluster)  [unwired: 3 in, 7 out]
        n45 = Unbundle("Image C2") -> ("Nom"=w153:path, "Légende"=w156:string)
        n46 = call-poly <userlib>:"Append Text polymorphic.vi"("PDF Report"=w132, "Text"="Text C5", "error in (no error)"=w135) -> ("PDF Report duplicate"=w133:refnum<class "PDF Report Class.lvclass">, "error out"=w134:errorcluster)  [unwired: 5 in, 6 out]
        n47 = call <userlib>:"Update path.vi"("Path IN"=w153) -> ("Path OUT"=w152:path)  [unwired: 1 in, 2 out]
        n48 = call <userlib>:"Append Image File.vi"("PDF Report IN"=w133, "Scale (%)"=w155, "Image path"=w152, "error in (no error)"=w134, "Caption"=w156) -> ("PDF Report OUT"=w128:refnum<class "PDF Report Class.lvclass">, "error out"=w129:errorcluster)  [unwired: 2 in, 7 out]
        n49 = Unbundle("Image C3") -> ("Nom"=w150:path, "Légende"=w147:string)
        n50 = call-poly <userlib>:"Append Text polymorphic.vi"("PDF Report"=w128, "Text"="Text C7", "error in (no error)"=w129) -> ("PDF Report duplicate"=w126:refnum<class "PDF Report Class.lvclass">, "error out"=w127:errorcluster)  [unwired: 5 in, 6 out]
        n51 = call <userlib>:"Update path.vi"("Path IN"=w150) -> ("Path OUT"=w148:path)  [unwired: 1 in, 2 out]
        n52 = call <userlib>:"Append Image File.vi"("PDF Report IN"=w126, "Scale (%)"=w151, "Image path"=w148, "error in (no error)"=w127, "Caption"=w147) -> ("PDF Report OUT"=w119:refnum<class "PDF Report Class.lvclass">, "error out"=w120:errorcluster)  [unwired: 2 in, 7 out]
        n53 = call <userlib>:"Append New Page.vi"("PDF Report"=w119, "error in (no error)"=w120) -> ("PDF Report duplicate"=w122:refnum<class "PDF Report Class.lvclass">, "error OUT"=w121:errorcluster)  [unwired: 12 out]
        n54 = Unbundle("Image C4") -> ("Nom"=w142:path, "Légende"=w140:string)
        n55 = call-poly <userlib>:"Append Text polymorphic.vi"("PDF Report"=w122, "Text"="Text C6", "error in (no error)"=w121) -> ("PDF Report duplicate"=w123:refnum<class "PDF Report Class.lvclass">, "error out"=w124:errorcluster)  [unwired: 5 in, 6 out]
        n56 = call <userlib>:"Update path.vi"("Path IN"=w142) -> ("Path OUT"=w141:path)  [unwired: 1 in, 2 out]
        n57 = call <userlib>:"Append Image File.vi"("PDF Report IN"=w123, "Scale (%)"=w146, "Image path"=w141, "error in (no error)"=w124, "Caption"=w140) -> ("PDF Report OUT"=w145:refnum<class "PDF Report Class.lvclass">, "error out"=w144:errorcluster)  [unwired: 2 in, 7 out]
        n58 = call-poly <userlib>:"Append Text polymorphic.vi"("PDF Report"=w145, "Text"="Text C8", "error in (no error)"=w144) -> ("PDF Report duplicate"=w157:refnum<class "PDF Report Class.lvclass">, "error out"=w158:errorcluster)  [unwired: 5 in, 6 out]
        n59 = call <userlib>:"Append New Page.vi"("PDF Report"=w157, "error in (no error)"=w158) -> ("PDF Report duplicate"=w162:refnum<class "PDF Report Class.lvclass">, "error OUT"=w161:errorcluster)  [unwired: 12 out]
      }
      frame 4 {
        w212 = sgl 48.0  # Scale (%)
        # "D et E) Chapters 3 and 4 and beginning of F"
        n60 = call <userlib>:"Append Chapter bookmark.vi"("PDF Report"=w201, "Chapter or section"=Chapter."Chapter - level 1", "Title"="Text D1", "error in (no error)"=w200) -> ("PDF Report duplicate"=w202:refnum<class "PDF Report Class.lvclass">, "error out"=w199:errorcluster)  [unwired: 10 in]
        n61 = Unbundle("Image D1") -> ("Nom"=w209:path, "Légende"=w214:string)
        n62 = call-poly <userlib>:"Append Text polymorphic.vi"("PDF Report"=w202, "Text [ ]"="Texte D2 [ ]", "error in (no error)"=w199) -> ("PDF Report duplicate"=w220:refnum<class "PDF Report Class.lvclass">, "error out"=w219:errorcluster)  [unwired: 1 in, 10 out]
        n63 = call <userlib>:"Update path.vi"("Path IN"=w209) -> ("Path OUT"=w210:path)  [unwired: 1 in, 2 out]
        n64 = call <userlib>:"Append Image File.vi"("PDF Report IN"=w220, "Image path"=w210, "error in (no error)"=w219, "Caption"=w214) -> ("PDF Report OUT"=w203:refnum<class "PDF Report Class.lvclass">, "error out"=w206:errorcluster)  [unwired: 3 in, 7 out]
        n65 = call <userlib>:"Append Chapter bookmark.vi"("PDF Report"=w203, "Chapter or section"=Chapter."Chapter - level 1", "Title"="Text E1", "error in (no error)"=w206) -> ("PDF Report duplicate"=w204:refnum<class "PDF Report Class.lvclass">, "error out"=w205:errorcluster)  [unwired: 10 in]
        n66 = call-poly <userlib>:"Append Text polymorphic.vi"("PDF Report"=w204, "Text [ ]"="Texte E2 [ ]", "error in (no error)"=w205) -> ("PDF Report duplicate"=w217:refnum<class "PDF Report Class.lvclass">, "error out"=w216:errorcluster)  [unwired: 2 in, 9 out]
        n67 = Unbundle("Image E1") -> ("Nom"=w208:path, "Légende"=w213:string)
        n68 = call <userlib>:"Update path.vi"("Path IN"=w208) -> ("Path OUT"=w207:path)  [unwired: 1 in, 2 out]
        n69 = call <userlib>:"Append Image File.vi"("PDF Report IN"=w217, "Scale (%)"=w212, "Image path"=w207, "error in (no error)"=w216, "Caption"=w213) -> ("PDF Report OUT"=w191:refnum<class "PDF Report Class.lvclass">, "error out"=w192:errorcluster)  [unwired: 2 in, 7 out]
        n70 = call <userlib>:"Append Chapter bookmark.vi"("PDF Report"=w191, "Chapter or section"=Chapter."Chapter - level 1", "Title"="Text F1", "error in (no error)"=w192, "Title properties"=T7 {" Aligment"=enum."LEFT", "Line spacing"=enum."1.5"}) -> ("PDF Report duplicate"=w190:refnum<class "PDF Report Class.lvclass">, "error out"=w189:errorcluster)  [unwired: 9 in]
        n71 = call <userlib>:"Append Chapter bookmark.vi"("PDF Report"=w190, "Chapter or section"=Chapter."Chapter - level 2", "Title"="Text F2", "error in (no error)"=w189) -> ("PDF Report duplicate"=w169:refnum<class "PDF Report Class.lvclass">, "error out"=w168:errorcluster)  [unwired: 10 in]
        n72 = call-poly <userlib>:"Append Text polymorphic.vi"("PDF Report"=w169, "Text [ ]"="Texte F3 [ ]", "error in (no error)"=w168) -> ("PDF Report duplicate"=w175:refnum<class "PDF Report Class.lvclass">, "error out"=w174:errorcluster)  [unwired: 2 in, 9 out]
        n73 = call <userlib>:"Update path [ ].vi"("Image to Add IN [ ]"="Image to Add [ ]") -> ("Image to Add OUT [ ]"=w180:T44)  [unwired: 1 in, 2 out]
        n74 = call <userlib>:"Create Table.vi"("PDF Report IN"=w175, "Table columnWidth [ ]"="Table columnWidth [ ] - Table 1", "Column Headers 2D [ ]"="Column Headers 2D [ ] - Table 1", "Text Data 2D [ ]"="Text Data 2D [ ] - Table 1", "error in (no error)"=w174, "Image to Add [ ]"=w180) -> ("PDF Report duplicate"=w183:refnum<class "PDF Report Class.lvclass">, "PDF Table"=w181:refnum<class "Pdfp Table Class.lvclass">, "error out"=w182:errorcluster)  [unwired: 7 in]
        n75 = call <userlib>:"Append Table.vi"("PDF Report IN"=w183, "Predefined Borders"="Predefined Borders Table 1", "Table properties"="Table properties 1)", "PDF Table"=w181, "Caption"="Caption 1", "error in (no error)"=w182, "Row Header format"="Datas properties 1", "Custom Table Borders"="Custom Table Borders 1") -> ("PDF Report OUT"=w166:refnum<class "PDF Report Class.lvclass">, "error out"=w167:errorcluster)  [unwired: 3 in, 3 out]
        n76 = call <userlib>:"Append New Page.vi"("PDF Report"=w166, "error in (no error)"=w167) -> ("PDF Report duplicate"=w165:refnum<class "PDF Report Class.lvclass">, "error OUT"=w164:errorcluster)  [unwired: 12 out]
      }
      frame 5 {
        w234 = sgl 40.0  # Scale (%)
        w246 = sgl 50.0  # Scale (%)
        w260 = sgl 55.0  # Scale (%)
        # "F) Chapter 5, section 5.1 - Text palette"
        n77 = Unbundle("Image F1") -> ("Nom"=w229:path, "Légende"=w228:string)
        n78 = call-poly <userlib>:"Append Text polymorphic.vi"("PDF Report"=w224, "Text"="Text F4", "error in (no error)"=w223) -> ("PDF Report duplicate"=w233:refnum<class "PDF Report Class.lvclass">, "error out"=w232:errorcluster)  [unwired: 5 in, 6 out]
        n79 = call <userlib>:"Update path.vi"("Path IN"=w229) -> ("Path OUT"=w230:path)  [unwired: 1 in, 2 out]
        n80 = call <userlib>:"Append Image File.vi"("PDF Report IN"=w233, "Scale (%)"=w234, "Image path"=w230, "error in (no error)"=w232, "Caption"=w228) -> ("PDF Report OUT"=w225:refnum<class "PDF Report Class.lvclass">, "error out"=w226:errorcluster)  [unwired: 2 in, 7 out]
        n81 = Unbundle("Image F2") -> ("Nom"=w251:path, "Légende"=w252:string)
        n82 = Unbundle("Image F3") -> ("Nom"=w240:path, "Légende"=w243:string)
        n83 = call-poly <userlib>:"Append Text polymorphic.vi"("PDF Report"=w225, "Text"="Text F5", "error in (no error)"=w226) -> ("PDF Report duplicate"=w247:refnum<class "PDF Report Class.lvclass">, "error out"=w248:errorcluster)  [unwired: 5 in, 6 out]
        n84 = call <userlib>:"Update path.vi"("Path IN"=w251) -> ("Path OUT"=w250:path)  [unwired: 1 in, 2 out]
        n85 = call <userlib>:"Update path.vi"("Path IN"=w240) -> ("Path OUT"=w239:path)  [unwired: 1 in, 2 out]
        n86 = call <userlib>:"Append Image File.vi"("PDF Report IN"=w247, "Scale (%)"=w246, "Image path"=w250, "error in (no error)"=w248, "Caption"=w252) -> ("PDF Report OUT"=w238:refnum<class "PDF Report Class.lvclass">, "error out"=w237:errorcluster)  [unwired: 2 in, 7 out]
        n87 = call-poly <userlib>:"Append Text polymorphic.vi"("PDF Report"=w238, "Text"="Text F6", "error in (no error)"=w237) -> ("PDF Report duplicate"=w241:refnum<class "PDF Report Class.lvclass">, "error out"=w242:errorcluster)  [unwired: 5 in, 6 out]
        n88 = Unbundle("Image F4") -> ("Nom"=w264:path, "Légende"=w261:string)
        n89 = call <userlib>:"Update path.vi"("Path IN"=w264) -> ("Path OUT"=w262:path)  [unwired: 1 in, 2 out]
        n90 = call <userlib>:"Append Image File.vi"("PDF Report IN"=w241, "Scale (%)"=sgl 60.0, "Image path"=w239, "error in (no error)"=w242, "Caption"=w243) -> ("PDF Report OUT"=w235:refnum<class "PDF Report Class.lvclass">, "error out"=w236:errorcluster)  [unwired: 2 in, 7 out]
        n91 = call <userlib>:"Append Image File.vi"("PDF Report IN"=w235, "Scale (%)"=w260, "Image path"=w262, "error in (no error)"=w236, "Caption"=w261) -> ("PDF Report OUT"=w265:refnum<class "PDF Report Class.lvclass">, "error out"=w266:errorcluster)  [unwired: 2 in, 7 out]
        n92 = local read "Image to Add [ ]"() -> (w273:T44)
        n93 = call-poly <userlib>:"Append Text polymorphic.vi"("PDF Report"=w265, "Text"="Text F7", "error in (no error)"=w266) -> ("PDF Report duplicate"=w255:refnum<class "PDF Report Class.lvclass">, "error out"=w254:errorcluster)  [unwired: 5 in, 6 out]
        n94 = call <userlib>:"Update path [ ].vi"("Image to Add IN [ ]"=w273) -> ("Image to Add OUT [ ]"=w272:T44)  [unwired: 1 in, 2 out]
        n95 = call-poly <userlib>:"Append Text polymorphic.vi"("PDF Report"=w255, "Text [ ]"="Text F8 [ ]", "error in (no error)"=w254, "Image to Add [ ]"=w272) -> ("PDF Report duplicate"=w256:refnum<class "PDF Report Class.lvclass">, "error out"=w259:errorcluster)  [unwired: 10 out]
        n96 = call <userlib>:"Set Page Size.vi"("PDF Report IN"=w256, "Page setup"=T2 {"Page Size"=1, "Orientation"=enum."Landscape", "Custom Size"={"Width"=0.0, "Height"=0.0}, "Margins"={"Left"=1.0, "Right"=1.0, "Top"=1.0, "Bottom"=1.0}} ("Page seup"), "error in (no error)"=w259) -> ("PDF Report OUT"=w257:refnum<class "PDF Report Class.lvclass">, "error OUT"=w258:errorcluster)  [unwired: 11 out]
        n97 = Unbundle("Image F5") -> ("Nom"=w270:path, "Légende"=w275:string)
        n98 = call <userlib>:"Update path.vi"("Path IN"=w270) -> ("Path OUT"=w269:path)  [unwired: 1 in, 2 out]
        n99 = call <userlib>:"Append Image File.vi"("PDF Report IN"=w257, "Image path"=w269, "error in (no error)"=w258, "Caption"=w275) -> ("PDF Report OUT"=w267:refnum<class "PDF Report Class.lvclass">, "error out"=w268:errorcluster)  [unwired: 3 in, 7 out]
        n100 = call <userlib>:"Set Page Size.vi"("PDF Report IN"=w267, "Page setup"=T2 {"Page Size"=1, "Orientation"=enum."Portrait", "Custom Size"={"Width"=0.0, "Height"=0.0}, "Margins"={"Left"=1.0, "Right"=1.0, "Top"=1.0, "Bottom"=1.0}} ("Page seup"), "error in (no error)"=w268) -> ("PDF Report OUT"=w280:refnum<class "PDF Report Class.lvclass">, "error OUT"=w279:errorcluster)  [unwired: 11 out]
      }
      frame 6 {
        w313 = sgl 55.0  # Scale (%)
        # "Append block diagram\nimage"
        # "Append front panel\nimage"
        # "G) Chapter 5, section 5.2 -  Image palette"
        n101 = call <userlib>:"Append Chapter bookmark.vi"("PDF Report"=w282, "Chapter or section"=Chapter."Chapter - level 2", "Title"="Text G1", "error in (no error)"=w281) -> ("PDF Report duplicate"=w283:refnum<class "PDF Report Class.lvclass">, "error out"=w284:errorcluster)  [unwired: 10 in]
        n102 = call-poly <userlib>:"Append Text polymorphic.vi"("PDF Report"=w283, "Text [ ]"="Texte G2 [ ]", "error in (no error)"=w284) -> ("PDF Report duplicate"=w300:refnum<class "PDF Report Class.lvclass">, "error out"=w299:errorcluster)  [unwired: 2 in, 9 out]
        n103 = Unbundle("Image G1") -> ("Nom"=w320:path, "Légende"=w314:string)
        n104 = call <userlib>:"Update path.vi"("Path IN"=w320) -> ("Path OUT"=w321:path)  [unwired: 1 in, 2 out]
        n105 = call <userlib>:"Append Image File.vi"("PDF Report IN"=w300, "Scale (%)"=w313, "Image path"=w321, "error in (no error)"=w299, "Caption"=w314) -> ("PDF Report OUT"=w301:refnum<class "PDF Report Class.lvclass">, "error out"=w302:errorcluster)  [unwired: 2 in, 7 out]
        n106 = Unbundle By Name("Cluster of images controls") -> ("Border"=w309:T39, "Scale (%)"=w310:sgl, "Position"=w312:T37)
        n107 = call-poly <userlib>:"Append Text polymorphic.vi"("PDF Report"=w301, "Text [ ]"="Texte G3 [ ]", "error in (no error)"=w302) -> ("PDF Report duplicate"=w307:refnum<class "PDF Report Class.lvclass">, "error out"=w303:errorcluster)  [unwired: 2 in, 9 out]
        n108 = control-ref of="Cluster of images controls"() -> (w311:refnum<vi>)
        n109 = call <userlib>:"Append Control Image.vi"("PDF Report IN"=w307, "Scale (%)"=w310, "Border"=w309, "Ctrl reference"=w311, "error in (no error)"=w303, "Position and indentation"=w312) -> ("PDF Report OUT"=w304:refnum<class "PDF Report Class.lvclass">, "error out"=w305:errorcluster)  [unwired: 1 in, 7 out]
        n110 = call-poly <userlib>:"Append Text polymorphic.vi"("PDF Report"=w304, "Text"="Text G4", "error in (no error)"=w305) -> ("PDF Report duplicate"=w319:refnum<class "PDF Report Class.lvclass">, "error out"=w318:errorcluster)  [unwired: 5 in, 6 out]
        n111 = call <userlib>:"Set Page Size.vi"("PDF Report IN"=w319, "Page setup"=T2 {"Page Size"=1, "Orientation"=enum."Landscape", "Custom Size"={"Width"=0.0, "Height"=0.0}, "Margins"={"Left"=1.0, "Right"=1.0, "Top"=1.0, "Bottom"=1.0}} ("Page seup"), "error in (no error)"=w318) -> ("PDF Report OUT"=w323:refnum<class "PDF Report Class.lvclass">, "error OUT"=w322:errorcluster)  [unwired: 11 out]
        n112 = control-ref of="This VI"() -> (w292:refnum<vi>)
        n113 = call <userlib>:"Append Front Panel Image.vi"("PDF Report IN"=w323, "VI reference"=w292, "error in (no error)"=w322, "Caption"="Image G2") -> ("PDF Report OUT"=w293:refnum<class "PDF Report Class.lvclass">, "error out"=w294:errorcluster)  [unwired: 4 in, 6 out]
        n114 = case shown="True" "Add block diagram" {
          tunnel: w293 -> [w325 w332]
          tunnel: w294 -> [w324 w331]
          tunnel: [w324 w328] -> w289
          tunnel: [w325 w327] -> w290
          tunnel: w292 -> [_ w330]
          tunnel: "Image G3" -> [_ w329]
          frame False {
          }
          frame True {
            w326 = T66 {"Maximum Width"=2500, "Maximum Height"=2500}  # Max Image size
            n115 = call <userlib>:"Append Block Diagram Image.vi"("PDF Report IN"=w332, "Image size"=w326, "VI reference"=w330, "error in (no error)"=w331, "Caption"=w329) -> ("PDF Report OUT"=w327:refnum<class "PDF Report Class.lvclass">, "error out"=w328:errorcluster)  [unwired: 9 in]
          }
        }
        n116 = call <userlib>:"Set Page Size.vi"("PDF Report IN"=w290, "Page setup"=T2 {"Page Size"=1, "Orientation"=enum."Portrait", "Custom Size"={"Width"=0.0, "Height"=0.0}, "Margins"={"Left"=1.0, "Right"=1.0, "Top"=1.0, "Bottom"=1.0}} ("Page seup"), "error in (no error)"=w289) -> ("PDF Report OUT"=w287:refnum<class "PDF Report Class.lvclass">, "error OUT"=w288:errorcluster)  [unwired: 11 out]
      }
      frame 7 {
        w361 = sgl 45.0  # Scale (%)
        w368 = sgl 28.0  # Scale (%)
        w369 = sgl 55.0  # Scale (%)
        w370 = sgl 45.0  # Scale (%)
        # "H) Chapter 5, section 5.3 - Table palette"
        n117 = call <userlib>:"Append Chapter bookmark.vi"("PDF Report"=w343, "Chapter or section"=Chapter."Chapter - level 2", "Title"="Text H1", "error in (no error)"=w344) -> ("PDF Report duplicate"=w346:refnum<class "PDF Report Class.lvclass">, "error out"=w345:errorcluster)  [unwired: 10 in]
        n118 = call-poly <userlib>:"Append Text polymorphic.vi"("PDF Report"=w346, "Text [ ]"="Texte H2 [ ]", "error in (no error)"=w345) -> ("PDF Report duplicate"=w378:refnum<class "PDF Report Class.lvclass">, "error out"=w379:errorcluster)  [unwired: 2 in, 9 out]
        n119 = Unbundle("Image H1") -> ("Nom"=w384:path, "Légende"=w381:string)
        n120 = call <userlib>:"Update path.vi"("Path IN"=w384) -> ("Path OUT"=w387:path)  [unwired: 1 in, 2 out]
        n121 = Unbundle("Image H2") -> ("Nom"=w360:path, "Légende"=w358:string)
        n122 = call <userlib>:"Update path.vi"("Path IN"=w360) -> ("Path OUT"=w359:path)  [unwired: 1 in, 2 out]
        n123 = call <userlib>:"Append Image File.vi"("PDF Report IN"=w378, "Scale (%)"=w369, "Image path"=w387, "error in (no error)"=w379, "Caption"=w381) -> ("PDF Report OUT"=w364:refnum<class "PDF Report Class.lvclass">, "error out"=w363:errorcluster)  [unwired: 2 in, 7 out]
        n124 = Unbundle("Image H3") -> ("Nom"=w367:path, "Légende"=w366:string)
        n125 = call <userlib>:"Append LF.vi"("PDF Report IN"=w364, "error in (no error)"=w363) -> ("PDF Report duplicate"=w356:refnum<class "PDF Report Class.lvclass">, "error out"=w355:errorcluster)  [unwired: 12 in]
        n126 = call <userlib>:"Update path.vi"("Path IN"=w367) -> ("Path OUT"=w362:path)  [unwired: 1 in, 2 out]
        n127 = call <userlib>:"Append Image File.vi"("PDF Report IN"=w356, "Image path"=w359, "error in (no error)"=w355, "Caption"=w358) -> ("PDF Report OUT"=w353:refnum<class "PDF Report Class.lvclass">, "error out"=w354:errorcluster)  [unwired: 3 in, 7 out]
        n128 = call <userlib>:"Append Image File.vi"("PDF Report IN"=w353, "Scale (%)"=w361, "Image path"=w362, "error in (no error)"=w354, "Caption"=w366) -> ("PDF Report OUT"=w349:refnum<class "PDF Report Class.lvclass">, "error out"=w350:errorcluster)  [unwired: 2 in, 7 out]
        n129 = call-poly <userlib>:"Append Text polymorphic.vi"("PDF Report"=w349, "Text"="Text H3", "error in (no error)"=w350) -> ("PDF Report duplicate"=w352:refnum<class "PDF Report Class.lvclass">, "error out"=w351:errorcluster)  [unwired: 5 in, 6 out]
        n130 = call-poly <userlib>:"Append Text polymorphic.vi"("PDF Report"=w352, "Text [ ]"="Texte H4 [ ]", "error in (no error)"=w351) -> ("PDF Report duplicate"=w336:refnum<class "PDF Report Class.lvclass">, "error out"=w335:errorcluster)  [unwired: 1 in, 10 out]
        n131 = Unbundle("Image H4") -> ("Nom"=w338:path, "Légende"=w339:string)
        n132 = call <userlib>:"Update path.vi"("Path IN"=w338) -> ("Path OUT"=w337:path)  [unwired: 1 in, 2 out]
        n133 = call <userlib>:"Append Image File.vi"("PDF Report IN"=w336, "Image path"=w337, "error in (no error)"=w335, "Caption"=w339) -> ("PDF Report OUT"=w333:refnum<class "PDF Report Class.lvclass">, "error out"=w334:errorcluster)  [unwired: 3 in, 7 out]
        n134 = Unbundle("Image H5") -> ("Nom"=w385:path, "Légende"=w382:string)
        n135 = call <userlib>:"Update path.vi"("Path IN"=w385) -> ("Path OUT"=w386:path)  [unwired: 1 in, 2 out]
        n136 = call <userlib>:"Append Image File.vi"("PDF Report IN"=w333, "Scale (%)"=w370, "Image path"=w386, "error in (no error)"=w334, "Caption"=w382) -> ("PDF Report OUT"=w375:refnum<class "PDF Report Class.lvclass">, "error out"=w374:errorcluster)  [unwired: 2 in, 7 out]
        n137 = Unbundle("Image H6") -> ("Nom"=w391:path, "Légende"=w389:string)
        n138 = call-poly <userlib>:"Append Text polymorphic.vi"("PDF Report"=w375, "Text"="Text H5", "error in (no error)"=w374) -> ("PDF Report duplicate"=w371:refnum<class "PDF Report Class.lvclass">, "error out"=w372:errorcluster)  [unwired: 5 in, 6 out]
        n139 = call <userlib>:"Update path.vi"("Path IN"=w391) -> ("Path OUT"=w392:path)  [unwired: 1 in, 2 out]
        n140 = call <userlib>:"Append Image File.vi"("PDF Report IN"=w371, "Scale (%)"=w368, "Image path"=w392, "error in (no error)"=w372, "Caption"=w389) -> ("PDF Report OUT"=w341:refnum<class "PDF Report Class.lvclass">, "error out"=w342:errorcluster)  [unwired: 2 in, 7 out]
      }
      frame 8 {
        w401 = sgl 50.0  # Scale (%)
        w411 = sgl 50.0  # Scale (%)
        w437 = sgl 60.0  # Scale (%)
        w441 = sgl 60.0  # Scale (%)
        # "H) Chapter 5, section 5.3 - Table palette"
        n141 = Unbundle("Image H7") -> ("Nom"=w394:path, "Légende"=w414:string)
        n142 = call <userlib>:"Update path.vi"("Path IN"=w394) -> ("Path OUT"=w393:path)  [unwired: 1 in, 2 out]
        n143 = call-poly <userlib>:"Append Text polymorphic.vi"("PDF Report"=w396, "Text"="Text H6", "error in (no error)"=w395) -> ("PDF Report duplicate"=w413:refnum<class "PDF Report Class.lvclass">, "error out"=w412:errorcluster)  [unwired: 5 in, 6 out]
        n144 = local read "Image to Add [ ]"() -> (w405:T44)
        n145 = call <userlib>:"Append Image File.vi"("PDF Report IN"=w413, "Scale (%)"=w411, "Image path"=w393, "error in (no error)"=w412, "Caption"=w414) -> ("PDF Report OUT"=w400:refnum<class "PDF Report Class.lvclass">, "error out"=w399:errorcluster)  [unwired: 2 in, 7 out]
        n146 = call <userlib>:"Update path [ ].vi"("Image to Add IN [ ]"=w405) -> ("Image to Add OUT [ ]"=w406:T44)  [unwired: 1 in, 2 out]
        n147 = call-poly <userlib>:"Append Text polymorphic.vi"("PDF Report"=w400, "Text [ ]"="Text H7 [ ]", "error in (no error)"=w399, "Image to Add [ ]"=w406) -> ("PDF Report duplicate"=w402:refnum<class "PDF Report Class.lvclass">, "error out"=w403:errorcluster)  [unwired: 10 out]
        n148 = Unbundle("Image H8") -> ("Nom"=w407:path, "Légende"=w409:string)
        n149 = call <userlib>:"Update path.vi"("Path IN"=w407) -> ("Path OUT"=w408:path)  [unwired: 1 in, 2 out]
        n150 = call <userlib>:"Append Image File.vi"("PDF Report IN"=w402, "Scale (%)"=w401, "Image path"=w408, "error in (no error)"=w403, "Caption"=w409) -> ("PDF Report OUT"=w397:refnum<class "PDF Report Class.lvclass">, "error out"=w398:errorcluster)  [unwired: 2 in, 7 out]
        n151 = call-poly <userlib>:"Append Text polymorphic.vi"("PDF Report"=w397, "Text"="Text H8", "error in (no error)"=w398) -> ("PDF Report duplicate"=w421:refnum<class "PDF Report Class.lvclass">, "error out"=w420:errorcluster)  [unwired: 5 in, 6 out]
        n152 = Unbundle("Image H9") -> ("Nom"=w434:path, "Légende"=w436:string)
        n153 = call <userlib>:"Update path.vi"("Path IN"=w434) -> ("Path OUT"=w435:path)  [unwired: 1 in, 2 out]
        n154 = Unbundle("Image H10") -> ("Nom"=w429:path, "Légende"=w431:string)
        n155 = call <userlib>:"Append Image File.vi"("PDF Report IN"=w421, "Scale (%)"=w437, "Image path"=w435, "error in (no error)"=w420, "Caption"=w436) -> ("PDF Report OUT"=w426:refnum<class "PDF Report Class.lvclass">, "error out"=w427:errorcluster)  [unwired: 2 in, 7 out]
        n156 = call <userlib>:"Update path.vi"("Path IN"=w429) -> ("Path OUT"=w430:path)  [unwired: 1 in, 2 out]
        n157 = call <userlib>:"Append Image File.vi"("PDF Report IN"=w426, "Image path"=w430, "error in (no error)"=w427, "Caption"=w431) -> ("PDF Report OUT"=w425:refnum<class "PDF Report Class.lvclass">, "error out"=w418:errorcluster)  [unwired: 3 in, 7 out]
        n158 = Unbundle("Image H11") -> ("Nom"=w438:path, "Légende"=w440:string)
        n159 = call <userlib>:"Update path.vi"("Path IN"=w438) -> ("Path OUT"=w439:path)  [unwired: 1 in, 2 out]
        n160 = call <userlib>:"Append New Page.vi"("PDF Report"=w425, "error in (no error)"=w418) -> ("PDF Report duplicate"=w419:refnum<class "PDF Report Class.lvclass">, "error OUT"=w417:errorcluster)  [unwired: 12 in]
        n161 = call <userlib>:"Append Image File.vi"("PDF Report IN"=w419, "Scale (%)"=w441, "Image path"=w439, "error in (no error)"=w417, "Caption"=w440) -> ("PDF Report OUT"=w424:refnum<class "PDF Report Class.lvclass">, "error out"=w423:errorcluster)  [unwired: 2 in, 7 out]
      }
      frame 9 {
        # "H) Chapter 5, section 5.3 - Table palette"
        # "Table 4"
        # "Table 3"
        # "Table 2"
        n162 = call <userlib>:"Create Table.vi"("PDF Report IN"=w445, "Column Headers 2D [ ]"="Column Headers 2D [ ] - Tables 2 to 4", "Text Data 2D [ ]"="Text Data 2D [ ]  - Tables 2 to 4", "error in (no error)"=w444) -> ("PDF Report duplicate"=w470:refnum<class "PDF Report Class.lvclass">, "PDF Table"=w471:refnum<class "Pdfp Table Class.lvclass">, "error out"=w472:errorcluster)  [unwired: 9 in]
        n163 = call <userlib>:"Append Table.vi"("PDF Report IN"=w470, "Table properties"="Table properties  - Tables 2 to 4", "PDF Table"=w471, "Caption"="Caption - Table 2", "error in (no error)"=w472) -> ("PDF Report OUT"=w477:refnum<class "PDF Report Class.lvclass">, "error out"=w478:errorcluster)  [unwired: 7 in, 2 out]
        n164 = call <userlib>:"Create Table.vi"("PDF Report IN"=w477, "Table columnWidth [ ]"="Table columnWidth [ ]  - Tables 3 and 4", "Column Headers 2D [ ]"="Column Headers 2D [ ] - Tables 2 to 4", "Text Data 2D [ ]"="Text Data 2D [ ]  - Tables 2 to 4", "error in (no error)"=w478) -> ("PDF Report duplicate"=w476:refnum<class "PDF Report Class.lvclass">, "PDF Table"=w473:refnum<class "Pdfp Table Class.lvclass">, "error out"=w475:errorcluster)  [unwired: 8 in]
        n165 = call <userlib>:"Append Table.vi"("PDF Report IN"=w476, "Table properties"="Table properties  - Tables 2 to 4", "PDF Table"=w473, "Caption"="Caption - Table 3", "error in (no error)"=w475) -> ("PDF Report OUT"=w480:refnum<class "PDF Report Class.lvclass">, "error out"=w479:errorcluster)  [unwired: 7 in, 2 out]
        n166 = call <userlib>:"Append New Page.vi"("PDF Report"=w480, "error in (no error)"=w479) -> ("PDF Report duplicate"=w455:refnum<class "PDF Report Class.lvclass">, "error OUT"=w454:errorcluster)  [unwired: 12 out]
        n167 = Unbundle("Image H12") -> ("Nom"=w462:path, "Légende"=w467:string)
        n168 = call <userlib>:"Update path.vi"("Path IN"=w462) -> ("Path OUT"=w466:path)  [unwired: 1 in, 2 out]
        n169 = call <userlib>:"Append Image File.vi"("PDF Report IN"=w455, "Scale (%)"=sgl 60.0, "Image path"=w466, "error in (no error)"=w454, "Caption"=w467) -> ("PDF Report OUT"=w465:refnum<class "PDF Report Class.lvclass">, "error out"=w468:errorcluster)  [unwired: 2 in, 7 out]
        n170 = call <userlib>:"Create Table.vi"("PDF Report IN"=w465, "Table columnWidth [ ]"="Table columnWidth [ ]  - Tables 3 and 4", "Column Headers 2D [ ]"="Column Headers 2D [ ] - Tables 2 to 4", "Text Data 2D [ ]"="Text Data 2D [ ]  - Tables 2 to 4", "error in (no error)"=w468) -> ("PDF Report duplicate"=w458:refnum<class "PDF Report Class.lvclass">, "PDF Table"=w457:refnum<class "Pdfp Table Class.lvclass">, "error out"=w456:errorcluster)  [unwired: 8 in]
        n171 = call <userlib>:"Append Table.vi"("PDF Report IN"=w458, "Column Header format"="Column Header format - Table 4", "Predefined Borders"="Predefined Borders - Table 4", "Row background color"="Row background color - Table 4", "Table properties"="Table properties  - Tables 2 to 4", "PDF Table"=w457, "Caption"="Caption - Table 4", "error in (no error)"=w456, "Datas format"="Datas format - Table 4") -> ("PDF Report OUT"=w446:refnum<class "PDF Report Class.lvclass">, "error out"=w447:errorcluster)  [unwired: 3 in, 2 out]
        n172 = call <userlib>:"Append New Page.vi"("PDF Report"=w446, "error in (no error)"=w447) -> ("PDF Report duplicate"=w443:refnum<class "PDF Report Class.lvclass">, "error OUT"=w442:errorcluster)  [unwired: 12 out]
      }
      frame 10 {
        # "H) Chapter 5, section 5.3 - Table palette"
        # "Table 5"
        n173 = Unbundle("Image H13") -> ("Nom"=w485:path, "Légende"=w489:string)
        n174 = call <userlib>:"Update path.vi"("Path IN"=w485) -> ("Path OUT"=w488:path)  [unwired: 1 in, 2 out]
        n175 = call <userlib>:"Append Image File.vi"("PDF Report IN"=w481, "Scale (%)"=sgl 60.0, "Image path"=w488, "error in (no error)"=w482, "Caption"=w489) -> ("PDF Report OUT"=w483:refnum<class "PDF Report Class.lvclass">, "error out"=w484:errorcluster)  [unwired: 2 in, 7 out]
        n176 = call <userlib>:"Create Table.vi"("PDF Report IN"=w483, "Table columnWidth [ ]"="Table columnWidth [ ] - Table 5", "Column Headers 2D [ ]"="Column Headers 2D [ ] - Table 5", "Row Headers 1D [ ]"="Row Headers 1D [ ] - Table 5", "Text Data 2D [ ]"="Text Data 2D [ ] - Table 5", "error in (no error)"=w484) -> ("PDF Report duplicate"=w500:refnum<class "PDF Report Class.lvclass">, "PDF Table"=w497:refnum<class "Pdfp Table Class.lvclass">, "error out"=w501:errorcluster)  [unwired: 7 in]
        n177 = call <userlib>:"Append Customized Table.vi"("PDF Report IN"=w500, "Table properties"="Table properties - Table 5", "PDF Table"=w497, "Caption"="Caption - Table 5", "error in (no error)"=w501, "Row  [ ]"="Row  [ ] - Table 5") -> ("PDF Report OUT"=w491:refnum<class "PDF Report Class.lvclass">, "error out"=w490:errorcluster)  [unwired: 8 in]
        n178 = call <userlib>:"Append New Page.vi"("PDF Report"=w491, "error in (no error)"=w490) -> ("PDF Report duplicate"=w503:refnum<class "PDF Report Class.lvclass">, "error OUT"=w502:errorcluster)  [unwired: 12 out]
      }
      frame 11 {
        w527 = sgl 100.0  # Scale (%)
        w552 = sgl 48.0  # Scale (%)
        # "Table 6"
        # "I) Chapter 5, section 5.4 Document palette"
        n179 = call <userlib>:"Append Chapter bookmark.vi"("PDF Report"=w504, "Chapter or section"=Chapter."Chapter - level 2", "Title"="Text I1", "error in (no error)"=w505) -> ("PDF Report duplicate"=w507:refnum<class "PDF Report Class.lvclass">, "error out"=w506:errorcluster)  [unwired: 10 in]
        n180 = call-poly <userlib>:"Append Text polymorphic.vi"("PDF Report"=w507, "Text [ ]"="Texte I2 [ ]", "error in (no error)"=w506) -> ("PDF Report duplicate"=w542:refnum<class "PDF Report Class.lvclass">, "error out"=w543:errorcluster)  [unwired: 2 in, 9 out]
        n181 = Unbundle("Image I1") -> ("Nom"=w558:path, "Légende"=w554:string)
        n182 = call <userlib>:"Update path.vi"("Path IN"=w558) -> ("Path OUT"=w561:path)  [unwired: 1 in, 2 out]
        n183 = call <userlib>:"Append Image File.vi"("PDF Report IN"=w542, "Scale (%)"=w552, "Image path"=w561, "error in (no error)"=w543, "Caption"=w554) -> ("PDF Report OUT"=w545:refnum<class "PDF Report Class.lvclass">, "error out"=w546:errorcluster)  [unwired: 2 in, 7 out]
        n184 = call-poly <userlib>:"Append Text polymorphic.vi"("PDF Report"=w545, "Text [ ]"="Texte I3 [ ]", "error in (no error)"=w546) -> ("PDF Report duplicate"=w548:refnum<class "PDF Report Class.lvclass">, "error out"=w547:errorcluster)  [unwired: 2 in, 9 out]
        n185 = Unbundle("Image I2") -> ("Nom"=w559:path, "Légende"=w553:string)
        n186 = Unbundle("Image I3") -> ("Nom"=w560:path, "Légende"=w555:string)
        n187 = call <userlib>:"Update path.vi"("Path IN"=w559) -> ("Path OUT"=w562:path)  [unwired: 1 in, 2 out]
        n188 = call <userlib>:"Update path.vi"("Path IN"=w560) -> ("Path OUT"=w563:path)  [unwired: 1 in, 2 out]
        n189 = call <userlib>:"Append Image File.vi"("PDF Report IN"=w548, "Scale (%)"=w552, "Image path"=w562, "error in (no error)"=w547, "Caption"=w553) -> ("PDF Report OUT"=w540:refnum<class "PDF Report Class.lvclass">, "error out"=w541:errorcluster)  [unwired: 2 in, 7 out]
        n190 = call <userlib>:"Append Image File.vi"("PDF Report IN"=w540, "Scale (%)"=w552, "Image path"=w563, "error in (no error)"=w541, "Caption"=w555) -> ("PDF Report OUT"=w519:refnum<class "PDF Report Class.lvclass">, "error out"=w518:errorcluster)  [unwired: 2 in, 7 out]
        n191 = Unbundle("Image I4") -> ("Nom"=w529:path, "Légende"=w528:string)
        n192 = call <userlib>:"Update path.vi"("Path IN"=w529) -> ("Path OUT"=w530:path)  [unwired: 1 in, 2 out]
        n193 = call-poly <userlib>:"Append Text polymorphic.vi"("PDF Report"=w519, "Text"="Texte I4", "error in (no error)"=w518) -> ("PDF Report duplicate"=w524:refnum<class "PDF Report Class.lvclass">, "error out"=w525:errorcluster)  [unwired: 5 in, 6 out]
        n194 = call <userlib>:"Append Image File.vi"("PDF Report IN"=w524, "Scale (%)"=w527, "Image path"=w530, "error in (no error)"=w525, "Caption"=w528) -> ("PDF Report OUT"=w522:refnum<class "PDF Report Class.lvclass">, "error out"=w521:errorcluster)  [unwired: 2 in, 7 out]
        n195 = call-poly <userlib>:"Append Text polymorphic.vi"("PDF Report"=w522, "Text"="Texte I5", "error in (no error)"=w521) -> ("PDF Report duplicate"=w520:refnum<class "PDF Report Class.lvclass">, "error out"=w513:errorcluster)  [unwired: 5 in, 6 out]
        n196 = call <userlib>:"Append New Page.vi"("PDF Report"=w520, "error in (no error)"=w513) -> ("PDF Report duplicate"=w514:refnum<class "PDF Report Class.lvclass">, "error OUT"=w512:errorcluster)  [unwired: 12 in]
        n197 = call <userlib>:"Create Table.vi"("PDF Report IN"=w514, "Table columnWidth [ ]"="Table columnWidth [ ] - table 6", "Column Headers 2D [ ]"="Column Headers 2D [ ] - table 6", "Row Headers 1D [ ]"="Row Headers 1D [ ] - table 6", "Text Data 2D [ ]"="Text Data 2D [ ] - table 6", "error in (no error)"=w512) -> ("PDF Report duplicate"=w538:refnum<class "PDF Report Class.lvclass">, "PDF Table"=w534:refnum<class "Pdfp Table Class.lvclass">, "error out"=w539:errorcluster)  [unwired: 7 in]
        n198 = call <userlib>:"Append Customized Table.vi"("PDF Report IN"=w538, "PDF Table"=w534, "Caption"="Caption - table 6", "error in (no error)"=w539, "Row  [ ]"="Row  [ ] - table 6") -> ("PDF Report OUT"=w516:refnum<class "PDF Report Class.lvclass">, "error out"=w515:errorcluster)  [unwired: 9 in]
        n199 = call-poly <userlib>:"Append Text polymorphic.vi"("PDF Report"=w516, "Text [ ]"="Texte I6 [ ]", "error in (no error)"=w515) -> ("PDF Report duplicate"=w510:refnum<class "PDF Report Class.lvclass">, "error out"=w511:errorcluster)  [unwired: 2 in, 9 out]
      }
      frame 12 {
        w595 = sgl 50.0  # Scale (%)
        # "J) Chapter 5, section 5.5 - Header, Footer and Watermark palette"
        n200 = call <userlib>:"Append Chapter bookmark.vi"("PDF Report"=w564, "Chapter or section"=Chapter."Chapter - level 2", "Title"="Text J1", "error in (no error)"=w565) -> ("PDF Report duplicate"=w567:refnum<class "PDF Report Class.lvclass">, "error out"=w566:errorcluster)  [unwired: 10 in]
        n201 = call-poly <userlib>:"Append Text polymorphic.vi"("PDF Report"=w567, "Text [ ]"="Texte J2 [ ]", "error in (no error)"=w566) -> ("PDF Report duplicate"=w594:refnum<class "PDF Report Class.lvclass">, "error out"=w593:errorcluster)  [unwired: 2 in, 9 out]
        n202 = Unbundle("Image J1") -> ("Nom"=w604:path, "Légende"=w596:string)
        n203 = Unbundle("Image J2") -> ("Nom"=w603:path, "Légende"=w597:string)
        n204 = Unbundle("Image J3") -> ("Nom"=w621:path, "Légende"=w598:string)
        n205 = Unbundle("Image J4") -> ("Nom"=w605:path, "Légende"=w599:string)
        n206 = call <userlib>:"Update path.vi"("Path IN"=w604) -> ("Path OUT"=w606:path)  [unwired: 1 in, 2 out]
        n207 = call <userlib>:"Update path.vi"("Path IN"=w603) -> ("Path OUT"=w607:path)  [unwired: 1 in, 2 out]
        n208 = call <userlib>:"Update path.vi"("Path IN"=w621) -> ("Path OUT"=w622:path)  [unwired: 1 in, 2 out]
        n209 = call <userlib>:"Update path.vi"("Path IN"=w605) -> ("Path OUT"=w608:path)  [unwired: 1 in, 2 out]
        n210 = call <userlib>:"Append Image File.vi"("PDF Report IN"=w594, "Scale (%)"=w595, "Image path"=w606, "error in (no error)"=w593, "Caption"=w596) -> ("PDF Report OUT"=w579:refnum<class "PDF Report Class.lvclass">, "error out"=w578:errorcluster)  [unwired: 2 in, 7 out]
        n211 = call-poly <userlib>:"Append Text polymorphic.vi"("PDF Report"=w579, "Text"="Texte J3", "error in (no error)"=w578) -> ("PDF Report duplicate"=w576:refnum<class "PDF Report Class.lvclass">, "error out"=w577:errorcluster)  [unwired: 5 in, 6 out]
        n212 = call <userlib>:"Append Image File.vi"("PDF Report IN"=w576, "Scale (%)"=w595, "Image path"=w607, "error in (no error)"=w577, "Caption"=w597) -> ("PDF Report OUT"=w632:refnum<class "PDF Report Class.lvclass">, "error out"=w631:errorcluster)  [unwired: 2 in, 7 out]
        n213 = call <userlib>:"Append Image File.vi"("PDF Report IN"=w632, "Scale (%)"=w595, "Image path"=w622, "error in (no error)"=w631, "Caption"=w598) -> ("PDF Report OUT"=w588:refnum<class "PDF Report Class.lvclass">, "error out"=w587:errorcluster)  [unwired: 2 in, 7 out]
        n214 = call-poly <userlib>:"Append Text polymorphic.vi"("PDF Report"=w588, "Text [ ]"="Texte J4 [ ]", "error in (no error)"=w587) -> ("PDF Report duplicate"=w582:refnum<class "PDF Report Class.lvclass">, "error out"=w581:errorcluster)  [unwired: 2 in, 9 out]
        n215 = call <userlib>:"Append Image File.vi"("PDF Report IN"=w582, "Image path"=w608, "error in (no error)"=w581, "Caption"=w599) -> ("PDF Report OUT"=w584:refnum<class "PDF Report Class.lvclass">, "error out"=w583:errorcluster)  [unwired: 3 in, 7 out]
        n216 = call-poly <userlib>:"Append Text polymorphic.vi"("PDF Report"=w584, "Text [ ]"="Texte J5 [ ]", "error in (no error)"=w583) -> ("PDF Report duplicate"=w585:refnum<class "PDF Report Class.lvclass">, "error out"=w586:errorcluster)  [unwired: 2 in, 9 out]
        n217 = Unbundle("Image J5") -> ("Nom"=w609:path, "Légende"=w618:string)
        n218 = Unbundle("Image J6") -> ("Nom"=w610:path, "Légende"=w619:string)
        n219 = Unbundle("Image J7") -> ("Nom"=w612:path, "Légende"=w620:string)
        n220 = Unbundle("Image J8") -> ("Nom"=w625:path, "Légende"=w628:string)
        n221 = call <userlib>:"Update path.vi"("Path IN"=w609) -> ("Path OUT"=w615:path)  [unwired: 1 in, 2 out]
        n222 = call <userlib>:"Update path.vi"("Path IN"=w610) -> ("Path OUT"=w616:path)  [unwired: 1 in, 2 out]
        n223 = call <userlib>:"Update path.vi"("Path IN"=w612) -> ("Path OUT"=w617:path)  [unwired: 1 in, 2 out]
        n224 = call <userlib>:"Update path.vi"("Path IN"=w625) -> ("Path OUT"=w627:path)  [unwired: 1 in, 2 out]
        n225 = call <userlib>:"Append Image File.vi"("PDF Report IN"=w585, "Image path"=w615, "error in (no error)"=w586, "Caption"=w618) -> ("PDF Report OUT"=w573:refnum<class "PDF Report Class.lvclass">, "error out"=w572:errorcluster)  [unwired: 3 in, 7 out]
        n226 = call <userlib>:"Append Image File.vi"("PDF Report IN"=w573, "Image path"=w616, "error in (no error)"=w572, "Caption"=w619) -> ("PDF Report OUT"=w575:refnum<class "PDF Report Class.lvclass">, "error out"=w574:errorcluster)  [unwired: 3 in, 7 out]
        n227 = call <userlib>:"Append Image File.vi"("PDF Report IN"=w575, "Image path"=w617, "error in (no error)"=w574, "Caption"=w620) -> ("PDF Report OUT"=w623:refnum<class "PDF Report Class.lvclass">, "error out"=w624:errorcluster)  [unwired: 3 in, 7 out]
        n228 = call <userlib>:"Append Image File.vi"("PDF Report IN"=w623, "Image path"=w627, "error in (no error)"=w624, "Caption"=w628) -> ("PDF Report OUT"=w629:refnum<class "PDF Report Class.lvclass">, "error out"=w630:errorcluster)  [unwired: 3 in, 7 out]
        n229 = call <userlib>:"Append New Page.vi"("PDF Report"=w629, "error in (no error)"=w630) -> ("PDF Report duplicate"=w571:refnum<class "PDF Report Class.lvclass">, "error OUT"=w570:errorcluster)  [unwired: 12 out]
      }
      frame 13 {
        w647 = sgl 50.0  # Scale (%)
        # "J) Chapter 5, section 5.5 - Header, Footer and Watermark palette"
        # "Ajout d'images provenant de contrôles."
        # "Gras et italique"
        n230 = call-poly <userlib>:"Append Text polymorphic.vi"("PDF Report"=w652, "Text [ ]"="Texte J6 [ ]", "error in (no error)"=w651) -> ("PDF Report duplicate"=w637:refnum<class "PDF Report Class.lvclass">, "error out"=w636:errorcluster)  [unwired: 2 in, 9 out]
        n231 = control-ref of="Watermark Image"() -> (w635:refnum<vi>)
        n232 = call <userlib>:"Append Control Image.vi"("PDF Report IN"=w637, "Scale (%)"=w647, "Ctrl reference"=w635, "error in (no error)"=w636, "Caption"="Image J9") -> ("PDF Report OUT"=w642:refnum<class "PDF Report Class.lvclass">, "error out"=w643:errorcluster)  [unwired: 2 in, 7 out]
        n233 = control-ref of="Watermark Text"() -> (w648:refnum<vi>)
        n234 = call <userlib>:"Append Control Image.vi"("PDF Report IN"=w642, "Scale (%)"=w647, "Ctrl reference"=w648, "error in (no error)"=w643, "Caption"="Image J10") -> ("PDF Report OUT"=w645:refnum<class "PDF Report Class.lvclass">, "error out"=w644:errorcluster)  [unwired: 2 in, 7 out]
        n235 = call-poly <userlib>:"Append Text polymorphic.vi"("PDF Report"=w645, "Text"="TexteJ7", "error in (no error)"=w644, "Font"=T11 {"Name"="", "Size"=-1.0, "Color"=0, "Style"={"Bold"=TRUE, "Italic"=TRUE, "Underline"=FALSE, "Strikeout"=FALSE}, "Type"={"Type&direction"=enum."Select", "Embedded"=FALSE, "Encoding"=""}} ("Font complete")) -> ("PDF Report duplicate"=w634:refnum<class "PDF Report Class.lvclass">, "error out"=w633:errorcluster)  [unwired: 4 in, 6 out]
        n236 = call <userlib>:"Append New Page.vi"("PDF Report"=w634, "error in (no error)"=w633) -> ("PDF Report duplicate"=w649:refnum<class "PDF Report Class.lvclass">, "error OUT"=w650:errorcluster)  [unwired: 12 in]
      }
      frame 14 {
        w667 = sgl 55.0  # Scale (%)
        # "K) Chapter 5, section 5.6 - Concatenate palette"
        n237 = call <userlib>:"Append Chapter bookmark.vi"("PDF Report"=w653, "Chapter or section"=Chapter."Chapter - level 2", "Title"="Text k1", "error in (no error)"=w654) -> ("PDF Report duplicate"=w655:refnum<class "PDF Report Class.lvclass">, "error out"=w656:errorcluster)  [unwired: 10 in]
        n238 = call-poly <userlib>:"Append Text polymorphic.vi"("PDF Report"=w655, "Text [ ]"="Texte K2 [ ]", "error in (no error)"=w656) -> ("PDF Report duplicate"=w673:refnum<class "PDF Report Class.lvclass">, "error out"=w672:errorcluster)  [unwired: 2 in, 9 out]
        n239 = Unbundle("Image K1") -> ("Nom"=w676:path, "Légende"=w674:string)
        n240 = call <userlib>:"Update path.vi"("Path IN"=w676) -> ("Path OUT"=w677:path)  [unwired: 1 in, 2 out]
        n241 = call <userlib>:"Append Image File.vi"("PDF Report IN"=w673, "Scale (%)"=w667, "Image path"=w677, "error in (no error)"=w672, "Caption"=w674) -> ("PDF Report OUT"=w669:refnum<class "PDF Report Class.lvclass">, "error out"=w670:errorcluster)  [unwired: 2 in, 7 out]
        n242 = control-ref of="PDF Files  to concatenate and pages"() -> (w668:refnum<vi>)
        n243 = call <userlib>:"Append Control Image.vi"("PDF Report IN"=w669, "Scale (%)"=w667, "Ctrl reference"=w668, "error in (no error)"=w670, "Caption"="Image K2") -> ("PDF Report OUT"=w660:refnum<class "PDF Report Class.lvclass">, "error out"=w661:errorcluster)  [unwired: 9 in]
        n244 = call-poly <userlib>:"Append Text polymorphic.vi"("PDF Report"=w660, "Text [ ]"="Texte K3 [ ]", "error in (no error)"=w661) -> ("PDF Report duplicate"=w663:refnum<class "PDF Report Class.lvclass">, "error out"=w662:errorcluster)  [unwired: 2 in, 9 out]
        n245 = call <userlib>:"Append New Page.vi"("PDF Report"=w663, "error in (no error)"=w662) -> ("PDF Report duplicate"=w666:refnum<class "PDF Report Class.lvclass">, "error OUT"=w665:errorcluster)  [unwired: 12 in]
      }
      frame 15 {
        w681 = sgl 45.0  # Scale (%)
        w692 = sgl 35.0  # Scale (%)
        w714 = sgl 55.0  # Scale (%)
        # "L) Chapter 5, section 5.7 - Table of Contents palette"
        n246 = call <userlib>:"Append Chapter bookmark.vi"("PDF Report"=w719, "Chapter or section"=Chapter."Chapter - level 2", "Title"="Text L1", "error in (no error)"=w718) -> ("PDF Report duplicate"=w713:refnum<class "PDF Report Class.lvclass">, "error out"=w703:errorcluster)  [unwired: 10 in]
        n247 = call-poly <userlib>:"Append Text polymorphic.vi"("PDF Report IN"=w713, "Text"="Text L2", "error in (no error)"=w703) -> ("PDF Report OUT"=w711:refnum<class "PDF Report Class.lvclass">, "error out"=w702:errorcluster)  [unwired: 11 in]
        n248 = Unbundle("Image L1") -> ("Nom"=w716:path, "Légende"=w715:string)
        n249 = Unbundle("Image L3") -> ("Nom"=w696:path, "Légende"=w693:string)
        n250 = Unbundle("Image L2") -> ("Nom"=w707:path, "Légende"=w708:string)
        n251 = Unbundle("Image L4") -> ("Nom"=w684:path, "Légende"=w682:string)
        n252 = call <userlib>:"Update path.vi"("Path IN"=w716) -> ("Path OUT"=w717:path)  [unwired: 1 in, 2 out]
        n253 = call <userlib>:"Update path.vi"("Path IN"=w696) -> ("Path OUT"=w694:path)  [unwired: 1 in, 2 out]
        n254 = call <userlib>:"Update path.vi"("Path IN"=w707) -> ("Path OUT"=w706:path)  [unwired: 1 in, 2 out]
        n255 = call <userlib>:"Update path.vi"("Path IN"=w684) -> ("Path OUT"=w683:path)  [unwired: 1 in, 2 out]
        n256 = call <userlib>:"Append Image File.vi"("PDF Report IN"=w711, "Scale (%)"=w714, "Image path"=w717, "error in (no error)"=w702, "Caption"=w715) -> ("PDF Report OUT"=w705:refnum<class "PDF Report Class.lvclass">, "error out"=w704:errorcluster)  [unwired: 2 in, 7 out]
        n257 = call <userlib>:"Append Image File.vi"("PDF Report IN"=w705, "Scale (%)"=w681, "Image path"=w706, "error in (no error)"=w704, "Caption"=w708) -> ("PDF Report OUT"=w700:refnum<class "PDF Report Class.lvclass">, "error out"=w699:errorcluster)  [unwired: 2 in, 7 out]
        n258 = call-poly <userlib>:"Append Text polymorphic.vi"("PDF Report IN"=w700, "Text"="Text L3", "error in (no error)"=w699) -> ("PDF Report OUT"=w697:refnum<class "PDF Report Class.lvclass">, "error out"=w698:errorcluster)  [unwired: 11 in]
        n259 = call <userlib>:"Append Image File.vi"("PDF Report IN"=w697, "Scale (%)"=w692, "Image path"=w694, "error in (no error)"=w698, "Caption"=w693) -> ("PDF Report OUT"=w689:refnum<class "PDF Report Class.lvclass">, "error out"=w690:errorcluster)  [unwired: 2 in, 7 out]
        n260 = call-poly <userlib>:"Append Text polymorphic.vi"("PDF Report IN"=w689, "Text"="Text L4", "error in (no error)"=w690) -> ("PDF Report OUT"=w687:refnum<class "PDF Report Class.lvclass">, "error out"=w688:errorcluster)  [unwired: 11 in]
        n261 = call <userlib>:"Append Image File.vi"("PDF Report IN"=w687, "Scale (%)"=w681, "Image path"=w683, "error in (no error)"=w688, "Caption"=w682) -> ("PDF Report OUT"=w686:refnum<class "PDF Report Class.lvclass">, "error out"=w679:errorcluster)  [unwired: 2 in, 7 out]
        n262 = call <userlib>:"Append New Page.vi"("PDF Report"=w686, "error in (no error)"=w679) -> ("PDF Report duplicate"=w680:refnum<class "PDF Report Class.lvclass">, "error OUT"=w678:errorcluster)  [unwired: 12 in]
      }
      frame 16 {
        w732 = sgl 55.0  # Scale (%)
        # "M) Chapter 5, section 5.8 - Tools palette"
        n263 = call <userlib>:"Append Chapter bookmark.vi"("PDF Report"=w727, "Chapter or section"=Chapter."Chapter - level 2", "Title"="Text M1", "error in (no error)"=w728) -> ("PDF Report duplicate"=w730:refnum<class "PDF Report Class.lvclass">, "error out"=w731:errorcluster)  [unwired: 10 in]
        n264 = Unbundle("Image M1") -> ("Nom"=w734:path, "Légende"=w733:string)
        n265 = call <userlib>:"Update path.vi"("Path IN"=w734) -> ("Path OUT"=w735:path)  [unwired: 1 in, 2 out]
        n266 = call <userlib>:"Append Image File.vi"("PDF Report IN"=w730, "Scale (%)"=w732, "Image path"=w735, "error in (no error)"=w731, "Caption"=w733) -> ("PDF Report OUT"=w726:refnum<class "PDF Report Class.lvclass">, "error out"=w724:errorcluster)  [unwired: 2 in, 7 out]
        n267 = call-poly <userlib>:"Append Text polymorphic.vi"("PDF Report"=w726, "Text"="Text M2", "error in (no error)"=w724) -> ("PDF Report duplicate"=w725:refnum<class "PDF Report Class.lvclass">, "error out"=w723:errorcluster)  [unwired: 11 in]
      }
      frame 17 {
        w759 = sgl 60.0  # Scale (%)
        w773 = sgl 35.0  # Scale (%)
        w785 = sgl 33.0  # Scale (%)
        w791 = sgl 23.0  # Scale (%)
        # "N) Chapter 6 - Unicode with PDF Report"
        n268 = call <userlib>:"Append Chapter bookmark.vi"("PDF Report"=w751, "Chapter or section"=Chapter."Chapter - level 1", "Title"="Text N1", "error in (no error)"=w750, "Font"="Font N1") -> ("PDF Report duplicate"=w744:refnum<class "PDF Report Class.lvclass">, "error out"=w743:errorcluster)  [unwired: 9 in]
        n269 = call-poly <userlib>:"Append Text polymorphic.vi"("PDF Report"=w744, "Text"="Text N2", "Font"=T11 {"Name"="", "Size"=-1.0, "Color"=0, "Style"={"Bold"=FALSE, "Italic"=TRUE, "Underline"=FALSE, "Strikeout"=FALSE}, "Type"={"Type&direction"=enum."Select", "Embedded"=FALSE, "Encoding"=""}}) -> ("PDF Report duplicate"=w740:refnum<class "PDF Report Class.lvclass">)  [unwired: 11 in, 1 out]
        n270 = call <userlib>:"Append Chapter bookmark.vi"("PDF Report"=w740, "Chapter or section"=Chapter."Chapter - level 2", "Title"="Text N3", "error in (no error)"=w743) -> ("PDF Report duplicate"=w745:refnum<class "PDF Report Class.lvclass">, "error out"=w746:errorcluster)  [unwired: 10 in]
        n271 = call-poly <userlib>:"Append Text polymorphic.vi"("PDF Report"=w745, "Text [ ]"="Texte N4 [ ]", "error in (no error)"=w746) -> ("PDF Report duplicate"=w788:refnum<class "PDF Report Class.lvclass">, "error out"=w789:errorcluster)  [unwired: 2 in, 9 out]
        n272 = Unbundle("Image N1") -> ("Nom"=w793:path, "Légende"=w792:string)
        n273 = call <userlib>:"Update path.vi"("Path IN"=w793) -> ("Path OUT"=w794:path)  [unwired: 1 in, 2 out]
        n274 = call <userlib>:"Append Image File.vi"("PDF Report IN"=w788, "Scale (%)"=w791, "Image path"=w794, "error in (no error)"=w789, "Caption"=w792) -> ("PDF Report OUT"=w779:refnum<class "PDF Report Class.lvclass">, "error out"=w780:errorcluster)  [unwired: 2 in, 7 out]
        n275 = Unbundle("Image N2") -> ("Nom"=w783:path, "Légende"=w784:string)
        n276 = call-poly <userlib>:"Append Text polymorphic.vi"("PDF Report"=w779, "Text"="Text N5", "error in (no error)"=w780) -> ("PDF Report duplicate"=w778:refnum<class "PDF Report Class.lvclass">, "error out"=w777:errorcluster)  [unwired: 5 in, 6 out]
        n277 = call <userlib>:"Update path.vi"("Path IN"=w783) -> ("Path OUT"=w782:path)  [unwired: 1 in, 2 out]
        n278 = call <userlib>:"Append Image File.vi"("PDF Report IN"=w778, "Scale (%)"=w785, "Image path"=w782, "error in (no error)"=w777, "Caption"=w784) -> ("PDF Report OUT"=w769:refnum<class "PDF Report Class.lvclass">, "error out"=w770:errorcluster)  [unwired: 2 in, 7 out]
        n279 = call-poly <userlib>:"Append Text polymorphic.vi"("PDF Report"=w769, "Text"="Text N6", "error in (no error)"=w770) -> ("PDF Report duplicate"=w767:refnum<class "PDF Report Class.lvclass">, "error out"=w768:errorcluster)  [unwired: 5 in, 6 out]
        n280 = Unbundle("Image N3") -> ("Nom"=w775:path, "Légende"=w774:string)
        n281 = call <userlib>:"Update path.vi"("Path IN"=w775) -> ("Path OUT"=w776:path)  [unwired: 1 in, 2 out]
        n282 = call <userlib>:"Append Image File.vi"("PDF Report IN"=w767, "Scale (%)"=w773, "Image path"=w776, "error in (no error)"=w768, "Caption"=w774) -> ("PDF Report OUT"=w765:refnum<class "PDF Report Class.lvclass">, "error out"=w766:errorcluster)  [unwired: 2 in, 7 out]
        n283 = call-poly <userlib>:"Append Text polymorphic.vi"("PDF Report"=w765, "Text"="Text N7", "error in (no error)"=w766) -> ("PDF Report duplicate"=w763:refnum<class "PDF Report Class.lvclass">, "error out"=w762:errorcluster)  [unwired: 5 in, 6 out]
        n284 = control-ref of="Text N9"() -> (w761:refnum<vi>)
        n285 = call <userlib>:"Append Control Image.vi"("PDF Report IN"=w763, "Scale (%)"=w759, "Ctrl reference"=w761, "error in (no error)"=w762, "Caption"="Image N4") -> ("PDF Report OUT"=w757:refnum<class "PDF Report Class.lvclass">, "error out"=w758:errorcluster)  [unwired: 9 in]
        n286 = call-poly <userlib>:"Append Text polymorphic.vi"("PDF Report"=w757, "Text"="Text N8", "error in (no error)"=w758) -> ("PDF Report duplicate"=w754:refnum<class "PDF Report Class.lvclass">, "error out"=w755:errorcluster)  [unwired: 5 in, 6 out]
        n287 = call-poly <userlib>:"Append Text polymorphic.vi"("PDF Report"=w754, "Text"="Text N9", "error in (no error)"=w755, "Font"="Font N1") -> ("PDF Report duplicate"=w747:refnum<class "PDF Report Class.lvclass">, "error out"=w748:errorcluster)  [unwired: 5 in, 5 out]
      }
      frame 18 {
        w833 = sgl 35.0  # Scale (%)
        n288 = Unbundle("Image N5") -> ("Nom"=w835:path, "Légende"=w834:string)
        n289 = call-poly <userlib>:"Append Text polymorphic.vi"("PDF Report"=w827, "Text"="Text N10", "error in (no error)"=w828) -> ("PDF Report duplicate"=w831:refnum<class "PDF Report Class.lvclass">, "error out"=w830:errorcluster)  [unwired: 5 in, 6 out]
        n290 = call <userlib>:"Update path.vi"("Path IN"=w835) -> ("Path OUT"=w829:path)  [unwired: 1 in, 2 out]
        n291 = call <userlib>:"Append Image File.vi"("PDF Report IN"=w831, "Scale (%)"=w833, "Image path"=w829, "error in (no error)"=w830, "Caption"=w834) -> ("PDF Report OUT"=w824:refnum<class "PDF Report Class.lvclass">, "error out"=w811:errorcluster)  [unwired: 2 in, 7 out]
        n292 = call <userlib>:"Append New Page.vi"("PDF Report"=w824, "error in (no error)"=w811) -> ("PDF Report duplicate"=w812:refnum<class "PDF Report Class.lvclass">, "error OUT"=w810:errorcluster)  [unwired: 12 in]
        n293 = call <userlib>:"Append Chapter bookmark.vi"("PDF Report"=w812, "Chapter or section"=Chapter."Chapter - level 2", "Title"="Text N11", "error in (no error)"=w810) -> ("PDF Report duplicate"=w814:refnum<class "PDF Report Class.lvclass">, "error out"=w813:errorcluster)  [unwired: 10 in]
        n294 = call <userlib>:"Create Table.vi"("PDF Report IN"=w814, "Table columnWidth [ ]"="Table columnWidth [ ] - Table 7", "Column Headers 2D [ ]"="Column Headers 2D [ ] - Table 7", "Row Headers 1D [ ]"="Row Headers 1D [ ] - Table 7", "Text Data 2D [ ]"="Text Data 2D [ ] - Table 7", "error in (no error)"=w813) -> ("PDF Report duplicate"=w822:refnum<class "PDF Report Class.lvclass">, "PDF Table"=w819:refnum<class "Pdfp Table Class.lvclass">, "error out"=w823:errorcluster)  [unwired: 7 in]
        n295 = call <userlib>:"Append Customized Table.vi"("PDF Report IN"=w822, "Table properties"="Table properties - Table 7", "PDF Table"=w819, "error in (no error)"=w823, "Row  [ ]"="Row  [ ] - Table 7") -> ("PDF Report OUT"=w801:refnum<class "PDF Report Class.lvclass">, "error out"=w800:errorcluster)  [unwired: 9 in]
        n296 = call <userlib>:"Append LF.vi"("PDF Report IN"=w801, "error in (no error)"=w800) -> ("PDF Report duplicate"=w798:refnum<class "PDF Report Class.lvclass">, "error out"=w799:errorcluster)  [unwired: 12 in]
        n297 = call <userlib>:"Create Table.vi"("PDF Report IN"=w798, "Table columnWidth [ ]"="Table columnWidth [ ] - Table 8", "Row Headers 1D [ ]"="Row Headers 1D [ ] - Table 8", "Text Data 2D [ ]"="Text Data 2D [ ] - Table 8", "error in (no error)"=w799) -> ("PDF Report duplicate"=w808:refnum<class "PDF Report Class.lvclass">, "PDF Table"=w806:refnum<class "Pdfp Table Class.lvclass">, "error out"=w809:errorcluster)  [unwired: 8 in]
        n298 = call <userlib>:"Append Customized Table.vi"("PDF Report IN"=w808, "Table properties"="Table properties - Table 8", "PDF Table"=w806, "error in (no error)"=w809, "Row  [ ]"="Row  [ ] - Table 8") -> ("PDF Report OUT"=w796:refnum<class "PDF Report Class.lvclass">, "error out"=w797:errorcluster)  [unwired: 9 in]
      }
      frame 19 {
        # "O) Chapter 7"
        n299 = call <userlib>:"Append Chapter bookmark.vi"("PDF Report"=w841, "Chapter or section"=Chapter."Chapter - level 1", "Title"="Text O1", "error in (no error)"=w840) -> ("PDF Report duplicate"=w842:refnum<class "PDF Report Class.lvclass">, "error out"=w843:errorcluster)  [unwired: 10 in]
        n300 = call-poly <userlib>:"Append Text polymorphic.vi"("PDF Report"=w842, "Text [ ]"="Text O2 [ ]", "error in (no error)"=w843) -> ("PDF Report duplicate"=w848:refnum<class "PDF Report Class.lvclass">, "error out"=w847:errorcluster)  [unwired: 2 in, 9 out]
        n301 = call <userlib>:"Append LF.vi"("PDF Report IN"=w848, "Number of LF (default 1)"=u8 3, "error in (no error)"=w847) -> ("PDF Report duplicate"=w844:refnum<class "PDF Report Class.lvclass">, "error out"=w845:errorcluster)  [unwired: 11 in]
        n302 = call <userlib>:"Append PDF file to PDF Report .vi"("PDF Report"=w844, "PDF Files  to concatenate and pages"="PDF Files  to concatenate and pages", "error in (no error)"=w845) -> ("PDF Report duplicate"=w851:refnum<class "PDF Report Class.lvclass">, "error out"=w850:errorcluster)  [unwired: 11 in]
      }
      frame 20 {
        # "It is here that are added the the Table of Contents, the headers, footers and watermark. Furthermore, it is here that are concatenated the PDF files."
        # "L) Closing PDF Report"
        n303 = call <userlib>:"Close PDF.vi"("PDF Report"=w852, "error in (no error)"=w853) -> ("Path"=→"PDF File Name":path, "error out"=w854:errorcluster)  [unwired: 12 out]
      }
      frame 21 {
      }
    }
    "Progress" <- w3
  }
  "error out" <- w2
